vi "SIcamera_Manager.vi"() -> ()   [LabVIEW 2015]
uses:
  SI_Client_Subvis/Client Acquisition Mode Menu.ctl
  SI_Client_Subvis/Frame Mode 1.ctl
  W:/GSCS/Systems/SystemUtil/Command.ctl
  W:/GSCS/Systems/SIcamera_Control/SI_Client_Subvis/CameraStates.ctl
  W:/GSCS/Systems/Cam_Focus/CF_drivercontrol.ctl
  W:/GSCS/Log/LogItem.ctl
  SIcamera_Globals.vi
  W:/GSCS/Systems/SIcamera_Control/GPS_Drivers/GPS_Driver_Global.vi
  W:/GSCS/Systems/TCS_Link/TCSLINK_global.vi
  Instance          36 24Saved   SIcamera_Manager .vi
  W:/GSCS/GUI/GSP_GUI_global.vi
  W:/GSCS/Systems/SIcamera_Control/Apogee_Global.vi
  W:/GSCS/Systems/Cam_Focus/GSP_CF_Global.vi
panel:
  out "Focus Changed?":bool
  out "Current Lamp Percent":string
  out "Current Lamp":string
  out "Has Red switch been run":bool
  out "Readout left":dbl format="%<%M:%S>t"
  out "Exp time left":dbl format="%<%M:%S >t"
  out "Fe Ind":u16(ring)
  out "Quartz Ind":u16(ring)
  out "Ar Ind":u16(ring)
  out "Hg(Ar) Ind":u16(ring)
  out "Cu Ind":u16(ring)
  out "Ne Ind":u16(ring)
  out "Bulb Ind":u16(ring)
  in  "CCD Readout Speed":u8(ring)=3 items=["750 kHz, ATTN 0", "750 kHz, ATTN 2", "344 kHz, ATTN 0", "344 kHz, ATTN 3", "100 kHz, ATTN 2", "100 kHz, ATTN 3"]
  in  "CCD ROI Mode":u16(ring)=10 items=["Imaging, 1x1  "=0, "Imaging, 2x2"=1, "Imaging, 3x3"=2, "Spectroscopic, 1x1"=3, "Spectroscopic, 2x2"=4, "Spectroscopic, 3x3"=5, "MOS, 1x1"=11, "MOS, 2x2"=12, "MOS, 3x3"=13, "Slicer"=6, "Spectroscopic, ZZ Ceti"=14, "Slit Imaging/Alignment"=7, "MOS Imaging/Alignment"=10, "Set user-defined ROI..."=8, "Custom Mode"=9, "Custom from Script"=21]
  in  "MOS":bool
  in  "Lamp Cluster":T1
  in  "Calculate Offset":bool
  in  "sy1":dbl
  in  "sx1":dbl
  in  "oy1":dbl
  in  "ox1":dbl
  in  "N/S Offset":dbl min=0.0 max=420.0 step=0.15 format="%03.2f"
  in  "N/S Offset Choice":u16(ring) items=["North", "South"]
  in  "E/W Offset Choice":u8(ring) items=["East", "West"]
  in  "E/W Offset":dbl min=0.0 max=420.0 step=0.15 format="%03.2f"
  in  "Offset Telescope":bool
  in  "Systems Status & Control":enum32{"Camera", "General"}(tab)
  in  "Camera Color":string(combo)="Red"
  in  "Get Camera Status":bool
  out "CCD Temp.":string
  out "Vacuum Pressure":string
  in  "Reset TCP":bool
  out "Connection Status":bool
  in  "Reset Wavelength Angles System":bool
  in  "Proposal #":string
  in  "Observer Name":string
  in  "Show Images?":bool
  out "Image File Name":string="0001.image.fits"
  in  "Image #":i32=1 min=1 step=1 format="%04.0f"
  out "Current Status":string
  in  "Exp. Time (s)":dbl=1.0 min=0.25 step=1.0 format="%.2f"
  in  "RO Done":bool
  out "Exposure":u16(slide) scale=0.0..100.0
  out "Readout":u16(slide) caption="% Readout" scale=0.0..100.0
  in  "File Name Base":string="image"
  in  "Start Exposure":bool
  in  "Exposure Tab":T2(tab)=enum."Zero"
  in  "# Exposures":i32=1 min=1 step=1
  in  "Object Comments:":string
  in  "Object Name:":string
  in  "Dome Set Percent":i32 caption="%"
  out "Dome Ind":u16(ring)
  out "Dome Percent":i8=70 caption="%" min=0 max=100 step=1
  in  "Dome":bool
  out "Quartz Actual":i8 caption="%"
  in  "Quartz Intensity":i8=70 caption="%" min=0 max=100 step=1
  in  "# Flat Exposures":i32=1 min=1 step=1
  in  "Flat Name:":string
  in  "# Comp Exposures":i32=1 min=1 step=1
  in  "Comp Comments:":string
  in  "Comp Name:":string
  out "Dark Name:":string="DARK"
  in  "Dark Comments:":string
  in  "# Dark Exposures":i32=1 min=1 step=1
  out "Zero Name:":string="ZERO"
  in  "Zero Comments:":string
  in  "# Zero Exposures":i32=1 min=1 step=1
  in  "Step Size":dbl
  in  "Focus Start":dbl
  in  "# Focus Steps":dbl
  in  "Focus Name":string
  in  "Control references":T3
  in  "?":bool
  in  "ROIMODE":string
  in  "Exp. Time (s) 2":dbl=1.0 min=0.5 step=1.0 format="%.1f"
  in  "Save As":u16(ring)=1 items=["U16 FITS", "I16 FITS", "I32 FITS", "SGL FITS", "U16 TIFF", "I16 TIFF", "I32 TIFF", "SGL TIFF"]
  in  "Port Readout":u16(ring)=2 items=["4-port", "Port A", "Port B", "Port C", "Port D"]
  out "Current File Name":string
  out "TCP/IP ID":refnum<k5>
  out "CCD ROI":cluster{i32, i32, i32, i32, i32, i32}={0, 4096, 1, 0, 4096, 1}
  out "Open Shutter During Image?":bool=TRUE
  out "Readout Time":dbl
  in  "Thumbnail Setting":enum16{"Check Entire CCD", "Check Star Focus"}(ring)
  in  "Take Thumbnail":bool
  in  "Save":bool
  in  "Frames":i32=1 min=1 step=1
  in  "Frame Mode":T4 items=["Single Frame Buffer", "Multiple Frame Buffer"]
  out "Packet\nError code":i32
  out "Function #":u16
  in  "# to Average":u32=2 caption="of"
  out "Error out":errorcluster
  out "Acquiring":u32
  out "P Len":i32
  out "S Len":i32
  in  "Mode":u16(ring)=4 items=["Retrieve Image Buffer", "Acquire and transfer to client", "Acquire and hold in Server Image Buffer", "Acquire, transfer to client, and save to Server's disk", "Acquire, save to Server's disk, and hold in Server Image Buffer"]
  in  "Acq Mode":T5 caption="Acquisition Mode"
  in  "SHUTDOWN":bool
  in  "Script":T6={"Exposure Time"=0.0, "#Exposures"=1, "Current Exposure"=2, "Last Exposure Start Time"=92278252, "Exposure type"=1, "Obs parameters"={"Object Name"="", "Telescope"="SOAR 4.1m", "Instrument"="Goodman Spectrograph", "Comment"="", "INSTCONF"="", "CAMSWV"="", "CONSWV"="", "INSTSWV"="", "CAMERA"=""}, "System Pos Info"={"Grating#"=0, "Slit#"=0, "Primary Filter#"=0, "Secondary Filter#"=0, "Coll Position"=1000, "Camera Focus"=-396, "Camera Angle"=12.21, "Grating Angle"=20.740599999999997, "Coll Temp"=0.0, "Cam Temp"=0.0, "Camera Target"=12.21, "Grating Target"=20.740599999999997, "WAVMODE"="", "Slit hidden?"=FALSE}, "TCSInfo"={"Mount Az"=0.0, "Mount El"=0.0, "RA"="", "DEC"="", "Hour Angle"="", "Airmass"=0.0, "Focus"=0.0, "Rotator Angle"=0.0, "Rotator Location"="", "Dome Shutter"="", "Dome Az"=0.0, "Date"="", "UT Time"="", "Sidereal Time"="", "Position Angle"=0.0, "Seeing"=0.0, "OBSRA"="", "OBSDEC"="", "Position ADC"="", "Position ADC 2"="", "Bulb"=FALSE, "Ar"=FALSE, "Cu"=FALSE, "Dome"=FALSE, "Fe"=FALSE, "Hg(Ar)"=FALSE, "Ne"=FALSE, "Quartz"=FALSE, "Dome Percent"=0.0, "Quartz Percent"=0.0}, "Exposure Active?"=FALSE, "Component Names"={"Slit Name"="<NO MASK>", "F1_Name"="<NO FILTER>", "F2_Name"="<NO FILTER>", "Grating Name"="<NO GRATING>"}, "Other Info."={"CCD Read Noise"=3.99, "CCD Gain"=2.06, "OBSTYPE"="OBJECT", "OBSERVER"="", "Proposal #"="", "Equinox"=2000.0}, "Reduction Info."={"DISPAXIS"=1, "DETSIZE"="[1:4096,1:4096]", "CCDSUM"="1 1", "DETSEC"="[1:4096,1:4096]", "DATASEC"="[1:4096,1:4096]"}, "EnvironmentalInfo"={"Outside Temp"=0.0, "Wind Direction"=0.0, "Wind Speed"=0.0, "Pressure"=0.0, "Humidity"=0.0}} {"Other Info."."Equinox" format="%#.2f"; "Other Info."."CCD Gain" format="%#.2g"; "Other Info."."CCD Read Noise" format="%#.2g"; "Exposure type" items=["Dark", "Light"]}
  out "Camera Errors":errorcluster
  in  "CommandQ":string
  # "x"
  # "y"
  # "Save As"
  # "I16 FITS"
  # "Current Pixel Values:"
  # "\" to the"
  # "Port Readout"
  # "\" to the"
  # "Desired Pixel Values:"
  # "Port B"
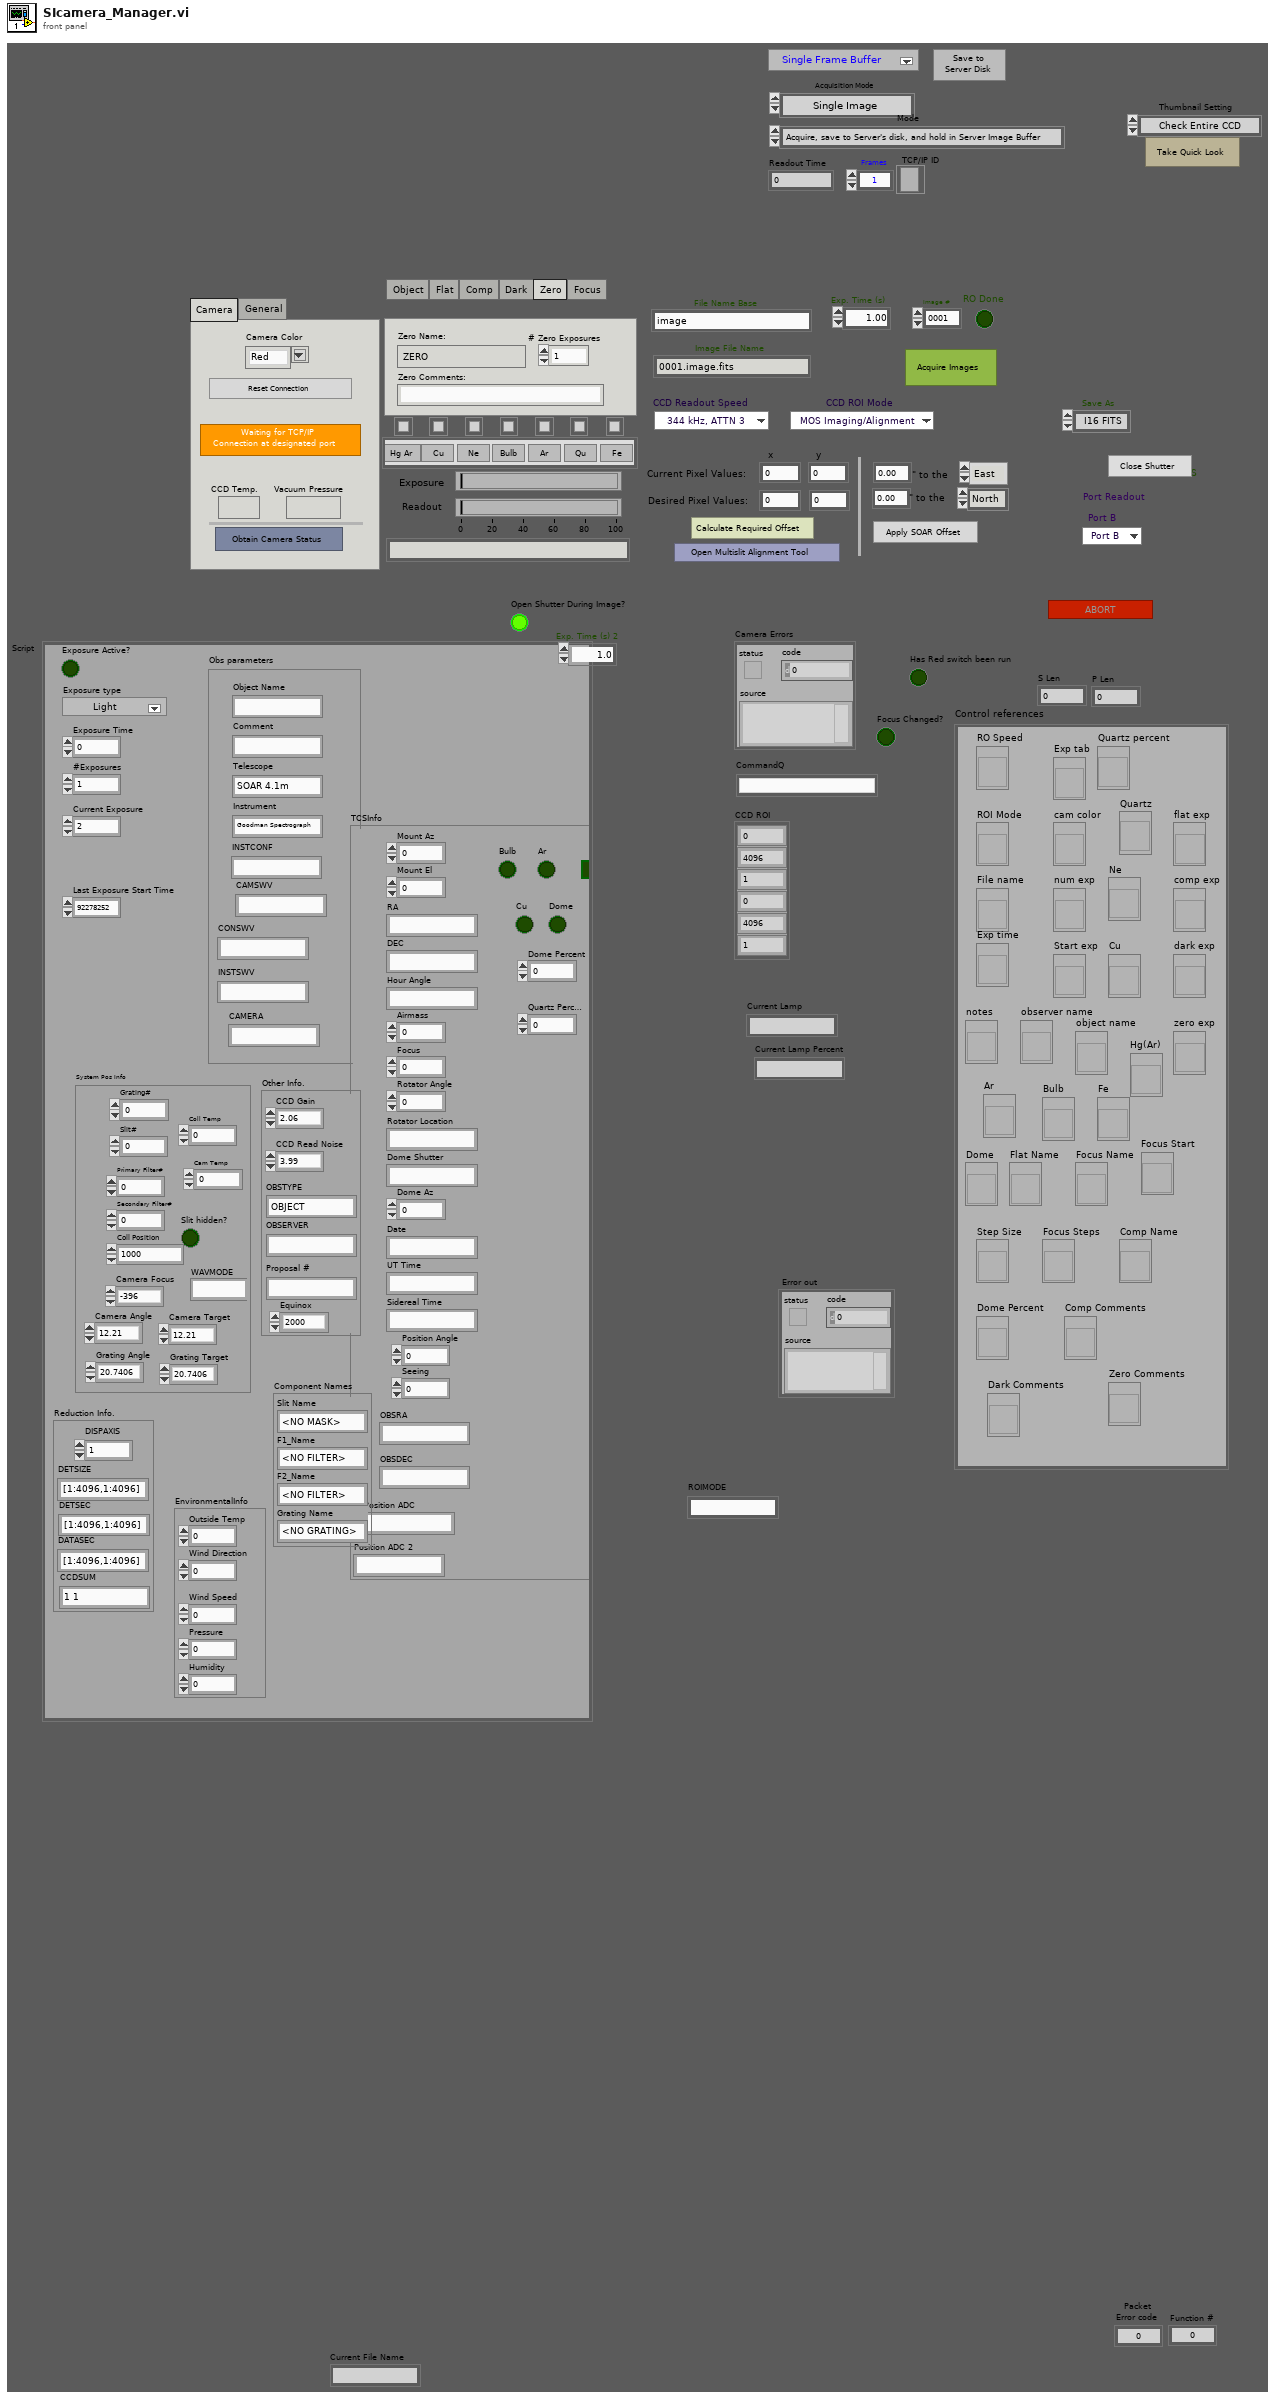
[diagram p1: front panel]
types:
  T1 = cluster{"Hg(Ar)":bool, "Cu":bool, "Ne":bool, "Ar":bool, "Quartz":bool, "Fe":bool, "Bulb":bool}
  T2 = enum32{"Object", "Flat", "Comp", "Dark", "Zero", "Focus"}
  T3 = cluster{"ROI Mode":refnum<vi>, "RO Speed":refnum<vi>, "File name":refnum<vi>, "Exp time":refnum<vi>, "Start exp":refnum<vi>, "num exp":refnum<vi>, "cam color":refnum<vi>, "Exp tab":refnum<vi>, "notes":refnum<vi>, "observer name":refnum<vi>, "object name":refnum<vi>, "Ar":refnum<vi>, "Bulb":refnum<vi>, "Fe":refnum<vi>, "Hg(Ar)":refnum<vi>, "Cu":refnum<vi>, "Ne":refnum<vi>, "Quartz":refnum<vi>, "Quartz percent":refnum<vi>, "flat exp":refnum<vi>, "comp exp":refnum<vi>, "dark exp":refnum<vi>, "zero exp":refnum<vi>, "Dome":refnum<vi>, "Flat Name":refnum<vi>, "Focus Name":refnum<vi>, "Focus Start":refnum<vi>, "Step Size":refnum<vi>, "Comp Name":refnum<vi>, "Comp Comments":refnum<vi>, "Focus Steps":refnum<vi>, "Dome Percent":refnum<vi>, "Dark Comments":refnum<vi>, "Zero Comments":refnum<vi>}
  T4 = typedef "Frame Mode 1.ctl" = i32
  T5 = typedef "Client Acquisition Mode Menu.ctl" = enum16{"Single Image", "Average Images", "Multiple Frames"}
  T6 = cluster{"Exposure Time":dbl, "#Exposures":i32, "Current Exposure":i32, "Last Exposure Start Time":u32, "Exposure type":i16, "Obs parameters":cluster{"Object Name":string, "Telescope":string, "Instrument":string, "Comment":string, "INSTCONF":string, "CAMSWV":string, "CONSWV":string, "INSTSWV":string, "CAMERA":string}, "System Pos Info":cluster{"Grating#":i32, "Slit#":i32, "Primary Filter#":i32, "Secondary Filter#":i32, "Coll Position":i32, "Camera Focus":i32, "Camera Angle":dbl, "Grating Angle":dbl, "Coll Temp":dbl, "Cam Temp":dbl, "Camera Target":dbl, "Grating Target":dbl, "WAVMODE":string, "Slit hidden?":bool}, "TCSInfo":cluster{"Mount Az":dbl, "Mount El":dbl, "RA":string, "DEC":string, "Hour Angle":string, "Airmass":dbl, "Focus":dbl, "Rotator Angle":dbl, "Rotator Location":string, "Dome Shutter":string, "Dome Az":dbl, "Date":string, "UT Time":string, "Sidereal Time":string, "Position Angle":dbl, "Seeing":dbl, "OBSRA":string, "OBSDEC":string, "Position ADC":string, "Position ADC 2":string, "Bulb":bool, "Ar":bool, "Cu":bool, "Dome":bool, "Fe":bool, "Hg(Ar)":bool, "Ne":bool, "Quartz":bool, "Dome Percent":dbl, "Quartz Percent":dbl}, "Exposure Active?":bool, "Component Names":cluster{"Slit Name":string, "F1_Name":string, "F2_Name":string, "Grating Name":string}, "Other Info.":cluster{"CCD Read Noise":dbl, "CCD Gain":dbl, "OBSTYPE":string, "OBSERVER":string, "Proposal #":string, "Equinox":dbl}, "Reduction Info.":cluster{"DISPAXIS":i8, "DETSIZE":string, "CCDSUM":string, "DETSEC":string, "DATASEC":string}, "EnvironmentalInfo":cluster{"Outside Temp":dbl, "Wind Direction":dbl, "Wind Speed":dbl, "Pressure":dbl, "Humidity":dbl}}
  T7 = typedef "Command.ctl" = cluster{"Command":string, "Parameter":string}
  T8 = cluster{"Object Name":string, "Telescope":string, "Instrument":string, "Comment":string, "\nINSTCONF":string, "CAMSWV":string, "CONSWV":string, "INSTSWV":string, "CAMERA":string}
  T9 = enum16{"POL (0)", "CPL (1)", "HLT (2)", "STP (3)", "RST (4)", "RVN (5)", "RPB (6)", "CLP (8)", "SDL (9)", "RUN (10)", "WRI (11)", "RRG (12)", "SPR (13)", "LPR (14)", "VMI (15)", "SSP (17)", "SSE (18)", "RIS (20)", "RIO (21)", "IMW (25)", "END (128)", "MAV (134)", "MRV (135)", "JRE (137)", "WCL (138)", "WCW (139)", "DLY (140)", "WDL (141)", "GCL (142)", "GOP (143)", "ZTG (144)", "ZTP (145)", "TTP (146)", "CME (147)", "CTC (148)", "TQL (149)", "AHC (150)", "ERL (151)", "OLP (152)", "WRP (154)", "IDT (155)", "LRP (156)", "VMP (159)", "RAV (160)", "RRV (161)", "JMP (162)", "JOI (162)", "CIS (163)", "CKS (164)", "CLC (165)", "KMC (167)", "MCT (168)", "FLC (169)", "EEM (170)", "DDB (171)", "DEM (171)", "PAC (172)", "ADL (173)", "BRT (174)", "MAT (176)", "MRT (177)", "RAT (178)", "RRT (179)", "SSD (180)", "KMR (181)", "KED (182)", "KDD (183)", "DIR (184)", "PRO (185)", "SIF (186)", "EDL (187)", "CIO (188)", "MDS (189)", "MDC (190)", "MDT (191)", "SEE (192)", "ARI (193)", "WBS (194)", "SCF (195)", "RSM (196)", "RLM (197)", "RSN (198)", "RLN (199)", "PCL (201)", "PCI (201)", "PRT (202)", "PRI (202)", "WBE (204)", "SOB (205)", "COB (206)", "ACR (207)", "PLR (208)", "CAI (211)", "LVT (212)", "OVT (213)", "MTT (214)", "CLC (215)", "PIM (216)", "VIM (217)", "TIM (218)", "AHM (219)", "SSL (221)", "TRU (222)", "RSD (223)", "EMT (225)", "DMT (226)", "EMD (227)", "DMD (228)", "HSM (229)", "AHD (230)", "PCM (231)", "PCG (232)", "XRV (233)", "XAV (234)", "XRT (235)", "XAT (236)", "GOC (237)", "JNA (238)", "JOR (239)", "PMC (240)", "PMV (241)", "PMX (242)", "DLC (243)", "SLC (244)", "PCP (245)", "ATR (248)", "PMO (249)", "JAN (250)", "EDH (251)", "DIF (252)", "IMS (253)", "IMQ (254)"}
  T10 = typedef "CameraStates.ctl" = enum16{"Ready", "Exposing", "Error"}
  T11 = typedef "CF_drivercontrol.ctl" = enum16{"Launch", "Move", "Set Piezos", "Flexure On", "Flexure Off", "Home", "Shutdown"}
  T12 = typedef "LogItem.ctl" = cluster{"error in (no error)":errorcluster, "Source":string, "Comment ":string}
  T13 = enum16{"Launch", "Log", "Open", "Close", "Shutdown"}
  T14 = cluster{"Serial Origin":i32, "Serial Length":i32, "Serial Binning":i32, "Parallel Origin":i32, "Parallel Length":i32, "Parallel Binning":i32}
  T15 = cluster{"Mount Az":dbl, "Mount El":dbl, "RA":string, "DEC":string, "Hour Angle":string, "Airmass":dbl, "Focus":dbl, "Rotator Angle":dbl, "Rotator Location":string, "Dome Shutter":string, "Dome Az":dbl, "Date":string, "UT Time":string, "Sidereal Time":string, "Position Angle":dbl, "Seeing":dbl, "OBSRA":string, "OBSDEC":string, "Position ADC":string, "Position ADC 2":string, "Bulb":bool, "Ar":bool, "Cu":bool, "Dome":bool, "Fe":bool, "Hg(Ar)":bool, "Ne":bool, "Quartz":bool, "Dome Percent":dbl, "Quartz Percent":dbl}
  T16 = cluster{"Grating#":i32, "Slit#":i32, "Primary Filter#":i32, "Secondary Filter#":i32, "Coll Position":i32, "Camera Focus":i32, "Camera Angle":dbl, "Grating Angle":dbl, "Coll Temp":dbl, "CF Temp\n":dbl, "Camera Target":dbl, "Grating Target":dbl, "WAVMODE":string, "Slit Hidden??":bool}
  T17 = cluster{"Slit Name":string, "F1_Name":string, "F2_Name":string, "Grating Name":string}
  T18 = cluster{"element":i32, "element":i32, "element":i32, "element":i32, "element":i32, "element":i32}
  T19 = cluster{"% Exp.":u16, "%Readout":u16, "Relative Pos.":u32, "Acquiring":i32}
  T20 = typedef "TCP-IP Image Packet.ctl" = cluster{"Image ID":u16, "Image Type":u16, "Serial Length":u16, "Parallel Length":u16, "# of Packets":u16, "Packet #":u16, "Offset":u32, "Image Bytes":u32, "Image Data $":string}
  T21 = cluster{"DISPAXIS":i8, "DETSIZE":string, "CCDSUM":string, "DETSEC":string, "DATASEC":string}
  T22 = cluster{"Object Name":string, "Telescope":string, "Instrument":string, "Comment":string, "INSTCONF":string, "CAMSWV":string, "CONSWV":string, "INSTSWV":string, "CAMERA":string}
  T23 = cluster{"CCD Read Noise":dbl, "CCD Gain":dbl, "OBSTYPE":string, "OBSERVER":string, "Proposal #":string, "Equinox":dbl}
  T24 = cluster{"Exp. Time (s)":dbl, "CCD Read Noise":dbl, "CCD Gain":dbl, "OBSTYPE":string, "OBSERVER":string, "Proposal #":string, "Equinox":dbl, "ROIMODE":string}
  T25 = cluster{"Outside Temp":dbl, "Wind Direction":dbl, "Wind Speed":dbl, "Pressure":dbl, "Humidity":dbl}
  T26 = typedef "ThreadStates.ctl" = enum16{"Waiting", "Scripting", "Uninitialized", "Error"}
  T27 = cluster{"Command":string, "Current File Name":string}
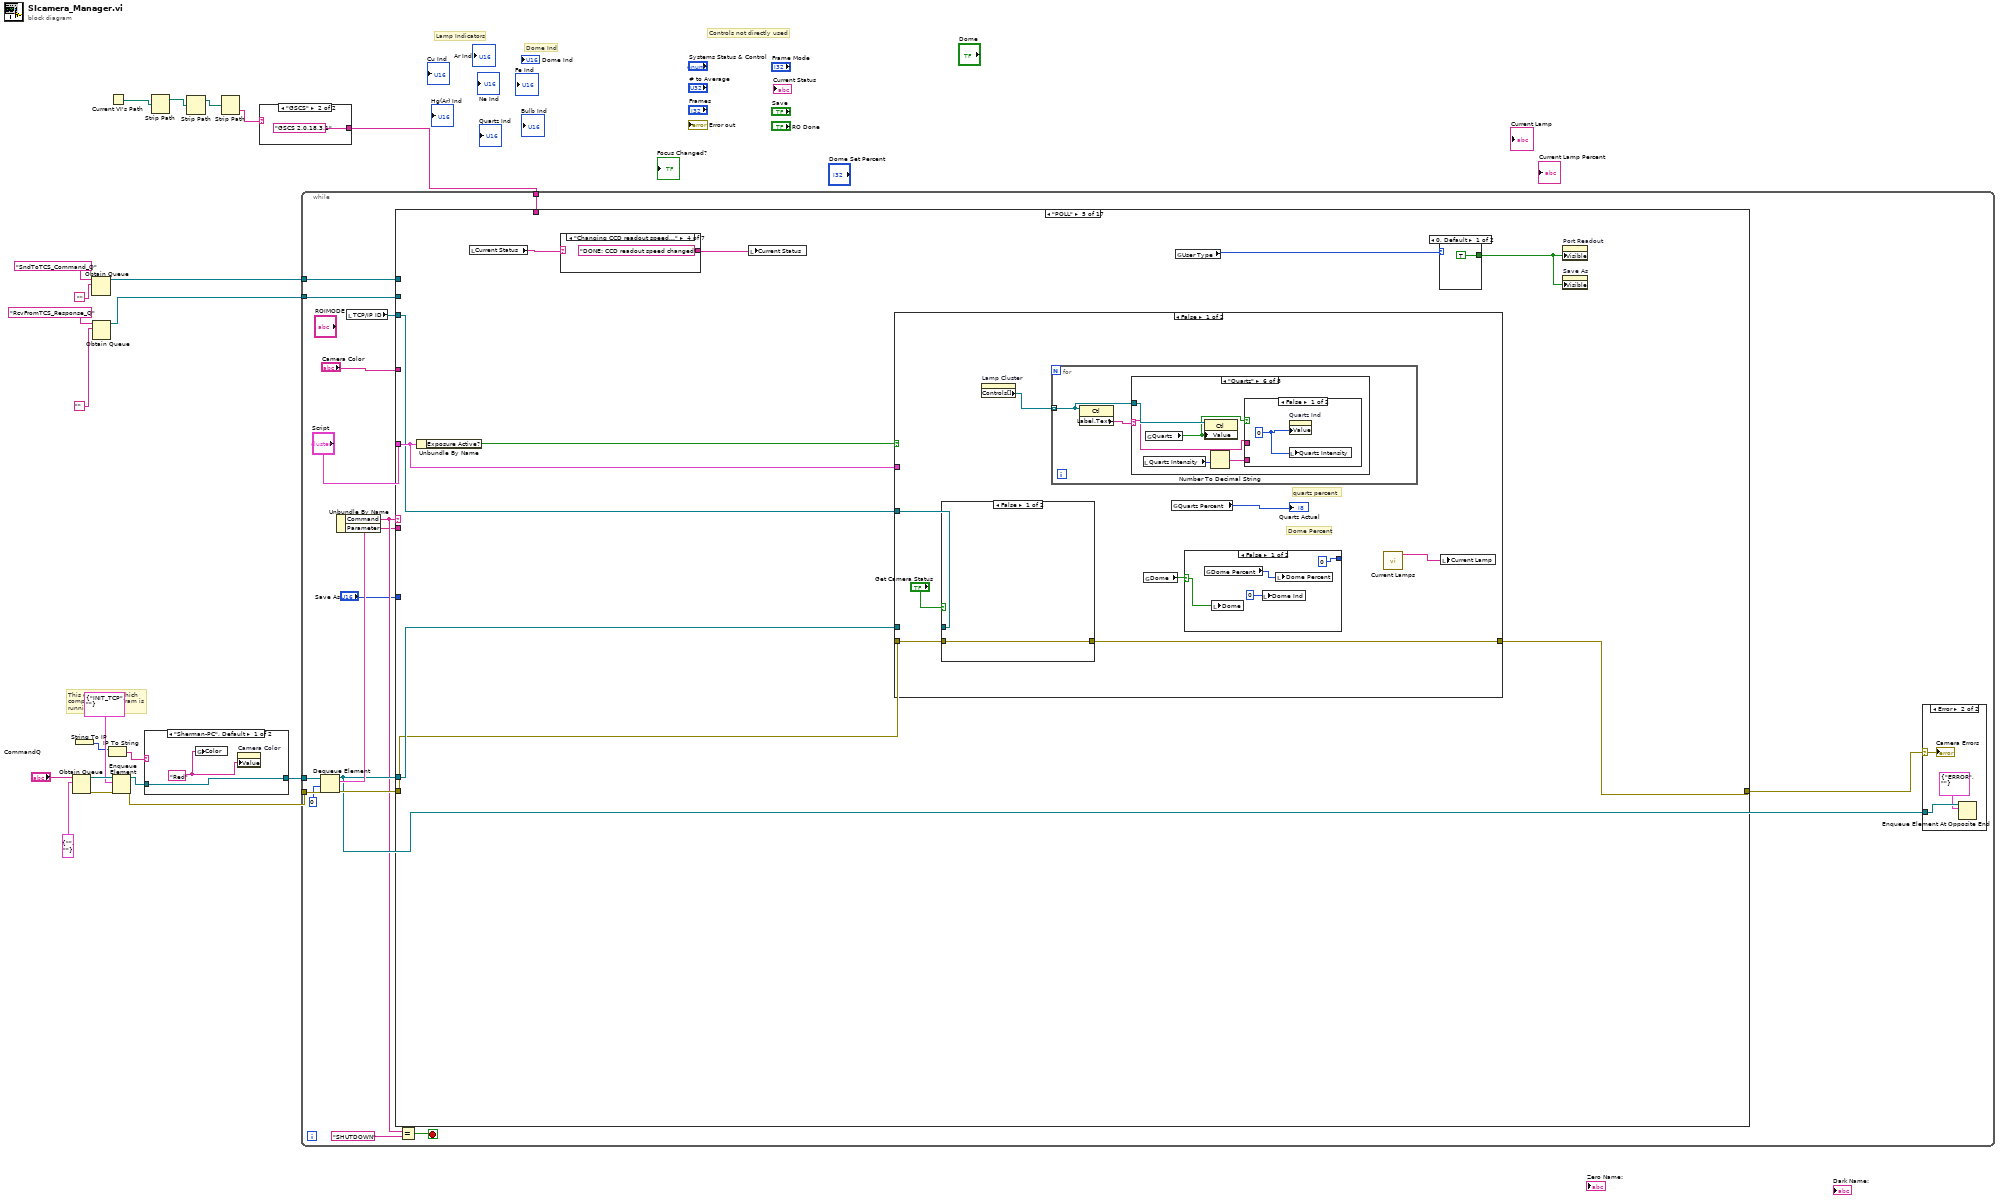
[diagram p0: block diagram]
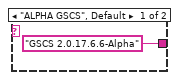
[diagram p2: hidden frame]
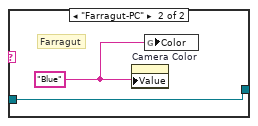
[diagram p3: hidden frame]
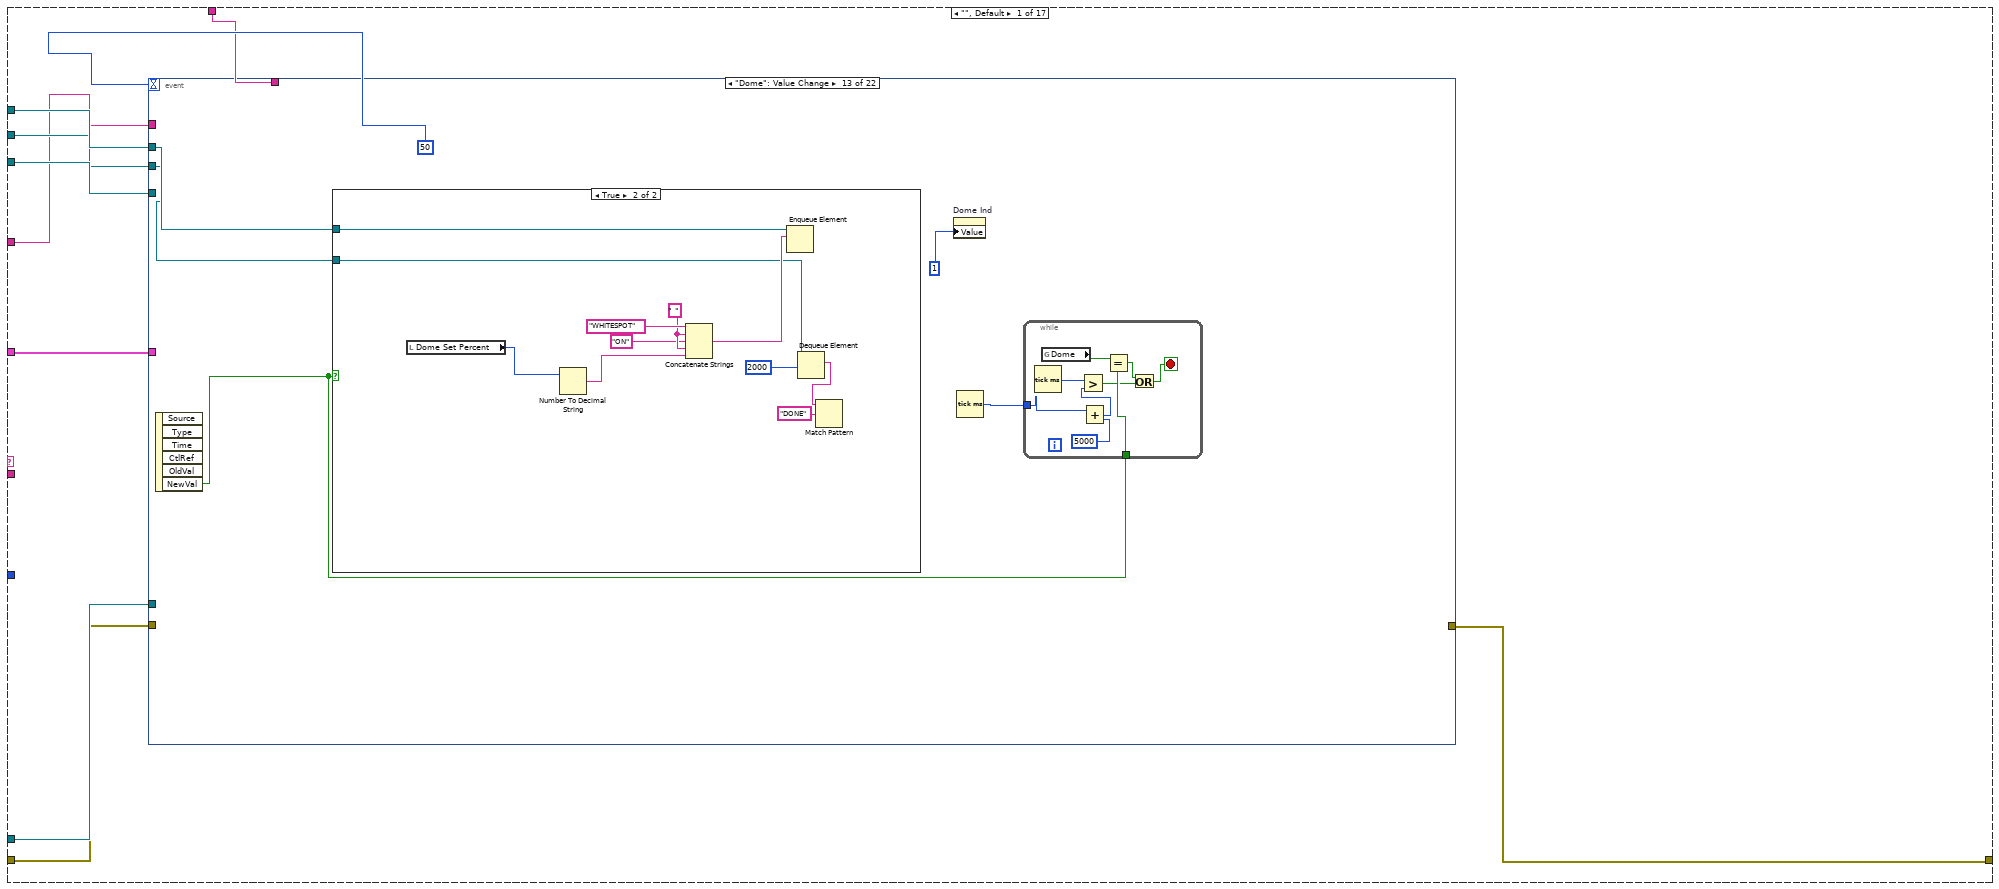
[diagram p5: hidden frame]
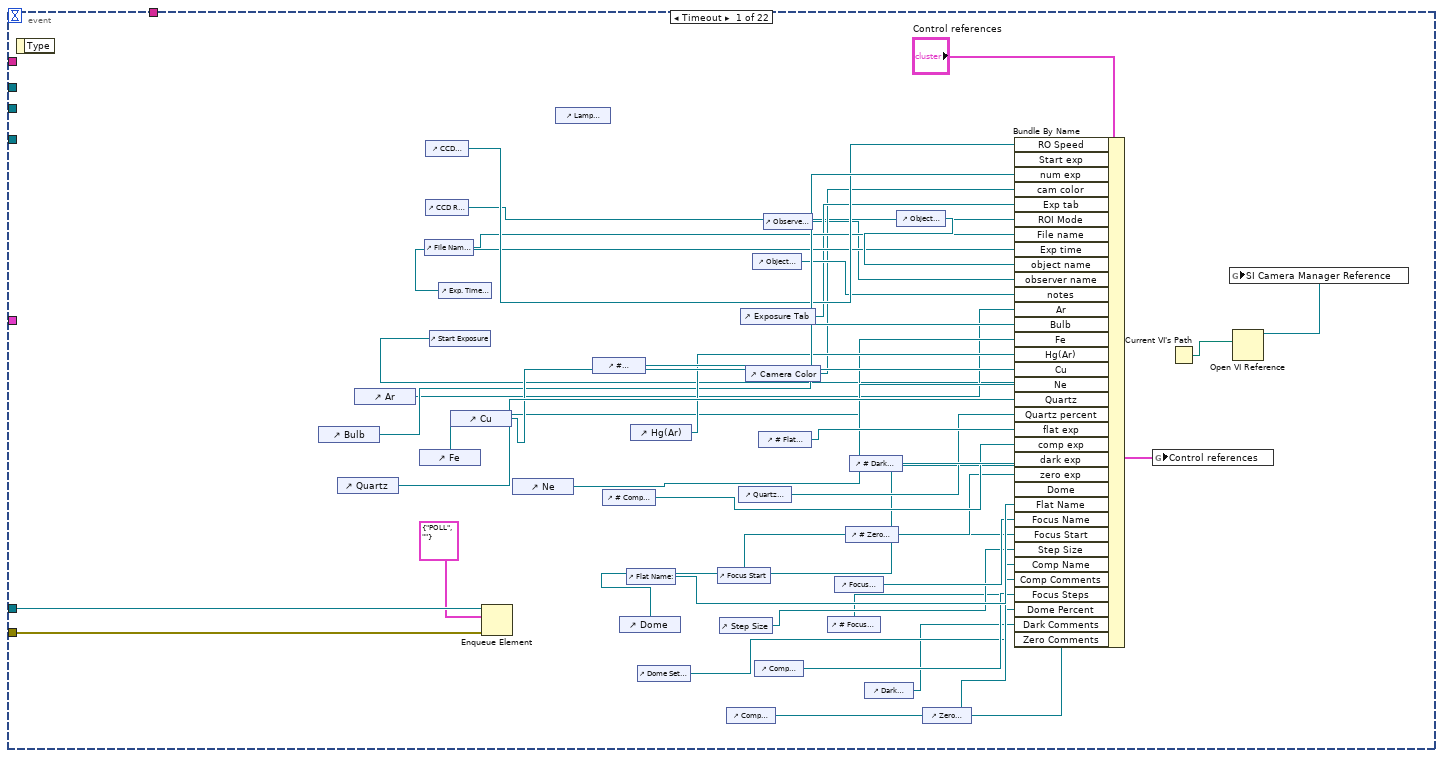
[diagram p6: hidden frame]
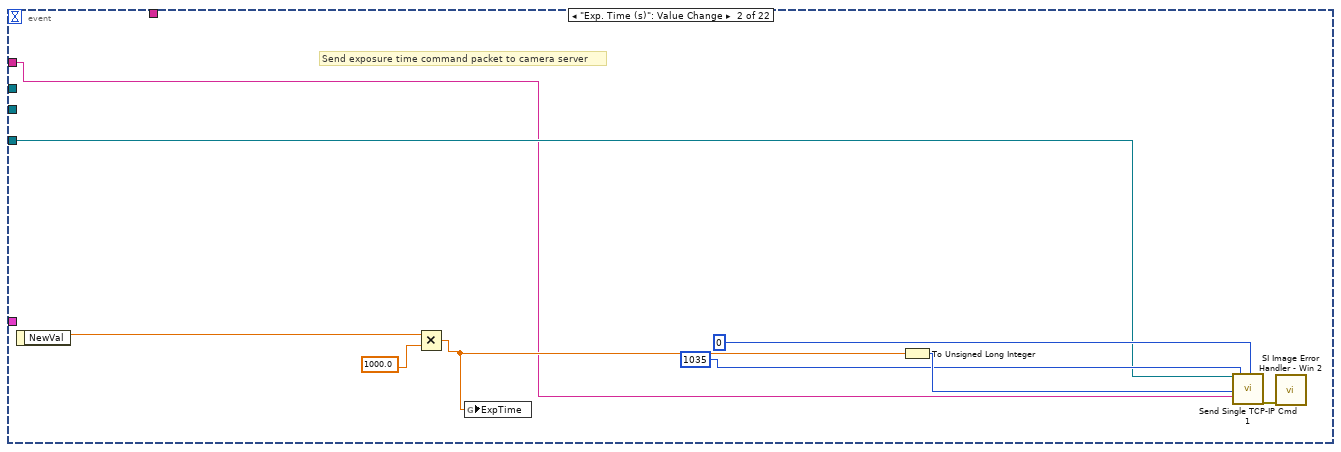
[diagram p7: hidden frame]
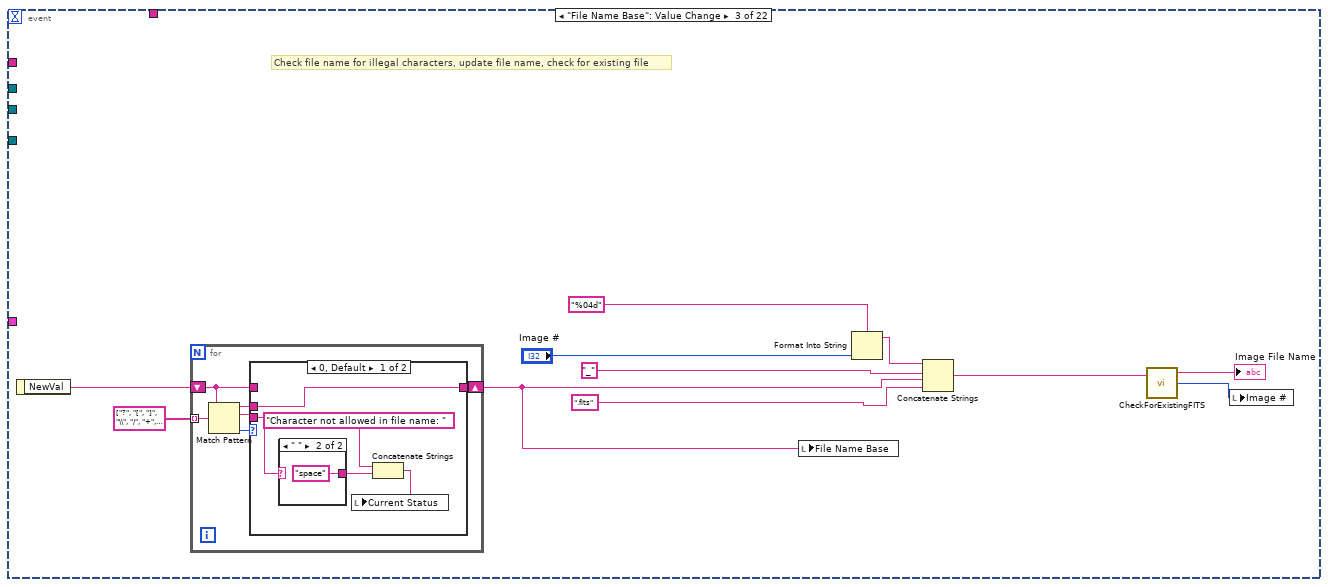
[diagram p8: hidden frame]
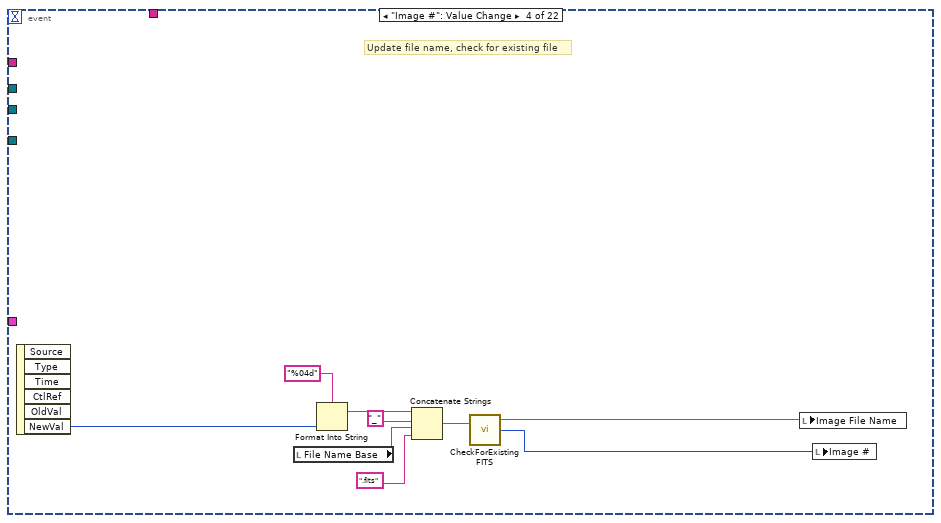
[diagram p11: hidden frame]
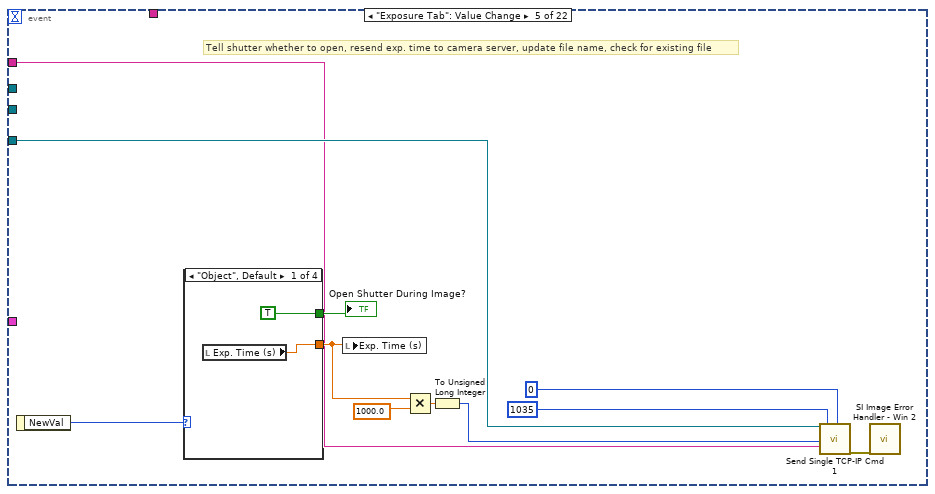
[diagram p12: hidden frame]
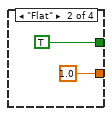
[diagram p13: hidden frame]
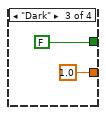
[diagram p14: hidden frame]
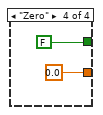
[diagram p15: hidden frame]
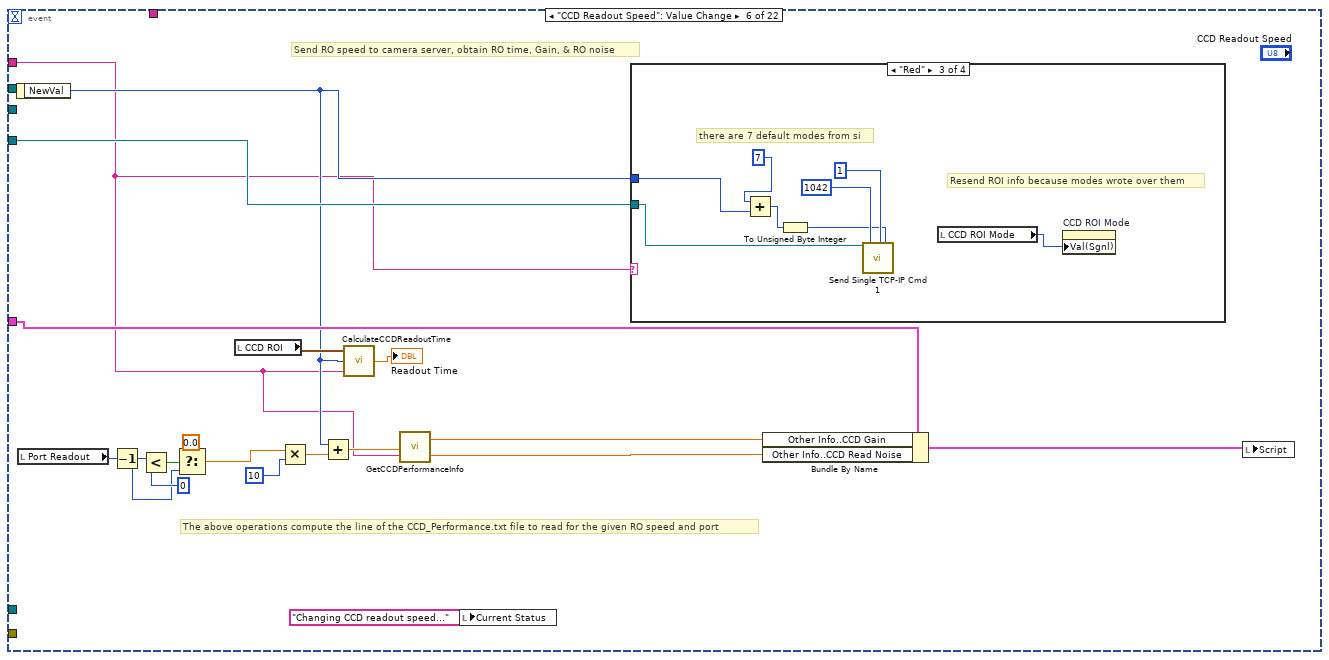
[diagram p16: hidden frame]
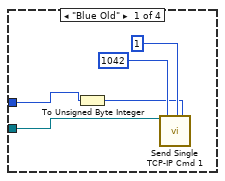
[diagram p17: hidden frame]
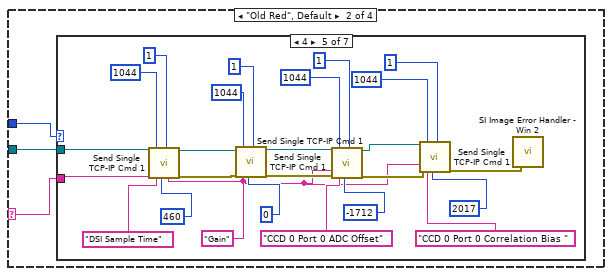
[diagram p18: hidden frame]
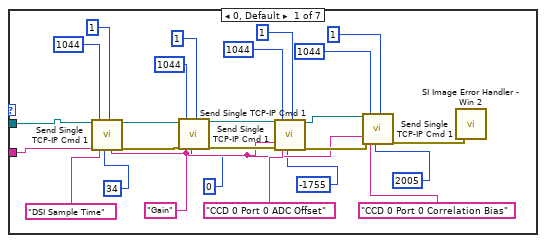
[diagram p19: hidden frame]
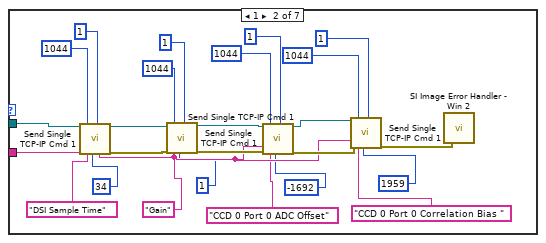
[diagram p20: hidden frame]
diagram:
  # "Lamp Indicators"
  # "Dome Ind"
  # "This determines which \ncomputer the program is \nrunning on"
  # "Controls not directly used"
  n1 = Obtain Queue(name (unnamed)="CommandQ", element data type=T7 {"Command"="", "Parameter"=""} ("Command")) -> (queue out=w18:refnum<queue>, error out=w19:errorcluster)  [unwired: 3 in, 1 out]
  n2 = String To IP() -> (0:w9:u32)  [unwired: 1 in]
  n3 = Obtain Queue(name (unnamed)="SndToTCS_Command_Q", element data type="") -> (queue out=w13:refnum<queue>)  [unwired: 3 in, 2 out]
  n4 = Obtain Queue(name (unnamed)="RcvFromTCS_Response_Q", element data type="") -> (queue out=w10:refnum<queue>)  [unwired: 3 in, 2 out]
  n5 = IP To String(2:w9) -> (0:w8:string)  [unwired: 1 in]
  n6 = Current VI's Path() -> (path=w5:path)
  n7 = Enqueue Element(queue=w18, element=T7 {"Command"="INIT_TCP", "Parameter"=""}, error in (no error)=w19) -> (queue out=w7:refnum<queue>, error out=w16:errorcluster)  [unwired: 1 in, 1 out]
  n8 = case shown="\"Sherman-PC\", Default" w8 {
    tunnel: w7 -> [w23 w25]
    tunnel: [w23 w25] -> w6
    frame "Sherman-PC", Default {
      w22 = "Red"
      n9 = global write "SIcamera_Globals.vi" "Color"(w22) -> ()
      n10 = property on="Camera Color" class="CmbBox"("Value"=w22) -> ()  [unwired: 2 in, 2 out]
    }
    frame "Farragut-PC" {
      w24 = "Blue"
      # "Farragut"
      n11 = property on="Camera Color" class="CmbBox"("Value"=w24) -> ()  [unwired: 2 in, 2 out]
      n12 = global write "SIcamera_Globals.vi" "Color"(w24) -> ()
    }
  }
  n13 = Strip Path(path=w5) -> (stripped path=w4:path)  [unwired: 1 out]
  n14 = Strip Path(path=w4) -> (stripped path=w3:path)  [unwired: 1 out]
  n15 = Strip Path(path=w3) -> (name=w2:string)  [unwired: 1 out]
  n16 = case shown="\"GSCS\"" w2 {
    tunnel: ["GSCS 2.0.17.6.6-Alpha" "GSCS 2.0.18.3.1"] -> w1
    frame "ALPHA GSCS", Default {
    }
    frame "GSCS" {
    }
  }
  n17 = while {
    tunnel: w6 -> [w45]
    tunnel: w16 -> [w44]
    tunnel: w13 -> [w34]
    tunnel: w10 -> [w33]
    tunnel: w1 -> [w29]
    stop <- w37 stop-if-true
    n18 = Dequeue Element(queue=w45, timeout in ms (-1)=0, error in (no error)=w44) -> (queue out=w39:refnum<queue>, element=w42:T7, error out=w40:errorcluster)  [unwired: 1 out]
    n19 = Unbundle By Name(w42) -> ("Command"=w36:string, "Parameter"=w32:string)
    n20 = local read "TCP/IP ID"() -> (w35:refnum<k5>)
    n21 = case shown="\"POLL\"" w36 {
      tunnel: w39 -> [w58 _ w1597 _ w1677 w1832 _ _ _ w2156 _ _ _ _ _ w2378 w2416]
      tunnel: w40 -> [w57 w1581 w1592 w1641 w1675 w1846 w2094 w2108 w2117 w2152 w2257 w2291 w2306 w2320 w2376 _ w2415]
      tunnel: [w55 w1581 errorcluster {"status"=FALSE, "code"=0, "source"=""} ("error out") w1627 w1676 w1846 w2068 w2108 w2110 w2135 w2256 w2287 w2306 w2315 w2376 errorcluster {"status"=FALSE, "code"=0, "source"=""} ("error out") w2412] -> w38
      tunnel: "Script" -> [w56 _ _ _ w1678 w1834 w2097 _ w2116 w2145 _ w2285 _ _ _ _ _]
      tunnel: w35 -> [w53 _ _ w1645 w1674 w1833 _ _ _ w2149 _ w2295 _ w2316 _ _ w2410]
      tunnel: w34 -> [w52 _ _ _ _ _ _ _ _ _ _ _ _ _ _ _ w2409]
      tunnel: w33 -> [w51 _ _ _ _ _ _ _ _ _ _ _ _ _ _ _ w2408]
      tunnel: w32 -> [_ w1584 _ _ _ _ _ _ _ _ _ _ _ _ _ _ _]
      tunnel: "Camera Color" -> [w50 _ w1589 w1625 _ w1831 _ _ _ w2136 w2255 w2294 _ w2314 _ _ _]
      tunnel: "Save As" -> [_ _ _ _ _ _ _ _ _ w2137 _ w2290 _ _ _ _ _]
      tunnel: w29 -> [w49 _ _ _ _ _ _ _ _ _ _ _ _ _ _ _ _]
      frame "", Default {
        n22 = event shown="[12] \"Dome\": Value Change" {
          selector: _ -> [_ _ _ _ _ _ _ _ _ _ _ _ _ _ _ _ _ _ _ _ _ _]
          dyn-events: _ -> [_ _ _ _ _ _ _ _ _ _ _ _ _ _ _ _ _ _ _ _ _ _]
          timeout: 50 -> [_ _ _ _ _ _ _ _ _ _ _ _ _ _ _ _ _ _ _ _ _ _]
          tunnel: w58 -> [w99 _ _ _ _ _ _ _ _ _ _ _ _ _ _ _ _ _ _ _ w1568 w1573]
          tunnel: w57 -> [w98 _ _ _ _ _ w585 _ _ _ _ _ _ w1373 w1401 _ _ _ _ _ w1567 w1572]
          tunnel: w56 -> [_ _ _ _ _ w176 w566 w1098 _ _ _ _ _ _ w1402 _ w1488 _ _ _ _ _]
          tunnel: [_ _ _ _ _ _ w585 _ _ _ _ _ _ w1372 w1401 _ _ _ _ _ w1563 w1571] -> w55
          tunnel: w53 -> [_ w103 _ _ w146 w180 w571 w1107 _ _ _ _ _ _ _ _ w1489 _ _ _ w1569 _]
          tunnel: w52 -> [_ _ _ _ _ _ _ _ _ w1142 w1281 w1311 w1336 _ _ _ _ _ _ w1543 _ _]
          tunnel: w51 -> [_ _ _ _ _ _ _ _ _ w1141 w1280 w1310 w1335 _ _ _ _ _ _ w1542 _ _]
          tunnel: w50 -> [_ w100 _ _ w143 w162 w557 w1086 _ _ _ _ _ _ w1387 _ w1481 _ _ _ _ _]
          tunnel: w49 -> [_ _ _ _ _ _ _ _ _ _ _ _ _ _ w1389 _ _ _ _ _ _ _]
          event Timeout {
            n23 = event-data() -> ()  [unwired: 1 in, 1 out]
            n24 = control-ref of="Bulb"() -> (w83:refnum<vi>)
            n25 = control-ref of="Quartz"() -> (w88:refnum<vi>)
            n26 = control-ref of="Ar"() -> (w82:refnum<vi>)
            n27 = control-ref of="Fe"() -> (w84:refnum<vi>)
            n28 = control-ref of="File Name Base"() -> (w77:refnum<vi>)
            n29 = control-ref of="CCD Readout Speed"() -> (w95:refnum<vi>)
            n30 = control-ref of="CCD ROI Mode"() -> (w70:refnum<vi>)
            n31 = control-ref of="Start Exposure"() -> (w79:refnum<vi>)
            n32 = control-ref of="Exp. Time (s)"() -> (w78:refnum<vi>)
            n33 = control-ref of="Cu"() -> (w86:refnum<vi>)
            n34 = Enqueue Element(queue=w99, element=T7 {"Command"="POLL", "Parameter"=""}, error in (no error)=w98) -> ()  [unwired: 1 in, 3 out]
            n35 = control-ref of="Ne"() -> (w87:refnum<vi>)
            n36 = control-ref of="Lamp Cluster"() -> ()  [unwired: 1 out]
            n37 = control-ref of="# Exposures"() -> (w96:refnum<vi>)
            n38 = control-ref of="# Comp Exposures"() -> (w91:refnum<vi>)
            n39 = control-ref of="Dome"() -> (w69:refnum<vi>)
            n40 = control-ref of="Flat Name:"() -> (w68:refnum<vi>)
            n41 = control-ref of="Hg(Ar)"() -> (w85:refnum<vi>)
            n42 = control-ref of="Dome Set Percent"() -> (w61:refnum<vi>)
            n43 = control-ref of="Focus Start"() -> (w66:refnum<vi>)
            n44 = control-ref of="Step Size"() -> (w65:refnum<vi>)
            n45 = control-ref of="Comp Comments:"() -> (w63:refnum<vi>)
            n46 = control-ref of="Quartz Intensity"() -> (w89:refnum<vi>)
            n47 = control-ref of="Exposure Tab"() -> (w76:refnum<vi>)
            n48 = control-ref of="Camera Color"() -> (w75:refnum<vi>)
            n49 = control-ref of="Object Comments:"() -> (w81:refnum<vi>)
            n50 = control-ref of="Comp Name:"() -> (w64:refnum<vi>)
            n51 = control-ref of="# Flat Exposures"() -> (w90:refnum<vi>)
            n52 = control-ref of="Observer Name"() -> (w71:refnum<vi>)
            n53 = control-ref of="# Focus Steps"() -> (w62:refnum<vi>)
            n54 = control-ref of="Focus Name"() -> (w67:refnum<vi>)
            n55 = control-ref of="# Zero Exposures"() -> (w73:refnum<vi>)
            n56 = control-ref of="# Dark Exposures"() -> (w92:refnum<vi>)
            n57 = control-ref of="Dark Comments:"() -> (w60:refnum<vi>)
            n58 = control-ref of="Object Name:"() -> (w94:refnum<vi>)
            n59 = control-ref of="Zero Comments:"() -> (w59:refnum<vi>)
            n60 = Bundle By Name(cluster="Control references", "RO Speed"=w95, "Start exp"=w79, "num exp"=w96, "cam color"=w75, "Exp tab"=w76, "ROI Mode"=w70, "File name"=w77, "Exp time"=w78, "object name"=w94, "observer name"=w71, "notes"=w81, "Ar"=w82, "Bulb"=w83, "Fe"=w84, "Hg(Ar)"=w85, "Cu"=w86, "Ne"=w87, "Quartz"=w88, "Quartz percent"=w89, "flat exp"=w90, "comp exp"=w91, "dark exp"=w92, "zero exp"=w73, "Dome"=w69, "Flat Name"=w68, "Focus Name"=w67, "Focus Start"=w66, "Step Size"=w65, "Comp Name"=w64, "Comp Comments"=w63, "Focus Steps"=w62, "Dome Percent"=w61, "Dark Comments"=w60, "Zero Comments"=w59) -> (w80:T3)
            n61 = global write "SIcamera_Globals.vi" "Control references"(w80) -> ()
            n62 = Current VI's Path() -> (path=w93:path)
            n63 = Open VI Reference(vi path=w93) -> (vi reference=w72:refnum<vi>)  [unwired: 5 in, 1 out]
            n64 = global write "SIcamera_Globals.vi" "SI Camera Manager Reference"(w72) -> ()
          }
          event "Exp. Time (s)": Value Change {
            # "Send exposure time command packet to camera server"
            n65 = event-data() -> ("NewVal"=w101:dbl)  [unwired: 1 in]
            n66 = Multiply(x=w101, y=1000.0) -> (x*y=w102:dbl)
            n67 = global write "GPS_Driver_Global.vi" "ExpTime"(w102) -> ()
            n68 = To Unsigned Long Integer(number=w102) -> (unsigned 32bit integer=w108:u32)
            n69 = call "Send Single TCP-IP Cmd 1.vi"("TCP/IP ID"=w103, "Exposure Time (ms)"=w108, "Camera Color"=w100, "Function #"=u16 1035, "Camera ID"=u8 0) -> ("Error Out"=w106:errorcluster)  [unwired: 11 in, 3 out]
            n70 = call "SI Image Error Handler - Win 2.vi"("error in (no error)"=w106) -> ()  [unwired: 4 in, 1 out]
          }
          event "File Name Base": Value Change {
            # "Check file name for illegal characters, update file name, check for existing file"
            n71 = event-data() -> ("NewVal"=w110:string)  [unwired: 1 in]
            n72 = for {
              tunnel: string[] ["?", "[", "]", "\\", "/", "=", "+", "<", ">", ":", ";", "\"", ",", " ", "*"] -> [w125] mode=indexing
              shift-right: [w121] -> w109
              shift-left: w110 -> [w122]
              n73 = Match Pattern(string=w122, regular expression=w125) -> (before substring=w123:string, match substring=w120:string, offset past match=w124:i32)  [unwired: 1 in, 1 out]
              n74 = case shown="0, Default" w124 {
                tunnel: w123 -> [w130 _]
                tunnel: w122 -> [_ w133]
                tunnel: [w130 w133] -> w121
                tunnel: w120 -> [w128 _]
                frame 0, Default {
                  n75 = case shown="\" \"" w128 {
                    selector: w128 -> [w131 _]
                    tunnel: [w131 "space"] -> w127
                    frame Default {
                    }
                    frame " " {
                    }
                  }
                  n76 = Concatenate Strings("Character not allowed in file name: " ("string"), w127) -> (w126:string)
                  n77 = local write "Current Status"(w126) -> ()
                }
                frame -1 {
                }
              }
            }
            n78 = local write "File Name Base"(w109) -> ()
            n79 = Format Into String(format string="%04d", "Image #") -> (resulting string=w117:string)  [unwired: 2 in, 1 out]
            n80 = Concatenate Strings(w117, "_" ("string"), w109, ".fits" ("string")) -> (w113:string)
            n81 = call "CheckForExistingFITS.vi"("Filename"=w113) -> ("New Filename"=→"Image File Name":string, "New Exposure #"=w114:i32)  [unwired: 1 in, 1 out]
            n82 = local write "Image #"(w114) -> ()
          }
          event "Image #": Value Change {
            # "Update file name, check for existing file"
            n83 = event-data() -> ("NewVal"=w141:i32)  [unwired: 1 in, 5 out]
            n84 = local read "File Name Base"() -> (w138:string)
            n85 = Format Into String(format string="%04d", w141) -> (resulting string=w140:string)  [unwired: 2 in, 1 out]
            n86 = Concatenate Strings(w140, "_" ("string"), w138, ".fits" ("string")) -> (w136:string)
            n87 = call "CheckForExistingFITS.vi"("Filename"=w136) -> ("New Filename"=w135:string, "New Exposure #"=w134:i32)  [unwired: 1 in, 1 out]
            n88 = local write "Image File Name"(w135) -> ()
            n89 = local write "Image #"(w134) -> ()
          }
          event "Exposure Tab": Value Change {
            # "Tell shutter whether to open, resend exp. time to camera server, update file name, check for existing file"
            n90 = event-data() -> ("NewVal"=w153:T2)  [unwired: 1 in]
            n91 = case shown="\"Object\", Default" w153 {
              tunnel: [w154 1.0 ("Exposure Time") 1.0 ("Exposure Time") 0.0 ("Exposure Time")] -> w145
              tunnel: [TRUE ("Open Shutter During Image?") TRUE ("Open Shutter During Image?") FALSE ("Open Shutter During Image?") FALSE ("Open Shutter During Image?")] -> w144
              frame "Object", Default {
                n92 = local read "Exp. Time (s)"() -> (w154:dbl)
              }
              frame "Flat" {
              }
              frame "Dark" {
              }
              frame "Zero" {
              }
            }
            "Open Shutter During Image?" <- w144
            n93 = local write "Exp. Time (s)"(w145) -> ()
            n94 = Multiply(x=w145, y=1000.0) -> (x*y=w151:dbl)
            n95 = To Unsigned Long Integer(number=w151) -> (unsigned 32bit integer=w152:u32)
            n96 = call "Send Single TCP-IP Cmd 1.vi"("TCP/IP ID"=w146, "Exposure Time (ms)"=w152, "Camera Color"=w143, "Function #"=u16 1035, "Camera ID"=u8 0) -> ("Error Out"=w149:errorcluster)  [unwired: 11 in, 3 out]
            n97 = call "SI Image Error Handler - Win 2.vi"("error in (no error)"=w149) -> ()  [unwired: 4 in, 1 out]
          }
          event "CCD Readout Speed": Value Change {
            # "The above operations compute the line of the CCD_Performance.txt file to read for the given RO speed and port"
            # "Send RO speed to camera server, obtain RO time, Gain, & RO noise"
            n98 = event-data() -> ("NewVal"=w163:u8)  [unwired: 1 in]
            n99 = local read "Port Readout"() -> (w166:u16)
            n100 = Decrement(x=w166) -> (x-1=w164:u16)
            n101 = Less?(x=w164, y=u16 0) -> (x < y?=w168:bool)
            n102 = Select(t=0.0, s=w168, f=w164) -> (s? t:f=w165:dbl)
            n103 = local read "CCD ROI"() -> (w179:cluster{i32, i32, i32, i32, i32, i32})
            n104 = Multiply(x=w165, y=u16 10) -> (x*y=w170:dbl)
            n105 = Add(x=w163, y=w170) -> (x+y=w171:dbl)
            n106 = call "CalculateCCDReadoutTime.vi"("Color"=w162, "Readout Speed"=w163, "CCD ROI"=w179) -> ("Readout Time"=→"Readout Time":dbl)
            n107 = call "GetCCDPerformanceInfo.vi"("Color"=w162, "RO Speed Mode"=w171) -> ("Read Noise"=w174:dbl, "Gain"=w175:dbl)
            n108 = local write "Current Status"("Changing CCD readout speed..." ("Current Status")) -> ()
            n109 = case shown="\"Red\"" w162 {
              selector: w162 -> [_ w186 _ w377]
              tunnel: w180 -> [w183 w188 w371 w376]
              tunnel: w163 -> [w182 w187 w370 w375]
              frame "Blue Old" {
                n110 = To Unsigned Byte Integer(number=w182) -> (unsigned 8bit integer=w181:u8)
                n111 = call "Send Single TCP-IP Cmd 1.vi"("TCP/IP ID"=w183, "Function #"=u16 1042, "Camera ID"=u8 1, "Acq. Mode/Type/Frame Mode/RO Mode #"=w181) -> ()  [unwired: 12 in, 4 out]
              }
              frame "Old Red", Default {
                n112 = case shown="4" w187 {
                  tunnel: w188 -> [w196 w236 w243 w268 w292 w318 w348]
                  tunnel: w186 -> [w197 w225 w239 w267 w293 w314 w349]
                  frame 0, Default {
                    n113 = call "Send Single TCP-IP Cmd 1.vi"("TCP/IP ID"=w196, "Camera Color"=w197, "Function #"=u16 1044, "File Name"="DSI Sample Time", "Parameter Value"=34, "Camera ID"=u8 1) -> ("TCP/IP ID Out"=w191:refnum<k5>, "Error Out"=w211:errorcluster)  [unwired: 10 in, 2 out]
                    n114 = call "Send Single TCP-IP Cmd 1.vi"("TCP/IP ID"=w191, "Camera Color"=w197, "Error In"=w211, "Function #"=u16 1044, "File Name"="Gain", "Parameter Value"=0, "Camera ID"=u8 1) -> ("TCP/IP ID Out"=w190:refnum<k5>, "Error Out"=w210:errorcluster)  [unwired: 9 in, 2 out]
                    n115 = call "Send Single TCP-IP Cmd 1.vi"("TCP/IP ID"=w190, "Camera Color"=w197, "Error In"=w210, "Function #"=u16 1044, "File Name"="CCD 0 Port 0 ADC Offset", "Parameter Value"=-1755, "Camera ID"=u8 1) -> ("TCP/IP ID Out"=w189:refnum<k5>, "Error Out"=w209:errorcluster)  [unwired: 9 in, 2 out]
                    n116 = call "Send Single TCP-IP Cmd 1.vi"("TCP/IP ID"=w189, "Camera Color"=w197, "Error In"=w209, "Function #"=u16 1044, "File Name"="CCD 0 Port 0 Correlation Bias", "Parameter Value"=2005, "Camera ID"=u8 1) -> ("Error Out"=w208:errorcluster)  [unwired: 9 in, 3 out]
                    n117 = call "SI Image Error Handler - Win 2.vi"("error in (no error)"=w208) -> ()  [unwired: 4 in, 1 out]
                  }
                  frame 1 {
                    n118 = call "Send Single TCP-IP Cmd 1.vi"("TCP/IP ID"=w236, "Camera Color"=w225, "Function #"=u16 1044, "File Name"="DSI Sample Time", "Parameter Value"=34, "Camera ID"=u8 1) -> ("TCP/IP ID Out"=w220:refnum<k5>, "Error Out"=w235:errorcluster)  [unwired: 10 in, 2 out]
                    n119 = call "Send Single TCP-IP Cmd 1.vi"("TCP/IP ID"=w220, "Camera Color"=w225, "Error In"=w235, "Function #"=u16 1044, "File Name"="Gain", "Parameter Value"=1, "Camera ID"=u8 1) -> ("TCP/IP ID Out"=w219:refnum<k5>, "Error Out"=w234:errorcluster)  [unwired: 9 in, 2 out]
                    n120 = call "Send Single TCP-IP Cmd 1.vi"("TCP/IP ID"=w219, "Camera Color"=w225, "Error In"=w234, "Function #"=u16 1044, "File Name"="CCD 0 Port 0 ADC Offset", "Parameter Value"=-1692, "Camera ID"=u8 1) -> ("TCP/IP ID Out"=w218:refnum<k5>, "Error Out"=w233:errorcluster)  [unwired: 9 in, 2 out]
                    n121 = call "Send Single TCP-IP Cmd 1.vi"("TCP/IP ID"=w218, "Camera Color"=w225, "Error In"=w233, "Function #"=u16 1044, "File Name"="CCD 0 Port 0 Correlation Bias ", "Parameter Value"=1959, "Camera ID"=u8 1) -> ("Error Out"=w232:errorcluster)  [unwired: 9 in, 3 out]
                    n122 = call "SI Image Error Handler - Win 2.vi"("error in (no error)"=w232) -> ()  [unwired: 4 in, 1 out]
                  }
                  frame 2 {
                    n123 = call "Send Single TCP-IP Cmd 1.vi"("TCP/IP ID"=w243, "Camera Color"=w239, "Function #"=u16 1044, "File Name"="DSI Sample Time", "Parameter Value"=113, "Camera ID"=u8 1) -> ("TCP/IP ID Out"=w242:refnum<k5>, "Error Out"=w261:errorcluster)  [unwired: 10 in, 2 out]
                    n124 = call "Send Single TCP-IP Cmd 1.vi"("TCP/IP ID"=w242, "Camera Color"=w239, "Error In"=w261, "Function #"=u16 1044, "File Name"="Gain", "Parameter Value"=0, "Camera ID"=u8 1) -> ("TCP/IP ID Out"=w241:refnum<k5>, "Error Out"=w260:errorcluster)  [unwired: 9 in, 2 out]
                    n125 = call "Send Single TCP-IP Cmd 1.vi"("TCP/IP ID"=w241, "Camera Color"=w239, "Error In"=w260, "Function #"=u16 1044, "File Name"="CCD 0 Port 0 ADC Offset", "Parameter Value"=-1752, "Camera ID"=u8 1) -> ("TCP/IP ID Out"=w240:refnum<k5>, "Error Out"=w259:errorcluster)  [unwired: 9 in, 2 out]
                    n126 = call "Send Single TCP-IP Cmd 1.vi"("TCP/IP ID"=w240, "Camera Color"=w239, "Error In"=w259, "Function #"=u16 1044, "File Name"="CCD 0 Port 0 Correlation Bias ", "Parameter Value"=2010, "Camera ID"=u8 1) -> ("Error Out"=w258:errorcluster)  [unwired: 9 in, 3 out]
                    n127 = call "SI Image Error Handler - Win 2.vi"("error in (no error)"=w258) -> ()  [unwired: 4 in, 1 out]
                  }
                  frame 3 {
                    n128 = call "Send Single TCP-IP Cmd 1.vi"("TCP/IP ID"=w268, "Camera Color"=w267, "Function #"=u16 1044, "File Name"="DSI Sample Time", "Parameter Value"=34, "Camera ID"=u8 1) -> ("TCP/IP ID Out"=w266:refnum<k5>, "Error Out"=w286:errorcluster)  [unwired: 10 in, 2 out]
                    n129 = call "Send Single TCP-IP Cmd 1.vi"("TCP/IP ID"=w266, "Camera Color"=w267, "Error In"=w286, "Function #"=u16 1044, "File Name"="Gain", "Parameter Value"=1, "Camera ID"=u8 1) -> ("TCP/IP ID Out"=w265:refnum<k5>, "Error Out"=w285:errorcluster)  [unwired: 9 in, 2 out]
                    n130 = call "Send Single TCP-IP Cmd 1.vi"("TCP/IP ID"=w265, "Camera Color"=w267, "Error In"=w285, "Function #"=u16 1044, "File Name"="CCD 0 Port 0 ADC Offset", "Parameter Value"=-1691, "Camera ID"=u8 1) -> ("TCP/IP ID Out"=w264:refnum<k5>, "Error Out"=w284:errorcluster)  [unwired: 9 in, 2 out]
                    n131 = call "Send Single TCP-IP Cmd 1.vi"("TCP/IP ID"=w264, "Camera Color"=w267, "Error In"=w284, "Function #"=u16 1044, "File Name"="CCD 0 Port 0 Correlation Bias ", "Parameter Value"=1993, "Camera ID"=u8 1) -> ("Error Out"=w283:errorcluster)  [unwired: 9 in, 3 out]
                    n132 = call "SI Image Error Handler - Win 2.vi"("error in (no error)"=w283) -> ()  [unwired: 4 in, 1 out]
                  }
                  frame 4 {
                    n133 = call "Send Single TCP-IP Cmd 1.vi"("TCP/IP ID"=w292, "Camera Color"=w293, "Function #"=u16 1044, "File Name"="DSI Sample Time", "Parameter Value"=460, "Camera ID"=u8 1) -> ("TCP/IP ID Out"=w291:refnum<k5>, "Error Out"=w311:errorcluster)  [unwired: 10 in, 2 out]
                    n134 = call "Send Single TCP-IP Cmd 1.vi"("TCP/IP ID"=w291, "Camera Color"=w293, "Error In"=w311, "Function #"=u16 1044, "File Name"="Gain", "Parameter Value"=0, "Camera ID"=u8 1) -> ("TCP/IP ID Out"=w290:refnum<k5>, "Error Out"=w310:errorcluster)  [unwired: 9 in, 2 out]
                    n135 = call "Send Single TCP-IP Cmd 1.vi"("TCP/IP ID"=w290, "Camera Color"=w293, "Error In"=w310, "Function #"=u16 1044, "File Name"="CCD 0 Port 0 ADC Offset", "Parameter Value"=-1712, "Camera ID"=u8 1) -> ("TCP/IP ID Out"=w289:refnum<k5>, "Error Out"=w309:errorcluster)  [unwired: 9 in, 2 out]
                    n136 = call "Send Single TCP-IP Cmd 1.vi"("TCP/IP ID"=w289, "Camera Color"=w293, "Error In"=w309, "Function #"=u16 1044, "File Name"="CCD 0 Port 0 Correlation Bias ", "Parameter Value"=2017, "Camera ID"=u8 1) -> ("Error Out"=w308:errorcluster)  [unwired: 9 in, 3 out]
                    n137 = call "SI Image Error Handler - Win 2.vi"("error in (no error)"=w308) -> ()  [unwired: 4 in, 1 out]
                  }
                  frame 5 {
                    n138 = call "Send Single TCP-IP Cmd 1.vi"("TCP/IP ID"=w318, "Camera Color"=w314, "Function #"=u16 1044, "File Name"="DSI Sample Time", "Parameter Value"=460, "Camera ID"=u8 1) -> ("TCP/IP ID Out"=w317:refnum<k5>, "Error Out"=w336:errorcluster)  [unwired: 10 in, 2 out]
                    n139 = call "Send Single TCP-IP Cmd 1.vi"("TCP/IP ID"=w317, "Camera Color"=w314, "Error In"=w336, "Function #"=u16 1044, "File Name"="Gain", "Parameter Value"=1, "Camera ID"=u8 1) -> ("TCP/IP ID Out"=w316:refnum<k5>, "Error Out"=w335:errorcluster)  [unwired: 9 in, 2 out]
                    n140 = call "Send Single TCP-IP Cmd 1.vi"("TCP/IP ID"=w316, "Camera Color"=w314, "Error In"=w335, "Function #"=u16 1044, "File Name"="CCD 0 Port 0 ADC Offset", "Parameter Value"=-1747, "Camera ID"=u8 1) -> ("TCP/IP ID Out"=w315:refnum<k5>, "Error Out"=w334:errorcluster)  [unwired: 9 in, 2 out]
                    n141 = call "Send Single TCP-IP Cmd 1.vi"("TCP/IP ID"=w315, "Camera Color"=w314, "Error In"=w334, "Function #"=u16 1044, "File Name"="CCD 0 Port 0 Correlation Bias ", "Parameter Value"=2011, "Camera ID"=u8 1) -> ("Error Out"=w333:errorcluster)  [unwired: 9 in, 3 out]
                    n142 = call "SI Image Error Handler - Win 2.vi"("error in (no error)"=w333) -> ()  [unwired: 4 in, 1 out]
                  }
                  frame 6 {
                    n143 = call "Send Single TCP-IP Cmd 1.vi"("TCP/IP ID"=w348, "Camera Color"=w349, "Function #"=u16 1044, "File Name"="DSI Sample Time", "Parameter Value"=460, "Camera ID"=u8 1) -> ("TCP/IP ID Out"=w347:refnum<k5>, "Error Out"=w344:errorcluster)  [unwired: 10 in, 2 out]
                    n144 = call "SI Image Error Handler - Win 2.vi"("error in (no error)"=w344) -> ("error out"=w343:errorcluster)  [unwired: 4 in]
                    n145 = call "Send Single TCP-IP Cmd 1.vi"("TCP/IP ID"=w347, "Camera Color"=w349, "Error In"=w343, "Function #"=u16 1044, "File Name"="Gain", "Parameter Value"=1, "Camera ID"=u8 1) -> ("TCP/IP ID Out"=w346:refnum<k5>, "Error Out"=w342:errorcluster)  [unwired: 9 in, 2 out]
                    n146 = call "SI Image Error Handler - Win 2.vi"("error in (no error)"=w342) -> ("error out"=w341:errorcluster)  [unwired: 4 in]
                    n147 = call "Send Single TCP-IP Cmd 1.vi"("TCP/IP ID"=w346, "Camera Color"=w349, "Error In"=w341, "Function #"=u16 1044, "File Name"="CCD 0 Port 0 ADC Offset", "Parameter Value"=-1659, "Camera ID"=u8 1) -> ("TCP/IP ID Out"=w345:refnum<k5>, "Error Out"=w340:errorcluster)  [unwired: 9 in, 2 out]
                    n148 = call "SI Image Error Handler - Win 2.vi"("error in (no error)"=w340) -> ("error out"=w339:errorcluster)  [unwired: 4 in]
                    n149 = call "Send Single TCP-IP Cmd 1.vi"("TCP/IP ID"=w345, "Camera Color"=w349, "Error In"=w339, "Function #"=u16 1044, "File Name"="CCD 0 Port 0 Correlation Bias ", "Parameter Value"=2019, "Camera ID"=u8 1) -> ("Error Out"=w364:errorcluster)  [unwired: 9 in, 3 out]
                    n150 = call "SI Image Error Handler - Win 2.vi"("error in (no error)"=w364) -> ()  [unwired: 4 in, 1 out]
                  }
                }
              }
              frame "Red" {
                # "Resend ROI info because modes wrote over them"
                # "there are 7 default modes from si"
                n151 = Add(x=7, y=w370) -> (x+y=w368:i32)
                n152 = To Unsigned Byte Integer(number=w368) -> (unsigned 8bit integer=w372:u8)
                n153 = call "Send Single TCP-IP Cmd 1.vi"("TCP/IP ID"=w371, "Function #"=u16 1042, "Camera ID"=u8 1, "Acq. Mode/Type/Frame Mode/RO Mode #"=w372) -> ()  [unwired: 12 in, 4 out]
                n154 = local read "CCD ROI Mode"() -> (w367:u16)
                n155 = property on="CCD ROI Mode" class="Ring (strict)"("Val(Sgnl)"=w367) -> ()  [unwired: 2 in, 2 out]
              }
              frame "Blue" {
                n156 = case shown="2" w375 {
                  tunnel: w376 -> [w385 w413 w420 w439 w458 w477 w500 w518 w538]
                  tunnel: w377 -> [w378 w397 w416 w435 w455 w473 w493 w514 w539]
                  frame 8 {
                    n157 = call "Send Single TCP-IP Cmd 1.vi"("TCP/IP ID"=w385, "Camera Color"=w378, "Function #"=u16 1044, "File Name"="DSI Sample Time", "Parameter Value"=30, "Camera ID"=u8 1) -> ("TCP/IP ID Out"=w381:refnum<k5>, "Error Out"=w394:errorcluster)  [unwired: 10 in, 2 out]
                    n158 = call "Send Single TCP-IP Cmd 1.vi"("TCP/IP ID"=w381, "Camera Color"=w378, "Error In"=w394, "Function #"=u16 1044, "File Name"="Analog Attenuation", "Parameter Value"=0, "Camera ID"=u8 1) -> ("TCP/IP ID Out"=w380:refnum<k5>, "Error Out"=w379:errorcluster)  [unwired: 9 in, 2 out]
                    n159 = call "Send Single TCP-IP Cmd 1.vi"("TCP/IP ID"=w380, "Camera Color"=w378, "Error In"=w379, "Function #"=u16 1044, "File Name"="CCD 0 Port 1 Correlation Bias", "Parameter Value"=1836, "Camera ID"=u8 1) -> ("Error Out"=w393:errorcluster)  [unwired: 9 in, 3 out]
                    n160 = call "SI Image Error Handler - Win 2.vi"("error in (no error)"=w393) -> ()  [unwired: 4 in, 1 out]
                  }
                  frame 7 {
                    n161 = call "Send Single TCP-IP Cmd 1.vi"("TCP/IP ID"=w413, "Camera Color"=w397, "Function #"=u16 1044, "File Name"="DSI Sample Time", "Parameter Value"=130, "Camera ID"=u8 1) -> ("TCP/IP ID Out"=w403:refnum<k5>, "Error Out"=w412:errorcluster)  [unwired: 10 in, 2 out]
                    n162 = call "Send Single TCP-IP Cmd 1.vi"("TCP/IP ID"=w403, "Camera Color"=w397, "Error In"=w412, "Function #"=u16 1044, "File Name"="Analog Attenuation", "Parameter Value"=2, "Camera ID"=u8 1) -> ("TCP/IP ID Out"=w399:refnum<k5>, "Error Out"=w398:errorcluster)  [unwired: 9 in, 2 out]
                    n163 = call "Send Single TCP-IP Cmd 1.vi"("TCP/IP ID"=w399, "Camera Color"=w397, "Error In"=w398, "Function #"=u16 1044, "File Name"="CCD 0 Port 1 Correlation Bias ", "Parameter Value"=1880, "Camera ID"=u8 1) -> ("Error Out"=w411:errorcluster)  [unwired: 9 in, 3 out]
                    n164 = call "SI Image Error Handler - Win 2.vi"("error in (no error)"=w411) -> ()  [unwired: 4 in, 1 out]
                  }
                  frame 6 {
                    n165 = call "Send Single TCP-IP Cmd 1.vi"("TCP/IP ID"=w420, "Camera Color"=w416, "Function #"=u16 1044, "File Name"="DSI Sample Time", "Parameter Value"=130, "Camera ID"=u8 1) -> ("TCP/IP ID Out"=w419:refnum<k5>, "Error Out"=w432:errorcluster)  [unwired: 10 in, 2 out]
                    n166 = call "Send Single TCP-IP Cmd 1.vi"("TCP/IP ID"=w419, "Camera Color"=w416, "Error In"=w432, "Function #"=u16 1044, "File Name"="Analog Attenuation", "Parameter Value"=0, "Camera ID"=u8 1) -> ("TCP/IP ID Out"=w418:refnum<k5>, "Error Out"=w417:errorcluster)  [unwired: 9 in, 2 out]
                    n167 = call "Send Single TCP-IP Cmd 1.vi"("TCP/IP ID"=w418, "Camera Color"=w416, "Error In"=w417, "Function #"=u16 1044, "File Name"="CCD 0 Port 1 Correlation Bias ", "Parameter Value"=1877, "Camera ID"=u8 1) -> ("Error Out"=w431:errorcluster)  [unwired: 9 in, 3 out]
                    n168 = call "SI Image Error Handler - Win 2.vi"("error in (no error)"=w431) -> ()  [unwired: 4 in, 1 out]
                  }
                  frame 5 {
                    n169 = call "Send Single TCP-IP Cmd 1.vi"("TCP/IP ID"=w439, "Camera Color"=w435, "Function #"=u16 1044, "File Name"="DSI Sample Time", "Parameter Value"=330, "Camera ID"=u8 1) -> ("TCP/IP ID Out"=w438:refnum<k5>, "Error Out"=w451:errorcluster)  [unwired: 10 in, 2 out]
                    n170 = call "Send Single TCP-IP Cmd 1.vi"("TCP/IP ID"=w438, "Camera Color"=w435, "Error In"=w451, "Function #"=u16 1044, "File Name"="Analog Attenuation", "Parameter Value"=3, "Camera ID"=u8 1) -> ("TCP/IP ID Out"=w436:refnum<k5>, "Error Out"=w437:errorcluster)  [unwired: 9 in, 2 out]
                    n171 = call "Send Single TCP-IP Cmd 1.vi"("TCP/IP ID"=w436, "Camera Color"=w435, "Error In"=w437, "Function #"=u16 1044, "File Name"="CCD 0 Port 1 Correlation Bias ", "Parameter Value"=1911, "Camera ID"=u8 1) -> ("Error Out"=w450:errorcluster)  [unwired: 9 in, 3 out]
                    n172 = call "SI Image Error Handler - Win 2.vi"("error in (no error)"=w450) -> ()  [unwired: 4 in, 1 out]
                  }
                  frame 4 {
                    n173 = call "Send Single TCP-IP Cmd 1.vi"("TCP/IP ID"=w458, "Camera Color"=w455, "Function #"=u16 1044, "File Name"="DSI Sample Time", "Parameter Value"=330, "Camera ID"=u8 1) -> ("TCP/IP ID Out"=w457:refnum<k5>, "Error Out"=w470:errorcluster)  [unwired: 10 in, 2 out]
                    n174 = call "Send Single TCP-IP Cmd 1.vi"("TCP/IP ID"=w457, "Camera Color"=w455, "Error In"=w470, "Function #"=u16 1044, "File Name"="Analog Attenuation", "Parameter Value"=2, "Camera ID"=u8 1) -> ("TCP/IP ID Out"=w454:refnum<k5>, "Error Out"=w456:errorcluster)  [unwired: 9 in, 2 out]
                    n175 = call "Send Single TCP-IP Cmd 1.vi"("TCP/IP ID"=w454, "Camera Color"=w455, "Error In"=w456, "Function #"=u16 1044, "File Name"="CCD 0 Port 1 Correlation Bias ", "Parameter Value"=1984, "Camera ID"=u8 1) -> ("Error Out"=w469:errorcluster)  [unwired: 9 in, 3 out]
                    n176 = call "SI Image Error Handler - Win 2.vi"("error in (no error)"=w469) -> ()  [unwired: 4 in, 1 out]
                  }
                  frame 3 {
                    n177 = call "Send Single TCP-IP Cmd 1.vi"("TCP/IP ID"=w477, "Camera Color"=w473, "Function #"=u16 1044, "File Name"="DSI Sample Time", "Parameter Value"=330, "Camera ID"=u8 1) -> ("TCP/IP ID Out"=w476:refnum<k5>, "Error Out"=w489:errorcluster)  [unwired: 10 in, 2 out]
                    n178 = call "Send Single TCP-IP Cmd 1.vi"("TCP/IP ID"=w476, "Camera Color"=w473, "Error In"=w489, "Function #"=u16 1044, "File Name"="Analog Attenuation", "Parameter Value"=0, "Camera ID"=u8 1) -> ("TCP/IP ID Out"=w475:refnum<k5>, "Error Out"=w474:errorcluster)  [unwired: 9 in, 2 out]
                    n179 = call "Send Single TCP-IP Cmd 1.vi"("TCP/IP ID"=w475, "Camera Color"=w473, "Error In"=w474, "Function #"=u16 1044, "File Name"="CCD 0 Port 1 Correlation Bias ", "Parameter Value"=1984, "Camera ID"=u8 1) -> ("Error Out"=w488:errorcluster)  [unwired: 9 in, 3 out]
                    n180 = call "SI Image Error Handler - Win 2.vi"("error in (no error)"=w488) -> ()  [unwired: 4 in, 1 out]
                  }
                  frame 2 {
                    n181 = call "Send Single TCP-IP Cmd 1.vi"("TCP/IP ID"=w500, "Camera Color"=w493, "Function #"=u16 1044, "File Name"="DSI Sample Time", "Parameter Value"=746, "Camera ID"=u8 1) -> ("TCP/IP ID Out"=w499:refnum<k5>, "Error Out"=w498:errorcluster)  [unwired: 10 in, 2 out]
                    n182 = call "SI Image Error Handler - Win 2.vi"("error in (no error)"=w498) -> ("error out"=w497:errorcluster)  [unwired: 4 in]
                    n183 = call "Send Single TCP-IP Cmd 1.vi"("TCP/IP ID"=w499, "Camera Color"=w493, "Error In"=w497, "Function #"=u16 1044, "File Name"="Analog Attenuation", "Parameter Value"=3, "Camera ID"=u8 1) -> ("TCP/IP ID Out"=w492:refnum<k5>, "Error Out"=w496:errorcluster)  [unwired: 9 in, 2 out]
                    n184 = call "SI Image Error Handler - Win 2.vi"("error in (no error)"=w496) -> ("error out"=w494:errorcluster)  [unwired: 4 in]
                    n185 = call "SI Image Error Handler - Win 2.vi"("error in (no error)"=w494) -> ("error out"=w495:errorcluster)  [unwired: 4 in]
                    n186 = call "Send Single TCP-IP Cmd 1.vi"("TCP/IP ID"=w492, "Camera Color"=w493, "Error In"=w495, "Function #"=u16 1044, "File Name"="CCD 0 Port 1 Correlation Bias ", "Parameter Value"=1968, "Camera ID"=u8 1) -> ("Error Out"=w511:errorcluster)  [unwired: 9 in, 3 out]
                    n187 = call "SI Image Error Handler - Win 2.vi"("error in (no error)"=w511) -> ()  [unwired: 4 in, 1 out]
                  }
                  frame 1 {
                    n188 = call "Send Single TCP-IP Cmd 1.vi"("TCP/IP ID"=w518, "Camera Color"=w514, "Function #"=u16 1044, "File Name"="DSI Sample Time", "Parameter Value"=746, "Camera ID"=u8 1) -> ("TCP/IP ID Out"=w522:refnum<k5>, "Error Out"=w521:errorcluster)  [unwired: 10 in, 2 out]
                    n189 = call "SI Image Error Handler - Win 2.vi"("error in (no error)"=w521) -> ("error out"=w520:errorcluster)  [unwired: 4 in]
                    n190 = call "Send Single TCP-IP Cmd 1.vi"("TCP/IP ID"=w522, "Camera Color"=w514, "Error In"=w520, "Function #"=u16 1044, "File Name"="Analog Attenuation", "Parameter Value"=2, "Camera ID"=u8 1) -> ("TCP/IP ID Out"=w516:refnum<k5>, "Error Out"=w519:errorcluster)  [unwired: 9 in, 2 out]
                    n191 = call "SI Image Error Handler - Win 2.vi"("error in (no error)"=w519) -> ("error out"=w515:errorcluster)  [unwired: 4 in]
                    n192 = call "Send Single TCP-IP Cmd 1.vi"("TCP/IP ID"=w516, "Camera Color"=w514, "Error In"=w515, "Function #"=u16 1044, "File Name"="CCD 0 Port 1 Correlation Bias ", "Parameter Value"=1984, "Camera ID"=u8 1) -> ("Error Out"=w532:errorcluster)  [unwired: 9 in, 3 out]
                    n193 = call "SI Image Error Handler - Win 2.vi"("error in (no error)"=w532) -> ()  [unwired: 4 in, 1 out]
                  }
                  frame 0, Default {
                    n194 = call "Send Single TCP-IP Cmd 1.vi"("TCP/IP ID"=w538, "Camera Color"=w539, "Function #"=u16 1044, "File Name"="DSI Sample Time", "Parameter Value"=746, "Camera ID"=u8 1) -> ("TCP/IP ID Out"=w544:refnum<k5>, "Error Out"=w543:errorcluster)  [unwired: 10 in, 2 out]
                    n195 = call "SI Image Error Handler - Win 2.vi"("error in (no error)"=w543) -> ("error out"=w542:errorcluster)  [unwired: 4 in]
                    n196 = call "Send Single TCP-IP Cmd 1.vi"("TCP/IP ID"=w544, "Camera Color"=w539, "Error In"=w542, "Function #"=u16 1044, "File Name"="Analog Attenuation", "Parameter Value"=0, "Camera ID"=u8 1) -> ("TCP/IP ID Out"=w535:refnum<k5>, "Error Out"=w541:errorcluster)  [unwired: 9 in, 2 out]
                    n197 = call "SI Image Error Handler - Win 2.vi"("error in (no error)"=w541) -> ("error out"=w536:errorcluster)  [unwired: 4 in]
                    n198 = call "SI Image Error Handler - Win 2.vi"("error in (no error)"=w536) -> ("error out"=w540:errorcluster)  [unwired: 4 in]
                    n199 = call "Send Single TCP-IP Cmd 1.vi"("TCP/IP ID"=w535, "Camera Color"=w539, "Error In"=w540, "Function #"=u16 1044, "File Name"="CCD 0 Port 1 Correlation Bias ", "Parameter Value"=1984, "Camera ID"=u8 1) -> ("Error Out"=w554:errorcluster)  [unwired: 9 in, 3 out]
                    n200 = call "SI Image Error Handler - Win 2.vi"("error in (no error)"=w554) -> ()  [unwired: 4 in, 1 out]
                  }
                }
              }
            }
            n201 = Bundle By Name(cluster=w176, "Other Info..CCD Gain"=w175, "Other Info..CCD Read Noise"=w174) -> (w173:T6)
            n202 = local write "Script"(w173) -> ()
          }
          event "CCD ROI Mode": Value Change {
            # "Send ROI parameters to camera server, recalculate RO time, trimsec, ccdsum"
            n203 = event-data() -> ("OldVal"=w561:u16, "NewVal"=w562:u16)  [unwired: 1 in, 4 out]
            n204 = local read "CCD ROI"() -> (w578:cluster{i32, i32, i32, i32, i32, i32})
            n205 = local read "Port Readout"() -> (w583:u16)
            n206 = Unbundle(w578) -> (w577:i32, w576:i32, w575:i32, w574:i32, w573:i32, w572:i32)
            n207 = Not Equal To 0?(x=w583) -> (x != 0?=w582:bool)
            n208 = case shown="True" w582 {
              tunnel: w562 -> [w612 w769]
              tunnel: [w626 w768] -> w590
              tunnel: [w625 w767] -> w589
              tunnel: [w624 w766] -> w569
              tunnel: [w623 w765] -> w588
              tunnel: [w622 w764] -> w587
              tunnel: [w621 w763] -> w586
              tunnel: [w620 w762] -> w558
              tunnel: w577 -> [w619 w761]
              tunnel: w576 -> [w618 w760]
              tunnel: w575 -> [w617 w759]
              tunnel: w574 -> [w616 w758]
              tunnel: w573 -> [w615 w757]
              tunnel: w572 -> [w614 w756]
              tunnel: w561 -> [w613 w755]
              tunnel: [w611 w754] -> w567
              tunnel: w557 -> [_ w753]
              frame False {
                # "4-port RO"
                n209 = case shown="1" w612 {
                  selector: w612 -> [w627 w635 w643 w651 w659 w667 w675 w683 w691 w699 w714 w715 w730 _]
                  tunnel: [516 516 516 16 16 16 0 0 0 0 0 1850 1366 w745] -> w626
                  tunnel: [1548 774 516 2048 1024 683 4142 2071 1381 2071 2071 200 1370 w744] -> w625
                  tunnel: [1 2 3 1 2 3 1 2 3 2 2 1 1 w743] -> w624
                  tunnel: [500 500 500 1100 1100 1100 740 740 740 1800 980 1100 790 w742] -> w623
                  tunnel: [1548 774 516 948 474 316 2514 1257 838 200 1008 948 2370 w741] -> w622
                  tunnel: [1 2 3 1 2 3 1 2 3 2 2 1 1 w740] -> w621
                  tunnel: ["Imaging 1x1" ("Current Status") "Imaging 2x2" ("Current Status") "Imaging 3x3" ("Current Status") "Spectroscopic 1x1" ("Current Status") "Spectroscopic 2x2" ("Current Status") "Spectroscopic 3x3" ("Current Status") "MOS 1x1" ("Current Status") "MOS 2x2" ("Current Status") "MOS 3x3" ("Current Status") "Spectroscopic ZZ Ceti" ("Current Status") "Slicer" ("Current Status") "Slit Imaging/Alignment" ("Current Status") "MOS Imaging/Alignment" ("Current Status") "user-defined" ("Current Status")] -> w620
                  tunnel: w619 -> [_ _ _ _ _ _ _ _ _ _ _ _ _ w738]
                  tunnel: w618 -> [_ _ _ _ _ _ _ _ _ _ _ _ _ w737]
                  tunnel: w617 -> [_ _ _ _ _ _ _ _ _ _ _ _ _ w736]
                  tunnel: w616 -> [_ _ _ _ _ _ _ _ _ _ _ _ _ w735]
                  tunnel: w615 -> [_ _ _ _ _ _ _ _ _ _ _ _ _ w734]
                  tunnel: w614 -> [_ _ _ _ _ _ _ _ _ _ _ _ _ w733]
                  tunnel: w613 -> [_ _ _ _ _ _ _ _ _ _ _ _ _ w732]
                  tunnel: [w627 w635 w643 w651 w659 w667 w675 w683 w691 w699 w714 w715 w730 w731] -> w611
                  frame 0, Default {
                  }
                  frame 1 {
                  }
                  frame 2 {
                  }
                  frame 3 {
                  }
                  frame 4 {
                  }
                  frame 5 {
                  }
                  frame 11 {
                  }
                  frame 12 {
                  }
                  frame 13 {
                  }
                  frame 14 {
                  }
                  frame 6 {
                  }
                  frame 7 {
                  }
                  frame 10 {
                  }
                  frame 8, 9 {
                    n210 = call "GetCCDParameters.vi"("Serial Origin"=w738, "Parallel Origin"=w735, "Serial Length"=w737, "Parallel Length"=w734, "Serial Binning"=w736, "Parallel Binning"=w733) -> ("Cancelled?"=w747:bool, "CCD Format Parameters"=w748:T14)  [unwired: 10 in, 2 out]
                    n211 = case shown="False" w747 {
                      tunnel: w748 -> [w750 _]
                      tunnel: [w750 w752] -> w746
                      tunnel: w732 -> [_ w751]
                      tunnel: [u8 8 ("Camera ID") w751] -> w731
                      frame False {
                      }
                      frame True {
                        n212 = local read "CCD ROI"() -> (w752:cluster{i32, i32, i32, i32, i32, i32})
                      }
                    }
                    n213 = Unbundle(w746) -> ("Serial Origin"=w745:i32, "Serial Length"=w744:i32, "Serial Binning"=w743:i32, "Parallel Origin"=w742:i32, "Parallel Length"=w741:i32, "Parallel Binning"=w740:i32)
                  }
                }
              }
              frame True {
                # "1-port RO"
                n214 = case shown="\"Red\", Default" w753 {
                  tunnel: w769 -> [w770 w938]
                  tunnel: [w782 w937] -> w768
                  tunnel: [w780 w936] -> w767
                  tunnel: [w779 w935] -> w766
                  tunnel: [w778 w934] -> w765
                  tunnel: [w783 w933] -> w764
                  tunnel: [w784 w932] -> w763
                  tunnel: [w785 w931] -> w762
                  tunnel: w761 -> [w777 w930]
                  tunnel: w760 -> [w776 w929]
                  tunnel: w759 -> [w775 w928]
                  tunnel: w758 -> [w774 w927]
                  tunnel: w757 -> [w773 w926]
                  tunnel: w756 -> [w772 w925]
                  tunnel: w755 -> [w771 w924]
                  tunnel: [w781 w923] -> w754
                  frame "Blue" {
                    n215 = case shown="8, 9" w770 {
                      selector: w770 -> [w786 w794 w802 w810 w818 w826 w834 w842 w850 w858 w873 w874 w882 _]
                      tunnel: [516 516 516 0 0 0 0 0 0 0 0 1850 1366 w904] -> w782
                      tunnel: [3096 1548 1032 4142 2071 1381 4142 2071 1381 2071 2071 400 1370 w903] -> w780
                      tunnel: [1 2 3 1 2 3 1 2 3 2 2 1 1 w902] -> w779
                      tunnel: [500 500 500 1100 1100 1100 740 740 740 1800 980 1100 790 w901] -> w778
                      tunnel: [3096 1548 1032 1896 948 632 2514 1257 838 200 1048 1896 2370 w900] -> w783
                      tunnel: [1 2 3 1 2 3 1 2 3 2 2 1 1 w899] -> w784
                      tunnel: ["Imaging 1x1" ("Current Status") "Imaging 2x2" ("Current Status") "Imaging 3x3" ("Current Status") "Spectroscopic 1x1" ("Current Status") "Spectroscopic 2x2" ("Current Status") "Spectroscopic 3x3" ("Current Status") "MOS 1x1" ("Current Status") "MOS 2x2" ("Current Status") "MOS 3x3" ("Current Status") "Spectroscopic ZZ Ceti" ("Current Status") "Slicer" ("Current Status") "Slit Imaging/Alignment" ("Current Status") "MOS Imaging/Alignment" ("Current Status") "user-defined" ("Current Status")] -> w785
                      tunnel: w777 -> [_ _ _ _ _ _ _ _ _ _ _ _ _ w897]
                      tunnel: w776 -> [_ _ _ _ _ _ _ _ _ _ _ _ _ w896]
                      tunnel: w775 -> [_ _ _ _ _ _ _ _ _ _ _ _ _ w895]
                      tunnel: w774 -> [_ _ _ _ _ _ _ _ _ _ _ _ _ w894]
                      tunnel: w773 -> [_ _ _ _ _ _ _ _ _ _ _ _ _ w893]
                      tunnel: w772 -> [_ _ _ _ _ _ _ _ _ _ _ _ _ w892]
                      tunnel: w771 -> [_ _ _ _ _ _ _ _ _ _ _ _ _ w891]
                      tunnel: [w786 w794 w802 w810 w818 w826 w834 w842 w850 w858 w873 w874 w882 w890] -> w781
                      frame 0, Default {
                      }
                      frame 1 {
                      }
                      frame 2 {
                      }
                      frame 3 {
                      }
                      frame 4 {
                      }
                      frame 5 {
                      }
                      frame 11 {
                      }
                      frame 12 {
                      }
                      frame 13 {
                      }
                      frame 14 {
                      }
                      frame 6 {
                      }
                      frame 7 {
                      }
                      frame 10 {
                      }
                      frame 8, 9 {
                        n216 = call "GetCCDParameters.vi"("Serial Origin"=w897, "Parallel Origin"=w894, "Serial Length"=w896, "Parallel Length"=w893, "Serial Binning"=w895, "Parallel Binning"=w892) -> ("Cancelled?"=w906:bool, "CCD Format Parameters"=w905:T14)  [unwired: 10 in, 2 out]
                        n217 = case shown="False" w906 {
                          tunnel: w905 -> [w914 _]
                          tunnel: [w913 w921] -> w904
                          tunnel: [w912 w920] -> w903
                          tunnel: [w911 w919] -> w902
                          tunnel: [w910 w918] -> w901
                          tunnel: [w909 w917] -> w900
                          tunnel: [w908 w916] -> w899
                          tunnel: w891 -> [_ w915]
                          tunnel: [u8 8 ("Camera ID") w915] -> w890
                          frame False {
                            n218 = Unbundle(w914) -> ("Serial Origin"=w913:i32, "Serial Length"=w912:i32, "Serial Binning"=w911:i32, "Parallel Origin"=w910:i32, "Parallel Length"=w909:i32, "Parallel Binning"=w908:i32)
                          }
                          frame True {
                            n219 = local read "CCD ROI"() -> (w922:cluster{i32, i32, i32, i32, i32, i32})
                            n220 = Unbundle(w922) -> (w921:i32, w920:i32, w919:i32, w918:i32, w917:i32, w916:i32)
                          }
                        }
                      }
                    }
                  }
                  frame "Red", Default {
                    n221 = case shown="8, 9" w938 {
                      selector: w938 -> [w939 w947 w955 w963 w971 w979 w987 w995 w1003 w1011 w1020 w1036 w1037 w1045 _]
                      tunnel: [530 530 530 0 0 0 0 0 0 0 w1026 0 1300 1300 w1067] -> w937
                      tunnel: [3096 1548 1032 4142 2071 1381 4142 2071 1381 2071 w1025 2071 1500 1500 w1066] -> w936
                      tunnel: [1 2 3 1 2 3 1 2 3 2 w1024 2 1 1 w1065] -> w935
                      tunnel: [388 388 388 980 980 980 650 650 650 1800 w1023 900 1100 790 w1064] -> w934
                      tunnel: [3096 1548 1032 1896 948 632 2514 1257 838 200 w1022 1048 1896 2370 w1063] -> w933
                      tunnel: [1 2 3 1 2 3 1 2 3 2 w1021 2 1 1 w1062] -> w932
                      tunnel: ["Imaging 1x1" ("Current Status") "Imaging 2x2" ("Current Status") "Imaging 3x3" ("Current Status") "Spectroscopic 1x1" ("Current Status") "Spectroscopic 2x2" ("Current Status") "Spectroscopic 3x3" ("Current Status") "MOS 1x1" ("Current Status") "MOS 2x2" ("Current Status") "MOS 3x3" ("Current Status") "Spectroscopic ZZ Ceti" ("Current Status") "Custom from Script" "Slicer" ("Current Status") "Slit Imaging/Alignment" ("Current Status") "MOS Imaging/Alignment" ("Current Status") "user-defined" ("Current Status")] -> w931
                      tunnel: w930 -> [_ _ _ _ _ _ _ _ _ _ _ _ _ _ w1060]
                      tunnel: w929 -> [_ _ _ _ _ _ _ _ _ _ _ _ _ _ w1059]
                      tunnel: w928 -> [_ _ _ _ _ _ _ _ _ _ _ _ _ _ w1058]
                      tunnel: w927 -> [_ _ _ _ _ _ _ _ _ _ _ _ _ _ w1057]
                      tunnel: w926 -> [_ _ _ _ _ _ _ _ _ _ _ _ _ _ w1056]
                      tunnel: w925 -> [_ _ _ _ _ _ _ _ _ _ _ _ _ _ w1055]
                      tunnel: w924 -> [_ _ _ _ _ _ _ _ _ _ _ _ _ _ w1054]
                      tunnel: [w939 w947 w955 w963 w971 w979 w987 w995 w1003 w1011 w1020 w1036 w1037 w1045 w1053] -> w923
                      frame 0, Default {
                      }
                      frame 1 {
                      }
                      frame 2 {
                      }
                      frame 3 {
                      }
                      frame 4 {
                      }
                      frame 5 {
                      }
                      frame 11 {
                      }
                      frame 12 {
                      }
                      frame 13 {
                      }
                      frame 14 {
                      }
                      frame 21 {
                        # "wait just to make sure Roi updates"
                        n222 = global read "SIcamera_Globals.vi" "CCD ROI"() -> (w1027:cluster{i32, i32, i32, i32, i32, i32})
                        n223 = Wait (ms)(milliseconds to wait=50) -> ()  [unwired: 1 out]
                        n224 = Unbundle(w1027) -> (w1026:i32, w1025:i32, w1024:i32, w1023:i32, w1022:i32, w1021:i32)
                      }
                      frame 6 {
                      }
                      frame 7 {
                      }
                      frame 10 {
                      }
                      frame 8, 9 {
                        n225 = call "GetCCDParameters.vi"("Serial Origin"=w1060, "Parallel Origin"=w1057, "Serial Length"=w1059, "Parallel Length"=w1056, "Serial Binning"=w1058, "Parallel Binning"=w1055) -> ("Cancelled?"=w1069:bool, "CCD Format Parameters"=w1068:T14)  [unwired: 10 in, 2 out]
                        n226 = case shown="True" w1069 {
                          tunnel: w1068 -> [w1077 _]
                          tunnel: [w1076 w1084] -> w1067
                          tunnel: [w1075 w1083] -> w1066
                          tunnel: [w1074 w1082] -> w1065
                          tunnel: [w1073 w1081] -> w1064
                          tunnel: [w1072 w1080] -> w1063
                          tunnel: [w1071 w1079] -> w1062
                          tunnel: w1054 -> [_ w1078]
                          tunnel: [u8 8 ("Camera ID") w1078] -> w1053
                          frame False {
                            n227 = Unbundle(w1077) -> ("Serial Origin"=w1076:i32, "Serial Length"=w1075:i32, "Serial Binning"=w1074:i32, "Parallel Origin"=w1073:i32, "Parallel Length"=w1072:i32, "Parallel Binning"=w1071:i32)
                          }
                          frame True {
                            n228 = local read "CCD ROI"() -> (w1085:cluster{i32, i32, i32, i32, i32, i32})
                            n229 = Unbundle(w1085) -> (w1084:i32, w1083:i32, w1082:i32, w1081:i32, w1080:i32, w1079:i32)
                          }
                        }
                      }
                    }
                  }
                }
              }
            }
            n230 = Bundle("Serial Origin"=w590, "Serial Length"=w589, "Serial Binning"=w569, "Parallel Origin"=w588, "Parallel Length"=w587, "Parallel Binning"=w586) -> (w568:T14)  [unwired: 1 in]
            "CCD ROI" <- w568
            n231 = local write "ROIMODE"(w558) -> ()
            n232 = Concatenate Strings("Setting " ("string"), w558, " mode..." ("Current Status")) -> ()  [unwired: 1 out]
            n233 = flat-sequence {
              tunnel: w571 -> [w594]
              tunnel: w568 -> [w593]
              tunnel: w557 -> [w592]
              tunnel: [w591] -> w560
              tunnel: w560 -> [w602]
              tunnel: [w601] -> w559
              tunnel: w557 -> [w598]
              tunnel: w559 -> [w606]
              tunnel: w557 -> [w605]
              frame #0 {
                n234 = call "Send Single TCP-IP Cmd 1.vi"("TCP/IP ID"=w594, "Camera Color"=w592, "Function #"=u16 1043, "Camera ID"=u8 1, "CCD Format Parameters"=w593) -> ("TCP/IP ID Out"=w591:refnum<k5>, "Error Out"=w595:errorcluster)  [unwired: 11 in, 2 out]
                n235 = call "SI Image Error Handler - Win 2.vi"("error in (no error)"=w595) -> ()  [unwired: 4 in, 1 out]
              }
              frame #1 {
                n236 = call "Send Single TCP-IP Cmd 1.vi"("TCP/IP ID"=w602, "Camera Color"=w598, "Function #"=u16 1044, "File Name"="Parallel Post Scan", "Parameter Value"=0, "Camera ID"=u8 1) -> ("TCP/IP ID Out"=w601:refnum<k5>)  [unwired: 10 in, 3 out]
              }
              frame #2 {
                n237 = call "Send Single TCP-IP Cmd 1.vi"("TCP/IP ID"=w606, "Camera Color"=w605, "Function #"=u16 1044, "File Name"="Serial Post Scan", "Parameter Value"=0, "Camera ID"=u8 1) -> ()  [unwired: 10 in, 4 out]
              }
            }
            n238 = local write "CCD ROI Mode"(w567) -> ()
            n239 = local read "CCD Readout Speed"() -> (w580:u8)
            n240 = call "DataSectionCalculator.vi"("Standard Mode #"=w567, "CCD ROI"=w568) -> ("CCDSUM"=w564:string, "TRIMSEC"=w565:string)
            n241 = call "CalculateCCDReadoutTime.vi"("Color"=w557, "Readout Speed"=w580, "CCD ROI"=w568) -> ("Readout Time"=w581:dbl)
            n242 = Bundle By Name(cluster=w566, "Reduction Info..DATASEC"=w565, "Reduction Info..CCDSUM"=w564) -> (w563:T6)
            n243 = local write "Readout Time"(w581) -> ()
            n244 = local write "Current Status"("Setting new ROI mode..." ("Current Status")) -> ()
            n245 = local write "Script"(w563) -> ()
          }
          event "Port Readout": Value Change {
            w1104 = u8 5 items=["50 kHz, ATTN 0", "50 kHz, ATTN 2", "50 kHz, ATTN 3", "100 kHz, ATTN 0", "100 kHz, ATTN 2", "100 kHz, ATTN 3", "200 kHz, ATTN 0", "200 kHz, ATTN 2", "400 kHz, ATTN 0"] ("CCD Readout Speed")
            # "Send camera server mode number to read from .set file to set correct port readout choice, get GAIN & RO noise"
            # "Can remove this once I take care of all of the RO speed possibilties for port modes in *.set file"
            # "Add 9 because there are nine previous modes before getting to Port-changing modes in .set file"
            n246 = event-data() -> ("NewVal"=w1088:u16)  [unwired: 1 in, 1 out]
            n247 = Decrement(x=w1088) -> (x-1=w1087:u16)
            n248 = Less?(x=w1087, y=u16 0) -> (x < y?=w1093:bool)
            n249 = Select(t=0.0, s=w1093, f=w1087) -> (s? t:f=w1091:dbl)
            n250 = Multiply(x=w1091, y=u16 10) -> (x*y=w1095:dbl)
            n251 = Add(x=5.0, y=w1095) -> (x+y=w1090:dbl)
            n252 = call "GetCCDPerformanceInfo.vi"("Color"=w1086, "RO Speed Mode"=w1090) -> ("Read Noise"=w1099:dbl, "Gain"=w1100:dbl)
            n253 = Add(x=w1088, y=9) -> (x+y=w1106:i32)
            n254 = call <vilib>:"Set Busy.vi"() -> ("error out"=w1102:errorcluster)  [unwired: 10 in, 1 out]
            n255 = Bundle By Name(cluster=w1098, "Other Info..CCD Gain"=w1100, "Other Info..CCD Read Noise"=w1099) -> (w1097:T6)
            n256 = call "Send Single TCP-IP Cmd 1.vi"("TCP/IP ID"=w1107, "Camera Color"=w1086, "Error In"=w1102, "Function #"=u16 1042, "Camera ID"=u8 1, "Acq. Mode/Type/Frame Mode/RO Mode #"=w1106) -> ("Error Out"=w1110:errorcluster)  [unwired: 10 in, 3 out]
            n257 = local write "CCD Readout Speed"(w1104) -> ()
            n258 = call "SI Image Error Handler - Win 2.vi"("error in (no error)"=w1110) -> ("error out"=w1101:errorcluster)  [unwired: 4 in]
            n259 = call <vilib>:"Unset Busy.vi"("error in (no error)"=w1101) -> ()  [unwired: 10 in, 1 out]
            n260 = local write "Current Status"("Changing CCD port readout mode..." ("Current Status")) -> ()
            n261 = local write "Script"(w1097) -> ()
          }
          event "Calculate Offset": Value Change {
            w1137 = 0.0 ("f")
            w1138 = 1.0 ("t")
            n262 = event-data() -> ()  [unwired: 1 in, 1 out]
            n263 = call "GetTCSInfo.vi"() -> ("TCSInfo"=w1122:T15)
            n264 = Unbundle By Name(w1122) -> ("Mount Az"=w1115:dbl, "Rotator Angle"=w1121:dbl, "Mount El"=w1120:dbl)
            n265 = global read "TCSLINK_global.vi" "Position Angle"() -> (w1111:dbl)
            n266 = local read "CCD ROI"() -> (w1127:cluster{i32, i32, i32, i32, i32, i32})
            n267 = Subtract(x=w1121, y=w1120) -> (x-y=w1114:dbl)
            n268 = Divide(x=3.141592653589793, y=180.0) -> (x/y=w1118:dbl)
            n269 = Compound Arithmetic op=ADD(w1115, w1114, 180.0 ("value")) -> ()  [unwired: 1 out]
            n270 = Unbundle(w1127) -> (w1126:i32, w1125:i32)  [unwired: 4 out]
            n271 = Multiply(x=w1111, y=w1118) -> (x*y=w1112:dbl)
            n272 = formula code="ew_o = x_o*cos(p)*b_x+y_o*sin(p)*b_y;\nns_o = -x_o*sin(p)*b_x+y_o*cos(p)*b_y;\new_s = x_s*cos(p)*b_x+y_s*sin(p)*b_y;\nns_s = -x_s*sin(p)*b_x+y_s*cos(p)*b_y;\new_move=((ew_o-ew_s)*0.146);\nns_move=((ns_o-ns_s)*0.146);"("x_o"="ox1", "y_o"="oy1", "x_s"="sx1", "y_s"="sy1", "b_x"=w1126, "b_y"=w1125, "p"=w1112) -> ("ew_move"=w1134:dbl, "ns_move"=w1135:dbl)  [unwired: 4 out]
            n273 = Less Than 0?(x=w1135) -> (x < 0?=w1139:bool)
            n274 = Select(t=w1138, s=w1139, f=w1137) -> (s? t:f=w1129:dbl)
            n275 = local write "N/S Offset Choice"(w1129) -> ()
            n276 = Less Than 0?(x=w1134) -> (x < 0?=w1136:bool)
            n277 = Select(t=w1138, s=w1136, f=w1137) -> (s? t:f=w1128:dbl)
            n278 = local write "E/W Offset Choice"(w1128) -> ()
            n279 = Absolute Value(x=w1134) -> (abs(x)=w1124:dbl)
            n280 = Absolute Value(x=w1135) -> (abs(x)=w1123:dbl)
            n281 = local write "E/W Offset"(w1124) -> ()
            n282 = local write "N/S Offset"(w1123) -> ()
            n283 = local write "Calculate Offset"(FALSE ("Calculate Offset")) -> ()
          }
          event "Lamp Cluster": Value Change {
            n284 = event-data() -> ("OldVal"=w1144:T1, "NewVal"=w1140:T1)  [unwired: 1 in]
            n285 = Cluster To Array(cluster=w1144) -> (array=w1143:bool[])
            n286 = Cluster To Array(cluster=w1140) -> (array=w1145:bool[])
            n287 = for {
              tunnel: w1145 -> [w1147] mode=indexing
              tunnel: w1143 -> [w1151] mode=indexing
              tunnel: w1142 -> [w1149]
              tunnel: w1141 -> [w1148]
              i -> [w1150]
              n288 = Equal?(x=w1151, y=w1147) -> (x = y?=w1146:bool)
              n289 = case shown="False" w1146 {
                tunnel: w1150 -> [_ w1161]
                tunnel: w1149 -> [_ w1165]
                tunnel: w1148 -> [_ w1164]
                tunnel: w1147 -> [_ w1152]
                frame True {
                }
                frame False {
                  w1159 = " " ("string")
                  # "What lamp is Fe?"
                  n290 = property on="Lamp Cluster" class="Clust (strict)"() -> ("Controls[]"=w1168:refnum<vi>[])  [unwired: 2 in, 2 out]
                  n291 = Index Array(array=w1168, index=w1161) -> (element=w1160:refnum<vi>)
                  n292 = property class="Ctl"(reference=w1160) -> ("Label.Text"=w1153:string)  [unwired: 1 in, 2 out]
                  n293 = case shown="True" w1152 {
                    tunnel: ["OFF" ("string") "ON" ("string")] -> w1157
                    frame False {
                    }
                    frame True {
                    }
                  }
                  n294 = case shown="\"Quartz\"" w1153 {
                    tunnel: ["" "" "" "" "" w1272 "" w1276] -> w1158
                    tunnel: ["L1" ("string") "L4" ("string") "L2" ("string") "L5" "L3" ("string") "L9" ("string") "L11" ("string") w1276] -> w1166
                    frame "Hg(Ar)" {
                    }
                    frame "Cu" {
                    }
                    frame "Ne" {
                    }
                    frame "Fe" {
                    }
                    frame "Ar" {
                    }
                    frame "Quartz" {
                      n295 = Number To Decimal String(number="Quartz Intensity") -> (decimal integer string=w1272:string)  [unwired: 1 in]
                    }
                    frame "Bulb" {
                    }
                    frame "", Default {
                      w1276 = ""
                    }
                  }
                  n296 = Concatenate Strings("LAMP", w1159, w1166, w1159, w1157, w1159, w1158) -> (w1156:string)
                  n297 = Enqueue Element(queue=w1165, element=w1156) -> ()  [unwired: 2 in, 3 out]
                  n298 = Dequeue Element(queue=w1164, timeout in ms (-1)=2000) -> (element=w1154:string)  [unwired: 1 in, 3 out]
                  n299 = Match Pattern(string=w1154, regular expression="DONE") -> (offset past match=w1162:i32)  [unwired: 1 in, 3 out]
                  n300 = case shown="-1" w1162 {
                    tunnel: w1160 -> [w1260 _]
                    frame -1 {
                      n301 = property class="Ctl"(reference=w1260) -> (reference out=w1255:refnum<vi>, "Value"=w1259:variant)  [unwired: 1 in, 1 out]
                      n302 = Variant To Data(type=TRUE, Variant=w1259) -> (data=w1258:bool)  [unwired: 1 in, 1 out]
                      n303 = Not(x=w1258) -> (.not. x?=w1257:bool)
                      n304 = property class="Ctl"(reference=w1255, "Value"=w1257) -> ()  [unwired: 1 in, 2 out]
                    }
                    frame 0, Default {
                    }
                  }
                  n305 = case shown="\"Quartz\"" w1153 {
                    tunnel: w1152 -> [w1170 w1181 _ w1193 w1205 w1217 w1229 w1241]
                    frame "Quartz" {
                      n306 = property on="Quartz Ind" class="Ring (strict)"("Value"=1) -> ()  [unwired: 2 in, 2 out]
                      n307 = Tick Count (ms)() -> (millisecond timer value=w1169:u32)
                      n308 = while {
                        tunnel: w1170 -> [w1179]
                        tunnel: w1169 -> [w1173]
                        stop <- w1175 stop-if-true
                        n309 = Tick Count (ms)() -> (millisecond timer value=w1174:u32)
                        n310 = global read "TCSLINK_global.vi" "Quartz"() -> (w1180:bool)
                        n311 = Add(x=w1173, y=10000) -> (x+y=w1172:u32)
                        n312 = Greater?(x=w1174, y=w1172) -> (0:w1176:bool)
                        n313 = Equal?(x=w1180, y=w1179) -> (x = y?=w1177:bool)
                        n314 = Or(x=w1177, y=w1176) -> (x .or. y?=w1175:bool)
                      }
                    }
                    frame "Bulb" {
                      n315 = property on="Bulb Ind" class="Ring (strict)"("Value"=1) -> ()  [unwired: 2 in, 2 out]
                      n316 = Tick Count (ms)() -> (millisecond timer value=w1182:u32)
                      n317 = while {
                        tunnel: w1181 -> [w1191]
                        tunnel: w1182 -> [w1185]
                        stop <- w1187 stop-if-true
                        n318 = Tick Count (ms)() -> (millisecond timer value=w1186:u32)
                        n319 = global read "TCSLINK_global.vi" "Bulb"() -> (w1192:bool)
                        n320 = Add(x=w1185, y=10000) -> (x+y=w1184:u32)
                        n321 = Greater?(x=w1186, y=w1184) -> (0:w1188:bool)
                        n322 = Equal?(x=w1192, y=w1191) -> (x = y?=w1189:bool)
                        n323 = Or(x=w1189, y=w1188) -> (x .or. y?=w1187:bool)
                      }
                    }
                    frame "", Default {
                    }
                    frame "Hg(Ar)" {
                      n324 = property on="Hg(Ar) Ind" class="Ring (strict)"("Value"=1) -> ()  [unwired: 2 in, 2 out]
                      n325 = Tick Count (ms)() -> (millisecond timer value=w1194:u32)
                      n326 = while {
                        tunnel: w1193 -> [w1203]
                        tunnel: w1194 -> [w1197]
                        stop <- w1199 stop-if-true
                        n327 = Tick Count (ms)() -> (millisecond timer value=w1198:u32)
                        n328 = global read "TCSLINK_global.vi" "Hg(Ar)"() -> (w1204:bool)
                        n329 = Add(x=w1197, y=10000) -> (x+y=w1196:u32)
                        n330 = Greater?(x=w1198, y=w1196) -> (0:w1200:bool)
                        n331 = Equal?(x=w1204, y=w1203) -> (x = y?=w1201:bool)
                        n332 = Or(x=w1201, y=w1200) -> (x .or. y?=w1199:bool)
                      }
                    }
                    frame "Cu" {
                      n333 = property on="Cu Ind" class="Ring (strict)"("Value"=1) -> ()  [unwired: 2 in, 2 out]
                      n334 = Tick Count (ms)() -> (millisecond timer value=w1206:u32)
                      n335 = while {
                        tunnel: w1205 -> [w1215]
                        tunnel: w1206 -> [w1209]
                        stop <- w1211 stop-if-true
                        n336 = Tick Count (ms)() -> (millisecond timer value=w1210:u32)
                        n337 = global read "TCSLINK_global.vi" "Cu"() -> (w1216:bool)
                        n338 = Add(x=w1209, y=10000) -> (x+y=w1208:u32)
                        n339 = Greater?(x=w1210, y=w1208) -> (0:w1212:bool)
                        n340 = Equal?(x=w1216, y=w1215) -> (x = y?=w1213:bool)
                        n341 = Or(x=w1213, y=w1212) -> (x .or. y?=w1211:bool)
                      }
                    }
                    frame "Ne" {
                      n342 = property on="Ne Ind" class="Ring (strict)"("Value"=1) -> ()  [unwired: 2 in, 2 out]
                      n343 = Tick Count (ms)() -> (millisecond timer value=w1218:u32)
                      n344 = while {
                        tunnel: w1217 -> [w1227]
                        tunnel: w1218 -> [w1221]
                        stop <- w1223 stop-if-true
                        n345 = Tick Count (ms)() -> (millisecond timer value=w1222:u32)
                        n346 = global read "TCSLINK_global.vi" "Ne"() -> (w1228:bool)
                        n347 = Add(x=w1221, y=10000) -> (x+y=w1220:u32)
                        n348 = Greater?(x=w1222, y=w1220) -> (0:w1224:bool)
                        n349 = Equal?(x=w1228, y=w1227) -> (x = y?=w1225:bool)
                        n350 = Or(x=w1225, y=w1224) -> (x .or. y?=w1223:bool)
                      }
                    }
                    frame "Fe" {
                      n351 = property on="Fe Ind" class="Ring (strict)"("Value"=1) -> ()  [unwired: 2 in, 2 out]
                      n352 = Tick Count (ms)() -> (millisecond timer value=w1230:u32)
                      n353 = while {
                        tunnel: w1229 -> [w1239]
                        tunnel: w1230 -> [w1233]
                        stop <- w1235 stop-if-true
                        n354 = Tick Count (ms)() -> (millisecond timer value=w1234:u32)
                        n355 = global read "TCSLINK_global.vi" "Fe"() -> (w1240:bool)
                        n356 = Add(x=w1233, y=10000) -> (x+y=w1232:u32)
                        n357 = Greater?(x=w1234, y=w1232) -> (0:w1236:bool)
                        n358 = Equal?(x=w1240, y=w1239) -> (x = y?=w1237:bool)
                        n359 = Or(x=w1237, y=w1236) -> (x .or. y?=w1235:bool)
                      }
                    }
                    frame "Ar" {
                      n360 = property on="Ar Ind" class="Ring (strict)"("Value"=1) -> ()  [unwired: 2 in, 2 out]
                      n361 = Tick Count (ms)() -> (millisecond timer value=w1242:u32)
                      n362 = while {
                        tunnel: w1241 -> [w1251]
                        tunnel: w1242 -> [w1245]
                        stop <- w1247 stop-if-true
                        n363 = Tick Count (ms)() -> (millisecond timer value=w1246:u32)
                        n364 = global read "TCSLINK_global.vi" "Ar"() -> (w1252:bool)
                        n365 = Add(x=w1245, y=10000) -> (x+y=w1244:u32)
                        n366 = Greater?(x=w1246, y=w1244) -> (0:w1248:bool)
                        n367 = Equal?(x=w1252, y=w1251) -> (x = y?=w1249:bool)
                        n368 = Or(x=w1249, y=w1248) -> (x .or. y?=w1247:bool)
                      }
                    }
                  }
                }
              }
            }
          }
          event "Quartz Intensity": Value Change {
            n369 = event-data() -> ("OldVal"=w1283:i8, "NewVal"=w1278:i8)  [unwired: 1 in, 4 out]
            n370 = Equal?(x=w1283, y=w1278) -> (x = y?=w1282:bool)
            n371 = case shown="False" w1282 {
              tunnel: w1281 -> [w1304 _]
              tunnel: w1280 -> [w1303 _]
              tunnel: w1278 -> [w1293 _]
              frame False {
                w1301 = " " ("string")
                n372 = Number To Decimal String(number=w1293) -> (decimal integer string=w1297:string)  [unwired: 1 in]
                n373 = Concatenate Strings("LAMP", w1301, "L9", w1301, "ON", w1301, w1297) -> (w1300:string)
                n374 = Enqueue Element(queue=w1304, element=w1300) -> ()  [unwired: 2 in, 3 out]
                n375 = Dequeue Element(queue=w1303, timeout in ms (-1)=2000) -> (element=w1295:string)  [unwired: 1 in, 3 out]
                n376 = Match Pattern(string=w1295, regular expression="DONE") -> ()  [unwired: 1 in, 4 out]
              }
              frame True {
              }
            }
            n377 = Tick Count (ms)() -> (millisecond timer value=w1279:u32)
            n378 = property on="Quartz Ind" class="Ring (strict)"("Value"=1) -> ()  [unwired: 2 in, 2 out]
            n379 = while {
              tunnel: w1278 -> [w1291]
              tunnel: w1279 -> [w1284]
              stop <- w1287 stop-if-true
              n380 = global read "TCSLINK_global.vi" "Quartz Percent"() -> (w1292:i8)
              n381 = Tick Count (ms)() -> (millisecond timer value=w1286:u32)
              n382 = Add(x=w1284, y=10000) -> (x+y=w1285:u32)
              n383 = Greater?(x=w1286, y=w1285) -> (0:w1288:bool)
              n384 = Equal?(x=w1292, y=w1291) -> (x = y?=w1289:bool)
              n385 = Or(x=w1289, y=w1288) -> (x .or. y?=w1287:bool)
            }
          }
          event "Dome Set Percent": Value Change {
            n386 = event-data() -> ("OldVal"=w1309:i32, "NewVal"=w1305:i32)  [unwired: 1 in, 4 out]
            n387 = Equal?(x=w1309, y=w1305) -> (x = y?=w1308:bool)
            n388 = case shown="False" w1308 {
              tunnel: w1311 -> [w1331 _]
              tunnel: w1310 -> [w1330 _]
              tunnel: w1305 -> [w1321 _]
              frame False {
                w1329 = " " ("string")
                n389 = Number To Decimal String(number=w1321) -> (decimal integer string=w1325:string)  [unwired: 1 in]
                n390 = Concatenate Strings("WHITESPOT", w1329, "ON", w1329, w1325) -> (w1328:string)
                n391 = Enqueue Element(queue=w1331, element=w1328) -> ()  [unwired: 2 in, 3 out]
                n392 = Dequeue Element(queue=w1330, timeout in ms (-1)=2000) -> (element=w1323:string)  [unwired: 1 in, 3 out]
                n393 = Match Pattern(string=w1323, regular expression="DONE") -> ()  [unwired: 1 in, 4 out]
              }
              frame True {
              }
            }
            n394 = property on="Dome Ind" class="Ring (strict)"("Value"=1) -> ()  [unwired: 2 in, 2 out]
            n395 = Tick Count (ms)() -> (millisecond timer value=w1307:u32)
            n396 = while {
              tunnel: w1305 -> [w1319]
              tunnel: w1307 -> [w1312]
              stop <- w1315 stop-if-true
              n397 = Tick Count (ms)() -> (millisecond timer value=w1314:u32)
              n398 = global read "TCSLINK_global.vi" "Dome Percent"() -> (w1320:i8)
              n399 = Add(x=w1312, y=5000) -> (x+y=w1313:u32)
              n400 = Greater?(x=w1314, y=w1313) -> (0:w1316:bool)
              n401 = Equal?(x=w1320, y=w1319) -> (x = y?=w1317:bool)
              n402 = Or(x=w1317, y=w1316) -> (x .or. y?=w1315:bool)
            }
          }
          event "Dome": Value Change {
            n403 = event-data() -> ("NewVal"=w1332:bool)  [unwired: 1 in, 5 out]
            n404 = case shown="True" w1332 {
              tunnel: w1336 -> [w1347 w1358]
              tunnel: w1335 -> [w1346 w1357]
              frame False {
                w1353 = " " ("string")
                n405 = Concatenate Strings("WHITESPOT", w1353, "OFF", w1353) -> (w1352:string)
                n406 = Enqueue Element(queue=w1347, element=w1352) -> ()  [unwired: 2 in, 3 out]
                n407 = Dequeue Element(queue=w1346, timeout in ms (-1)=2000) -> (element=w1349:string)  [unwired: 1 in, 3 out]
                n408 = Match Pattern(string=w1349, regular expression="DONE") -> ()  [unwired: 1 in, 4 out]
              }
              frame True {
                w1364 = " " ("string")
                n409 = local read "Dome Set Percent"() -> (w1355:i32)
                n410 = Number To Decimal String(number=w1355) -> (decimal integer string=w1356:string)  [unwired: 1 in]
                n411 = Concatenate Strings("WHITESPOT", w1364, "ON", w1364, w1356) -> (w1363:string)
                n412 = Enqueue Element(queue=w1358, element=w1363) -> ()  [unwired: 2 in, 3 out]
                n413 = Dequeue Element(queue=w1357, timeout in ms (-1)=2000) -> (element=w1360:string)  [unwired: 1 in, 3 out]
                n414 = Match Pattern(string=w1360, regular expression="DONE") -> ()  [unwired: 1 in, 4 out]
              }
            }
            n415 = property on="Dome Ind" class="Ring (strict)"("Value"=1) -> ()  [unwired: 2 in, 2 out]
            n416 = Tick Count (ms)() -> (millisecond timer value=w1333:u32)
            n417 = while {
              tunnel: w1332 -> [w1344]
              tunnel: w1333 -> [w1337]
              stop <- w1340 stop-if-true
              n418 = Tick Count (ms)() -> (millisecond timer value=w1339:u32)
              n419 = global read "TCSLINK_global.vi" "Dome"() -> (w1345:bool)
              n420 = Add(x=w1337, y=5000) -> (x+y=w1338:u32)
              n421 = Greater?(x=w1339, y=w1338) -> (0:w1341:bool)
              n422 = Equal?(x=w1345, y=w1344) -> (x = y?=w1342:bool)
              n423 = Or(x=w1342, y=w1341) -> (x .or. y?=w1340:bool)
            }
          }
          event "Reset Wavelength Angles System": Value Change {
            n424 = event-data() -> ()  [unwired: 1 in, 6 out]
            n425 = Two Button Dialog(message="ARE YOU SURE you want to stop camera motion? ", 2:"YES" ("T button name (\"OK\")")) -> (T button?=w1369:bool)  [unwired: 1 in]
            n426 = case shown="True" w1369 {
              tunnel: w1373 -> [w1374 w1379]
              tunnel: [w1374 w1378] -> w1372
              tunnel: FALSE ("Reset Wavelength Angles System") -> [w1375 w1383]
              tunnel: [w1375 w1383] -> w1367
              frame False {
              }
              frame True {
                n427 = Obtain Queue(name (unnamed)="WL_Command_Q", element data type=T7 {"Command"="", "Parameter"=""} ("Command"), error in (no error)=w1379) -> (queue out=w1377:refnum<queue>, error out=w1382:errorcluster)  [unwired: 2 in, 1 out]
                n428 = Enqueue Element(queue=w1377, element=T7 {"Command"="STOP_CAMERA_MOTION", "Parameter"=""}, error in (no error)=w1382) -> (error out=w1378:errorcluster)  [unwired: 1 in, 2 out]
              }
            }
            n429 = local write "Reset Wavelength Angles System"(w1367) -> ()
            n430 = local write "Current Status"("Camera Rotation Stopped" ("Current Status")) -> ()
          }
          event "Start Exposure": Value Change {
            w1385 = TRUE ("Exposure Active?")
            # "Software versions"
            # "Gather information for FITS header file, change 'Exposure Acxtive?' to start image-taking sequence in 'POLL'"
            n431 = event-data() -> ()  [unwired: 1 in, 1 out]
            n432 = case shown="\"Blue\"" w1387 {
              tunnel: ["Si 600-658 " "Si 1110-111"] -> w1386
              frame "Blue" {
              }
              frame "Red", Default {
              }
            }
            n433 = case shown="\"Focus\"" "Exposure Tab" {
              tunnel: "Exp. Time (s)" -> [w1429 w1436 w1443 w1449 w1452 w1461]
              tunnel: [w1429 w1436 w1443 w1449 w1452 w1461] -> w1404
              tunnel: ["# Dark Exposures" "# Zero Exposures" "# Exposures" "# Focus Steps" "# Comp Exposures" "# Flat Exposures"] -> w1403
              tunnel: ["Dark Comments:" "Zero Comments:" "Object Comments:" "Focus Name" "Comp Comments:" ""] -> w1409
              tunnel: ["DARK" ("Object Name:") "ZERO" ("Object Name:") "Object Name:" "Focus Name" "Comp Name:" "Flat Name:"] -> w1410
              tunnel: [w1425 w1432 w1439 w1448 w1454 w1463] -> w1405
              tunnel: ["DARK" ("Other Info..OBSTYPE") "BIAS" ("Other Info..OBSTYPE") "OBJECT" ("Other Info..OBSTYPE") "FOCUS" ("Other Info..OBSTYPE") "COMP" ("Other Info..OBSTYPE") "FLAT" ("Other Info..OBSTYPE")] -> w1397
              tunnel: [TRUE TRUE TRUE FALSE TRUE TRUE] -> w1384
              frame "Dark" {
                w1425 = i16 0 items=["Dark", "Light"] ("Exposure type")
              }
              frame "Zero" {
                w1432 = i16 0 items=["Dark", "Light"] ("Exposure type")
              }
              frame "Object" {
                w1439 = i16 1 items=["Dark", "Light"] ("Exposure type")
              }
              frame "Focus" {
                w1448 = i16 1 items=["Dark", "Light"] ("Exposure type")
              }
              frame "Comp" {
                w1454 = i16 1 items=["Dark", "Light"] ("Exposure type")
              }
              frame "Flat" {
                w1463 = i16 1 items=["Dark", "Light"] ("Exposure type")
              }
            }
            n434 = local write "Focus Changed?"(w1384) -> ()
            n435 = call "GetTCSInfo.vi"() -> ("TCSInfo"=w1398:T15)
            n436 = call "GetSystemsInfo.vi"() -> ("Pos Info"=w1396:T16)
            n437 = Bundle By Name(cluster=T8 {"Object Name"="", "Telescope"="", "Instrument"="", "Comment"="", "\nINSTCONF"="", "CAMSWV"="", "CONSWV"="", "INSTSWV"="", "CAMERA"=""} ("input cluster"), "Object Name"=w1410, "Telescope"="SOAR 4.1m", "Comment"=w1409, "Instrument"="Goodman Spectro", "INSTCONF"=w1387, "CAMSWV"="Beta 29", "CONSWV"="8359,10", "INSTSWV"=w1389, "CAMERA"=w1386) -> (w1392:T8)
            n438 = call "GetComponentNames.vi"() -> ("Component Names"=w1395:T17)
            n439 = local read "Has Red switch been run"() -> (w1388:bool)
            n440 = Tick Count (ms)() -> (millisecond timer value=w1400:u32)
            n441 = case shown="False" w1388 {
              tunnel: w1387 -> [_ w1416]
              frame True {
              }
              frame False {
                n442 = case shown="\"Red\"" w1416 {
                  frame "Blue", Default {
                  }
                  frame "Red" {
                    n443 = local write "Has Red switch been run"(TRUE) -> ()
                    n444 = Number To Decimal String(number=600) -> (decimal integer string=w1421:string)  [unwired: 1 in]
                    n445 = Build Array(w1421) -> (w1419:string[])
                    n446 = call "gsp_silvermax_commandreponse.vi"("Parameters (none)"=w1419, "Motor #"=u8 40, "Command"=T9."LRP (156)") -> ()  [unwired: 1 in, 4 out]
                  }
                }
              }
            }
            n447 = Bundle By Name(cluster=w1402, "Obs parameters"=w1392, "Current Exposure"=1, "Exposure type"=w1405, "Exposure Active?"=w1385, "#Exposures"=w1403, "Exposure Time"=w1404, "TCSInfo"=w1398, "System Pos Info"=w1396, "Component Names"=w1395, "Last Exposure Start Time"=w1400, "Other Info..OBSTYPE"=w1397, "Other Info..OBSERVER"="Observer Name", "Other Info..Proposal #"="Proposal #") -> (w1412:T6)
            n448 = local write "Script"(w1412) -> ()
            n449 = global write "SIcamera_Globals.vi" "Exposure Active?"(w1385) -> ()
          }
          event "Show Images?": Value Change {
            n450 = event-data() -> ("NewVal"=w1468:bool)  [unwired: 1 in]
            n451 = Current VI's Path() -> (path=w1465:path)
            n452 = Strip Path(path=w1465) -> (stripped path=w1466:path)  [unwired: 1 out]
            n453 = Build Path(base path=w1466, name or relative path="Quick_Look\\Quick_Look.vi") -> (appended path=w1464:path)
            n454 = case shown="False" w1468 {
              tunnel: w1464 -> [_ w1479]
              frame False {
                n455 = Obtain Queue(name (unnamed)="QUICKLOOK_Q", element data type=T7 {"Command"="", "Parameter"=""} ("element")) -> (queue out=w1475:refnum<queue>, error out=w1474:errorcluster)  [unwired: 3 in, 1 out]
                n456 = Enqueue Element(queue=w1475, element=T7 {"Command"="SHUTDOWN", "Parameter"=""}, error in (no error)=w1474) -> (queue out=w1472:refnum<queue>, error out=w1471:errorcluster)  [unwired: 1 in, 1 out]
                n457 = Release Queue(queue=w1472, error in (no error)=w1471) -> ()  [unwired: 1 in, 3 out]
              }
              frame True {
                n458 = Open VI Reference(vi path=w1479) -> (vi reference=w1480:refnum<vi>)  [unwired: 5 in, 1 out]
                n459 = invoke class="VI" method="FP.Open"(reference=w1480) -> (reference out=w1478:refnum<vi>)  [unwired: 4 in, 4 out]
                n460 = invoke class="VI" method="Run VI"(reference=w1478, "Wait until done"=FALSE) -> (reference out=w1476:refnum<vi>)  [unwired: 3 in, 4 out]
                n461 = Close Reference(reference=w1476) -> ()  [unwired: 1 in, 1 out]
              }
            }
          }
          event "Take Thumbnail": Value Change {
            w1496 = u16 1 items=["Retrieve Image Buffer", "Acquire and transfer to client", "Acquire and hold in Server Image Buffer", "Acquire, transfer to client, and save to Server's disk", "Acquire, save to Server's disk, and hold in Server Image Buffer"] ("Mode")
            w1485 = 1 ("Current Exposure")
            # "Transfer instead of save"
            n462 = event-data() -> ()  [unwired: 1 in, 1 out]
            n463 = case shown="\"Check Entire CCD\", Default" "Thumbnail Setting" {
              tunnel: [w1508 w1514] -> w1490
              frame "Check Entire CCD", Default {
                w1507 = 32 ("element")
                # "Take current ROI, bin by 4"
                n464 = local read "Port Readout"() -> (w1501:u16)
                n465 = Greater Than 0?(x=w1501) -> (x > 0?=w1502:bool)
                n466 = Select(t=128 ("element"), s=w1502, f=64 ("element")) -> (s? t:f=w1500:i32)
                n467 = Bundle("element"=16, "element"=w1500, "element"=w1507, "element"=0, "element"=w1500, "element"=w1507) -> (w1508:T18)  [unwired: 1 in]
              }
              frame "Check Star Focus" {
                w1509 = 1 ("element")
                n468 = Bundle("element"=1964, "element"=200, "element"=w1509, "element"=1948, "element"=200, "element"=w1509) -> (w1514:T18)  [unwired: 1 in]
              }
            }
            n469 = local read "Exposure Tab"() -> (w1484:T2)
            n470 = case shown="\"Object\", Default" w1484 {
              tunnel: [w1497 w1498 w1499] -> w1483
              frame "Object", Default {
                w1497 = i16 1 items=["Dark", "Light"] ("Exposure type")
              }
              frame "Zero" {
                w1498 = i16 0 items=["Dark", "Light"] ("Exposure type")
              }
              frame "Dark" {
                w1499 = i16 0 items=["Dark", "Light"] ("Exposure type")
              }
            }
            n471 = property on="Mode" class="Ring (strict)"("Value"=w1496) -> ()  [unwired: 2 in, 2 out]
            n472 = local read "Exp. Time (s)"() -> (w1482:dbl)
            n473 = local write "Current Status"("Acquiring thumbnail of CCD image..." ("Current Status")) -> ()
            n474 = Bundle By Name(cluster=w1488, "Exposure Active?"=TRUE, "Current Exposure"=w1485, "#Exposures"=w1485, "Exposure type"=w1483, "Exposure Time"=w1482) -> (w1486:T6)
            n475 = local write "Script"(w1486) -> ()
            n476 = call "Send Single TCP-IP Cmd 1.vi"("TCP/IP ID"=w1489, "Camera Color"=w1481, "Function #"=u16 1043, "Camera ID"=u8 1, "CCD Format Parameters"=w1490) -> ("Error Out"=w1494:errorcluster)  [unwired: 11 in, 3 out]
            n477 = call "SI Image Error Handler - Win 2.vi"("error in (no error)"=w1494) -> ()  [unwired: 4 in, 1 out]
          }
          event "MOS": Value Change {
            n478 = event-data() -> ("NewVal"=w1515:bool)  [unwired: 1 in]
            n479 = Current VI's Path() -> (path=w1517:path)
            n480 = Strip Path(path=w1517) -> (stripped path=w1518:path)  [unwired: 1 out]
            n481 = Build Path(base path=w1518, name or relative path="Quick_Look\\MultiSlit_Graphical.vi") -> (appended path=w1516:path)
            n482 = case shown="True" w1515 {
              tunnel: w1516 -> [_ w1530]
              frame False {
                n483 = Obtain Queue(name (unnamed)="MULTISLIT_Q", element data type=T7 {"Command"="", "Parameter"=""} ("element")) -> (queue out=w1526:refnum<queue>, error out=w1525:errorcluster)  [unwired: 3 in, 1 out]
                n484 = Enqueue Element(queue=w1526, element=T7 {"Command"="SHUTDOWN", "Parameter"=""}, error in (no error)=w1525) -> (queue out=w1523:refnum<queue>, error out=w1522:errorcluster)  [unwired: 1 in, 1 out]
                n485 = Release Queue(queue=w1523, error in (no error)=w1522) -> ()  [unwired: 1 in, 3 out]
              }
              frame True {
                n486 = Open VI Reference(vi path=w1530) -> (vi reference=w1531:refnum<vi>)  [unwired: 5 in, 1 out]
                n487 = invoke class="VI" method="FP.Open"(reference=w1531) -> (reference out=w1529:refnum<vi>)  [unwired: 4 in, 4 out]
                n488 = invoke class="VI" method="Run VI"(reference=w1529, "Wait until done"=FALSE) -> (reference out=w1527:refnum<vi>)  [unwired: 3 in, 4 out]
                n489 = Close Reference(reference=w1527) -> ()  [unwired: 1 in, 1 out]
              }
            }
          }
          event "Observer Name": Value Change {
            n490 = event-data() -> ()  [unwired: 1 in, 6 out]
            n491 = local read "Observer Name"() -> (w1536:string)
            n492 = Search and Replace String(input string=w1536, search string="'") -> (offset past replacement=w1534:i32)  [unwired: 6 in, 3 out]
            n493 = Equal?(x=w1534, y=-1) -> (x = y?=w1532:bool)
            n494 = case shown="False" w1532 {
              frame False {
                n495 = call "Display Message to User"() -> ()  [unwired: 10 in, 2 out]
              }
              frame True {
              }
            }
          }
          event "Offset Telescope": Value Change {
            w1547 = " " ("string")
            w1552 = "%1.2f" ("format string")
            w1557 = 1 ("length (rest)")
            # "Send offset command to TCS, obtain response from TCS"
            n496 = event-data() -> ()  [unwired: 1 in, 1 out]
            n497 = property on="E/W Offset Choice" class="Ring (strict)"() -> ("Ring Text.Text"=w1555:string)  [unwired: 2 in, 2 out]
            n498 = property on="N/S Offset Choice" class="Ring (strict)"() -> ("Ring Text.Text"=w1556:string)  [unwired: 2 in, 2 out]
            n499 = Format Value(format string=w1552, value (0)="E/W Offset") -> (output string=w1549:string)  [unwired: 1 in]
            n500 = Format Value(format string=w1552, value (0)="N/S Offset") -> (output string=w1546:string)  [unwired: 1 in]
            n501 = String Subset(string=w1555, length (rest)=w1557) -> (substring=w1553:string)  [unwired: 1 in]
            n502 = String Subset(string=w1556, length (rest)=w1557) -> (substring=w1548:string)  [unwired: 1 in]
            n503 = Concatenate Strings("OFFSET MOVE ", w1553, w1547, w1549, w1547, w1548, w1547, w1546) -> (w1541:string)
            n504 = Enqueue Element(queue=w1543, element=w1541) -> (error out=w1545:errorcluster)  [unwired: 2 in, 2 out]
            n505 = Dequeue Element(queue=w1542, timeout in ms (-1)=2000, error in (no error)=w1545) -> (element=w1539:string)  [unwired: 3 out]
            n506 = Concatenate Strings("TCS: " ("string"), w1539) -> (w1538:string)
            n507 = flat-sequence {
              tunnel: w1538 -> [_]
              tunnel: ["Applying SOAR offset..."] -> w1537
              frame #0 {
                w1559 = 0.0 ("E/W Offset")
                n508 = local write "Offset Telescope"(FALSE ("Offset Telescope")) -> ()
                n509 = local write "E/W Offset"(w1559) -> ()
                n510 = local write "N/S Offset"(w1559) -> ()
              }
            }
            n511 = local write "Current Status"(w1537) -> ()
          }
          event "Reset TCP": Value Change {
            n512 = event-data() -> ()  [unwired: 1 in, 1 out]
            n513 = Enqueue Element(queue=w1568, element=T7 {"Command"="INIT_TCP", "Parameter"=""}, error in (no error)=w1567) -> (error out=w1564:errorcluster)  [unwired: 1 in, 2 out]
            n514 = TCP Close Connection(connection ID=w1569, error in (no error)=w1564) -> (error out=w1563:errorcluster)  [unwired: 1 in, 1 out]
            n515 = local write "Connection Status"(FALSE ("Connection Status")) -> ()
            n516 = local write "Reset TCP"(FALSE ("Reset TCP")) -> ()
            n517 = local write "Current Status"("Resetting TCP/IP connection..." ("Current Status")) -> ()
          }
          event "SHUTDOWN": Value Change {
            n518 = event-data() -> ()  [unwired: 1 in, 1 out]
            n519 = Enqueue Element(queue=w1573, element=T7 {"Command"="SHUTDOWN", "Parameter"=""}, error in (no error)=w1572) -> (error out=w1571:errorcluster)  [unwired: 1 in, 2 out]
          }
        }
      }
      frame "ACCEPT_OFFSET_COORD" {
        w1576 = 0.0 ("sx1")
        w1574 = "%.1f" ("format string")
        w1580 = " " ("regular expression")
        n520 = Match Pattern(string=w1584, regular expression=w1580) -> (before substring=w1582:string, after substring=w1583:string)  [unwired: 1 in, 2 out]
        n521 = Match Pattern(string=w1583, regular expression=w1580) -> (before substring=w1579:string, after substring=w1577:string)  [unwired: 1 in, 2 out]
        n522 = Scan Value(string=w1579, format string=w1574, default (0 dbl)=w1576) -> (value=w1578:dbl)  [unwired: 1 out]
        n523 = Scan Value(string=w1577, format string=w1574, default (0 dbl)=w1576) -> (value=w1575:dbl)  [unwired: 1 out]
        n524 = case shown="\"O\"" w1582 {
          tunnel: w1578 -> [w1585 _ w1588]
          tunnel: w1575 -> [w1586 _ w1587]
          frame "O" {
            n525 = local write "ox1"(w1585) -> ()
            n526 = local write "oy1"(w1586) -> ()
          }
          frame Default {
          }
          frame "T" {
            n527 = local write "sx1"(w1588) -> ()
            n528 = local write "sy1"(w1587) -> ()
          }
        }
      }
      frame "INIT_TCP" {
        # "Establish TCP/ID connection with camera server; try again until connection sucessful."
        n529 = global write "SIcamera_Globals.vi" "Color"(w1589) -> ()
        n530 = case shown="\"Red\", Default" w1589 {
          tunnel: [w1604 w1608] -> w1593
          tunnel: w1592 -> [w1603 w1607]
          tunnel: [w1602 w1606] -> w1591
          frame "Red", Default {
            n531 = TCP Open Connection(address="Localhost", remote port or service name=u16 2055, error in (no error)=w1603) -> (connection ID=w1604:refnum<k5>, error out=w1602:errorcluster)  [unwired: 2 in]
          }
          frame "Blue" {
            # "Ip address of blue computer"
            n532 = TCP Open Connection(address="Localhost", remote port or service name=2055, error in (no error)=w1607) -> (connection ID=w1608:refnum<k5>, error out=w1606:errorcluster)  [unwired: 2 in]
          }
        }
        "TCP/IP ID" <- w1593
        n533 = Unbundle By Name(w1591) -> ("status"=w1595:bool)
        n534 = case shown="True" w1595 {
          tunnel: w1597 -> [w1614 w1618]
          tunnel: ["TCP/IP connection established..." ("Current Status") "Trying to establish TCP/IP connection..." ("Current Status")] -> w1594
          frame False {
            n535 = Enqueue Element(queue=w1614, element=T7 {"Command"="INIT_CAMERA", "Parameter"=""}) -> (queue out=w1612:refnum<queue>)  [unwired: 2 in, 2 out]
            n536 = Enqueue Element(queue=w1612, element=T7 {"Command"="ENABLE_CONTROLS", "Parameter"=""}) -> ()  [unwired: 2 in, 3 out]
          }
          frame True {
            n537 = Enqueue Element(queue=w1618, element=T7 {"Command"="INIT_TCP", "Parameter"=""}) -> ()  [unwired: 2 in, 3 out]
          }
        }
        n538 = Not(x=w1595) -> (.not. x?=→"Connection Status":bool)
        n539 = case shown="\"Red\", Default" w1589 {
          frame "Blue" {
            n540 = property on="CCD Readout Speed" class="Ring (strict)"("Strings []"=string[] ["50 kHz, ATTN 0", "50 kHz, ATTN 2", "50 kHz, ATTN 3", "100 kHz, ATTN 0", "100 kHz, ATTN 2", "100 kHz, ATTN 3", "200 kHz, ATTN 0", "200 kHz, ATTN 2", "400 kHz, ATTN 0"]) -> ()  [unwired: 2 in, 2 out]
          }
          frame "Red", Default {
            n541 = property on="CCD Readout Speed" class="Ring (strict)"("Strings []"=string[] ["750 kHz, ATTN 0", "750 kHz, ATTN 2", "344 kHz, ATTN 0", "344 kHz, ATTN 3", "100 kHz, ATTN 2", "100 kHz, ATTN 3"]) -> ()  [unwired: 2 in, 2 out]
          }
        }
        n542 = local write "Current Status"(w1594) -> ()
        n543 = Wait (ms)(milliseconds to wait=u32 100) -> ()  [unwired: 1 out]
      }
      frame "INIT_CAMERA" {
        w1624 = FALSE
        w1629 = u16 2 items=["4-port", "Port A", "Port B", "Port C", "Port D"] ("Port Readout")
        w1620 = 1.0 ("Exp. Time (s)")
        w1642 = u8 5 items=["50 kHz, ATTN 0", "50 kHz, ATTN 2", "50 kHz, ATTN 3", "100 kHz, ATTN 0", "100 kHz, ATTN 2", "100 kHz, ATTN 3", "200 kHz, ATTN 0", "200 kHz, ATTN 2", "400 kHz, ATTN 0"] ("CCD Readout Speed")
        w1643 = u16 0 items=["Imaging, 1x1  ", "Imaging, 2x2", "Spectroscopic, 1x1", "Spectroscopic, 2x2", "Focus (Imag.)", "Focus (Spect.)", "Slicer", "Slit Imaging/Alignment", "Set user-defined ROI...", "Custom Mode"] ("CCD ROI Mode")
        # "4/12/17 - we are not manually setting the port, \nwe are changing the readout speeds and this \nwill map the gain and read noise."
        # "Upon startup, set acquisition mode to \"Triggered Acquisition\""
        # "Upon startup, set tab to \"object\" , set exp time to 1sec."
        # "=100kHz ATTN3"
        # "Upon startup, set to Port B; proper gain and RDnoise for Port B, 100 kHz  ATTN 3 are default values in script"
        n544 = invoke on="Script" class="Clust (strict)" method="Reinit To Default"(error in=w1641) -> (error out=w1640:errorcluster)  [unwired: 2 in, 2 out]
        n545 = case shown="\"Red\", Default" w1625 {
          tunnel: w1645 -> [w1666 w1667]
          tunnel: w1640 -> [w1665 w1668]
          tunnel: [w1665 w1668] -> w1632
          tunnel: [w1666 w1667] -> w1631
          frame "Red", Default {
            n546 = property on="CCD Readout Speed" class="Ring (strict)"("Val(Sgnl)"=3) -> ()  [unwired: 2 in, 2 out]
          }
          frame "Blue" {
            # "=100kHz ATTN3\non Port B"
            n547 = property on="CCD Readout Speed" class="Ring (strict)"("Val(Sgnl)"=3) -> ()  [unwired: 2 in, 2 out]
          }
        }
        n548 = local write "Exp. Time (s)"(w1620) -> ()
        n549 = local write "Port Readout"(w1629) -> ()
        n550 = property on="Readout left" class="DigNum (strict)"("Visible"=w1624) -> ()  [unwired: 2 in, 2 out]
        n551 = property on="Port Readout" class="Ring (strict)"("Visible"=FALSE) -> ()  [unwired: 2 in, 2 out]
        n552 = property on="Exp time left" class="DigNum (strict)"("Visible"=w1624) -> ()  [unwired: 2 in, 2 out]
        n553 = local read "CCD ROI"() -> (w1639:cluster{i32, i32, i32, i32, i32, i32})
        n554 = local write "Exposure Tab"(enum32{"Object", "Flat", "Comp", "Dark", "Zero"}."Object" ("Exposure Tab")) -> ()
        n555 = call "CalculateCCDReadoutTime.vi"("Color"=w1625, "Readout Speed"=5.0 ("Acq. Mode/Type/Frame Mode/RO Mode #"), "CCD ROI"=w1639) -> ("Readout Time"=w1638:dbl)
        n556 = local write "CCD Readout Speed"(w1642) -> ()
        n557 = local write "CCD ROI Mode"(w1643) -> ()
        n558 = Multiply(x=w1620, y=1000.0) -> (x*y=w1622:dbl)
        n559 = global write "GPS_Driver_Global.vi" "ExpTime"(w1622) -> ()
        n560 = local write "Readout Time"(w1638) -> ()
        n561 = call "StartPCI.vi"("Device Number"=0) -> ()  [unwired: 5 in, 1 out]
        n562 = call "Send Single TCP-IP Cmd 1.vi"("TCP/IP ID"=w1631, "Exposure Time (ms)"=u32 1000, "Camera Color"=w1625, "Error In"=w1632, "Function #"=u16 1035, "Camera ID"=u8 0) -> ("TCP/IP ID Out"=w1626:refnum<k5>, "Error Out"=w1635:errorcluster)  [unwired: 10 in, 2 out]
        n563 = call "SI Image Error Handler - Win 2.vi"("error in (no error)"=w1635) -> ("error out"=w1628:errorcluster)  [unwired: 4 in]
        n564 = case shown="\"Red\", Default" w1625 {
          selector: w1625 -> [w1651 w1657]
          tunnel: w1628 -> [w1649 w1660]
          tunnel: [w1648 w1659] -> w1627
          tunnel: w1626 -> [w1650 w1658]
          frame "Blue" {
            n565 = To Unsigned Byte Integer(number=u8 2) -> (unsigned 8bit integer=w1646:u8)
            n566 = call "Send Single TCP-IP Cmd 1.vi"("TCP/IP ID"=w1650, "Camera Color"=w1651, "Error In"=w1649, "Function #"=u16 1036, "Camera ID"=u8 1, "Acq. Mode/Type/Frame Mode/RO Mode #"=w1646) -> ("Error Out"=w1654:errorcluster)  [unwired: 10 in, 3 out]
            n567 = call "SI Image Error Handler - Win 2.vi"("error in (no error)"=w1654) -> ("error out"=w1648:errorcluster)  [unwired: 4 in]
          }
          frame "Red", Default {
            n568 = To Unsigned Byte Integer(number=u8 0) -> (unsigned 8bit integer=w1655:u8)
            n569 = call "Send Single TCP-IP Cmd 1.vi"("TCP/IP ID"=w1658, "Camera Color"=w1657, "Error In"=w1660, "Function #"=u16 1036, "Camera ID"=u8 1, "Acq. Mode/Type/Frame Mode/RO Mode #"=w1655) -> ("Error Out"=w1663:errorcluster)  [unwired: 10 in, 3 out]
            n570 = call "SI Image Error Handler - Win 2.vi"("error in (no error)"=w1663) -> ("error out"=w1659:errorcluster)  [unwired: 4 in]
          }
        }
        "Has Red switch been run" <- FALSE
      }
      frame "POLL" {
        n571 = Unbundle By Name(w1678) -> ("Exposure Active?"=w1679:bool)
        n572 = local read "Current Status"() -> (w1672:string)
        n573 = case shown="\"Changing CCD readout speed...\"" w1672 {
          selector: w1672 -> [w1682 _ _ _ _ _ _]
          tunnel: [w1682 "DONE: SOAR offset applied" ("Current Status") "DONE: Camera status updated" ("Current Status") "DONE: CCD readout speed changed" ("Current Status") "DONE: Waiting for next command" ("Current Status") "DONE:  New ROI mode set" ("Current Status") "DONE: CCD port readout mode set" ("Current Status")] -> w1673
          frame "", Default {
          }
          frame "Applying SOAR offset..." {
          }
          frame "Getting camera status..." {
          }
          frame "Changing CCD readout speed..." {
          }
          frame "Finalizing acquisition..." {
          }
          frame "Setting new ROI mode..." {
          }
          frame "Changing CCD port readout mode..." {
          }
        }
        n574 = local write "Current Status"(w1673) -> ()
        n575 = case shown="False" w1679 {
          tunnel: w1678 -> [_ w1757]
          tunnel: w1677 -> [_ w1756]
          tunnel: w1675 -> [w1696 w1755]
          tunnel: [w1694 w1754] -> w1676
          tunnel: w1674 -> [w1695 w1753]
          frame False {
            # "Dome Percent"
            # "quartz percent"
            n576 = case shown="False" "Get Camera Status" {
              tunnel: w1696 -> [w1745 w1751]
              tunnel: w1695 -> [_ w1750]
              tunnel: [w1745 w1749] -> w1694
              frame False {
              }
              frame True {
                n577 = call "GetCameraStatus.vi"("TCP/IP ID"=w1750, "error in (no error)"=w1751) -> ("CCD temp"=→"CCD Temp.":string, "Vacuum Pressure"=→"Vacuum Pressure":string, "error out"=w1749:errorcluster)  [unwired: 1 in, 1 out]
                n578 = property on="Get Camera Status" class="Bool (strict)"("Value"=FALSE ("Get Camera Status")) -> ()  [unwired: 2 in, 2 out]
                n579 = local write "Current Status"("Getting camera status..." ("Current Status")) -> ()
              }
            }
            n580 = property on="Lamp Cluster" class="Clust (strict)"() -> ("Controls[]"=w1692:refnum<vi>[])  [unwired: 2 in, 2 out]
            n581 = for {
              tunnel: w1692 -> [w1705] mode=indexing
              n582 = property class="Ctl"(reference=w1705) -> ("Label.Text"=w1706:string)  [unwired: 1 in, 2 out]
              n583 = case shown="\"Quartz\"" w1706 {
                selector: w1706 -> [w1707 w1712 w1717 w1722 w1727 w1734 w1740 _]
                tunnel: w1705 -> [w1709 w1714 w1719 w1724 w1729 w1736 w1742 _]
                frame "Hg(Ar)" {
                  n584 = global read "TCSLINK_global.vi" "Hg(Ar)"() -> (w1708:bool)
                  n585 = property class="Ctl"(reference=w1709, "Value"=w1708) -> ()  [unwired: 1 in, 2 out]
                  n586 = case shown="True" w1708 {
                    tunnel: w1707 -> [_ _]
                    frame False {
                      n587 = property on="Hg(Ar) Ind" class="Ring (strict)"("Value"=0) -> ()  [unwired: 2 in, 2 out]
                    }
                    frame True {
                      n588 = property on="Hg(Ar) Ind" class="Ring (strict)"("Value"=2) -> ()  [unwired: 2 in, 2 out]
                    }
                  }
                }
                frame "Cu" {
                  n589 = global read "TCSLINK_global.vi" "Cu"() -> (w1713:bool)
                  n590 = property class="Ctl"(reference=w1714, "Value"=w1713) -> ()  [unwired: 1 in, 2 out]
                  n591 = case shown="True" w1713 {
                    tunnel: w1712 -> [_ _]
                    frame False {
                      n592 = property on="Cu Ind" class="Ring (strict)"("Value"=0) -> ()  [unwired: 2 in, 2 out]
                    }
                    frame True {
                      n593 = property on="Cu Ind" class="Ring (strict)"("Value"=2) -> ()  [unwired: 2 in, 2 out]
                    }
                  }
                }
                frame "Ne" {
                  n594 = global read "TCSLINK_global.vi" "Ne"() -> (w1718:bool)
                  n595 = property class="Ctl"(reference=w1719, "Value"=w1718) -> ()  [unwired: 1 in, 2 out]
                  n596 = case shown="True" w1718 {
                    tunnel: w1717 -> [_ _]
                    frame False {
                      n597 = property on="Ne Ind" class="Ring (strict)"("Value"=0) -> ()  [unwired: 2 in, 2 out]
                    }
                    frame True {
                      n598 = property on="Ne Ind" class="Ring (strict)"("Value"=2) -> ()  [unwired: 2 in, 2 out]
                    }
                  }
                }
                frame "Fe" {
                  n599 = global read "TCSLINK_global.vi" "Fe"() -> (w1723:bool)
                  n600 = property class="Ctl"(reference=w1724, "Value"=w1723) -> ()  [unwired: 1 in, 2 out]
                  n601 = case shown="True" w1723 {
                    tunnel: w1722 -> [_ _]
                    frame False {
                      n602 = property on="Fe Ind" class="Ring (strict)"("Value"=0) -> ()  [unwired: 2 in, 2 out]
                    }
                    frame True {
                      n603 = property on="Fe Ind" class="Ring (strict)"("Value"=2) -> ()  [unwired: 2 in, 2 out]
                    }
                  }
                }
                frame "Ar" {
                  n604 = global read "TCSLINK_global.vi" "Ar"() -> (w1728:bool)
                  n605 = property class="Ctl"(reference=w1729, "Value"=w1728) -> ()  [unwired: 1 in, 2 out]
                  n606 = case shown="True" w1728 {
                    tunnel: w1727 -> [_ _]
                    frame False {
                      n607 = property on="Ar Ind" class="Ring (strict)"("Value"=0) -> ()  [unwired: 2 in, 2 out]
                    }
                    frame True {
                      n608 = property on="Ar Ind" class="Ring (strict)"("Value"=2) -> ()  [unwired: 2 in, 2 out]
                    }
                  }
                }
                frame "Quartz" {
                  n609 = local read "Quartz Intensity"() -> (w1733:i8)
                  n610 = global read "TCSLINK_global.vi" "Quartz"() -> (w1735:bool)
                  n611 = property class="Ctl"(reference=w1736, "Value"=w1735) -> ()  [unwired: 1 in, 2 out]
                  n612 = Number To Decimal String(number=w1733) -> (decimal integer string=w1732:string)  [unwired: 1 in]
                  n613 = case shown="False" w1735 {
                    tunnel: w1734 -> [_ _]
                    tunnel: w1732 -> [_ w1738]
                    frame False {
                      w1737 = 0
                      n614 = property on="Quartz Ind" class="Ring (strict)"("Value"=w1737) -> ()  [unwired: 2 in, 2 out]
                      n615 = local write "Quartz Intensity"(w1737) -> ()
                    }
                    frame True {
                      n616 = local write "Current Lamp Percent"(w1738) -> ()
                      n617 = property on="Quartz Ind" class="Ring (strict)"("Value"=2) -> ()  [unwired: 2 in, 2 out]
                    }
                  }
                }
                frame "Bulb" {
                  n618 = global read "TCSLINK_global.vi" "Bulb"() -> (w1741:bool)
                  n619 = property class="Ctl"(reference=w1742, "Value"=w1741) -> ()  [unwired: 1 in, 2 out]
                  n620 = case shown="True" w1741 {
                    tunnel: w1740 -> [_ _]
                    frame False {
                      n621 = property on="Bulb Ind" class="Ring (strict)"("Value"=0) -> ()  [unwired: 2 in, 2 out]
                    }
                    frame True {
                      n622 = property on="Bulb Ind" class="Ring (strict)"("Value"=2) -> ()  [unwired: 2 in, 2 out]
                    }
                  }
                }
                frame "", Default {
                }
              }
            }
            n623 = global read "TCSLINK_global.vi" "Dome"() -> (w1691:bool)
            n624 = global read "TCSLINK_global.vi" "Quartz Percent"() -> (→"Quartz Actual":i8)
            n625 = case shown="False" w1691 {
              selector: w1691 -> [w1698 w1701]
              tunnel: [0 w1702] -> _
              frame False {
                n626 = global read "TCSLINK_global.vi" "Dome Percent"() -> (w1699:i8)
                n627 = local write "Dome"(w1698) -> ()
                n628 = local write "Dome Ind"(0) -> ()
                n629 = local write "Dome Percent"(w1699) -> ()
              }
              frame True {
                n630 = global read "TCSLINK_global.vi" "Dome Percent"() -> (w1702:i8)
                "Dome Percent" <- w1702
                n631 = Number To Decimal String(number=w1702) -> (decimal integer string=w1703:string)  [unwired: 1 in]
                n632 = local write "Dome"(w1701) -> ()
                n633 = local write "Current Lamp Percent"(w1703) -> ()
                n634 = local write "Dome Ind"(2) -> ()
              }
            }
            n635 = call "Current Lamps.vi"() -> ("Current Lamps"=w1689:string)  [unwired: 11 in]
            n636 = local write "Current Lamp"(w1689) -> ()
          }
          frame True {
            n637 = global read "Apogee_Global.vi" "Camera State"() -> (w1758:T10)
            n638 = case shown="\"Ready\", Default" w1758 {
              tunnel: w1757 -> [_ w1764]
              tunnel: w1756 -> [w1760 w1767]
              tunnel: w1755 -> [w1761 w1766]
              tunnel: [w1762 w1765] -> w1754
              tunnel: w1753 -> [_ _]
              frame "Exposing" {
                n639 = Enqueue Element(queue=w1760, element=T7 {"Command"="START_SCRIPT", "Parameter"=""}, error in (no error)=w1761) -> (error out=w1762:errorcluster)  [unwired: 1 in, 2 out]
              }
              frame "Ready", Default {
                n640 = Unbundle By Name(w1764) -> ("Current Exposure"=w1769:i32, "#Exposures"=w1768:i32)
                n641 = Greater?(x=w1769, y=w1768) -> (0:w1763:bool)
                n642 = case shown="False" w1763 {
                  tunnel: w1767 -> [w1779 w1824]
                  tunnel: w1766 -> [w1778 w1822]
                  tunnel: [w1777 w1825] -> w1765
                  tunnel: w1764 -> [w1770 w1827]
                  frame False {
                    n643 = local read "Take Thumbnail"() -> (w1773:bool)
                    n644 = Not(x=w1773) -> (.not. x?=w1772:bool)
                    n645 = local read "Mode"() -> (w1776:u16)
                    n646 = Greater?(x=w1776, y=u16 0) -> (0:w1774:bool)
                    n647 = And(x=w1774, y=w1772) -> (x .and. y?=w1771:bool)
                    n648 = case shown="True" w1771 {
                      tunnel: w1779 -> [w1781 w1816]
                      tunnel: w1778 -> [w1782 w1814]
                      tunnel: [w1783 w1818] -> w1777
                      tunnel: w1770 -> [_ _]
                      frame True {
                        n649 = local read "Focus Changed?"() -> (w1780:bool)
                        n650 = case shown="False" w1780 {
                          tunnel: [w1784 w1795] -> w1783
                          tunnel: w1782 -> [w1786 w1790]
                          tunnel: w1781 -> [w1785 w1789]
                          frame False {
                            n651 = Enqueue Element(queue=w1785, element=T7 {"Command"="FOCUS", "Parameter"=""}, error in (no error)=w1786) -> (error out=w1784:errorcluster)  [unwired: 1 in, 2 out]
                          }
                          frame True {
                            n652 = flat-sequence {
                              tunnel: w1790 -> [w1802]
                              tunnel: [w1797] -> _
                              tunnel: [w1797] -> w1788
                              frame #0 {
                                n653 = global write "GPS_Driver_Global.vi" "RODone"(FALSE) -> ()
                              }
                              frame #1 {
                                n654 = Current VI's Path() -> (path=w1801:path)
                                n655 = local read "Open Shutter During Image?"() -> (w1803:bool)
                                n656 = Strip Path(path=w1801) -> (stripped path=w1800:path)  [unwired: 1 out]
                                n657 = Build Path(base path=w1800, name or relative path="GPS_Drivers\\ReadExEventFINAL.vi" ("vi path")) -> (appended path=w1798:path)
                                n658 = case shown="True" w1803 {
                                tunnel: [w1804 w1809] -> w1797
                                tunnel: w1802 -> [w1804 w1806]
                                tunnel: w1798 -> [_ w1811]
                                frame False {
                                }
                                frame True {
                                n659 = Open VI Reference(vi path=w1811, error in (no error)=w1806) -> (vi reference=w1810:refnum<vi>, error out=w1805:errorcluster)  [unwired: 4 in]
                                n660 = invoke class="VI" method="Run VI"(reference=w1810, error in=w1805, "Wait until done"=FALSE, "Auto Dispose Ref"=TRUE) -> (error out=w1809:errorcluster)  [unwired: 1 in, 4 out]
                                }
                                }
                              }
                            }
                            n661 = Enqueue Element(queue=w1789, element=T7 {"Command"="DISABLE_CONTROLS", "Parameter"=""}, error in (no error)=w1788) -> (queue out=w1793:refnum<queue>, error out=w1792:errorcluster)  [unwired: 1 in, 1 out]
                            n662 = Enqueue Element(queue=w1793, element=T7 {"Command"="WRITE_FITS_HEADER", "Parameter"=""}, error in (no error)=w1792) -> (error out=w1795:errorcluster)  [unwired: 1 in, 2 out]
                          }
                        }
                      }
                      frame False {
                        n663 = Enqueue Element(queue=w1816, element=T7 {"Command"="DISABLE_CONTROLS", "Parameter"=""}, error in (no error)=w1814) -> (queue out=w1815:refnum<queue>, error out=w1813:errorcluster)  [unwired: 1 in, 1 out]
                        n664 = Enqueue Element(queue=w1815, element=T7 {"Command"="START_SCRIPT", "Parameter"=""}, error in (no error)=w1813) -> (error out=w1818:errorcluster)  [unwired: 1 in, 2 out]
                      }
                    }
                  }
                  frame True {
                    w1819 = FALSE ("Exposure Active?")
                    n665 = Bundle By Name(cluster=w1827, "Exposure Active?"=w1819) -> (w1826:T6)
                    n666 = Enqueue Element(queue=w1824, element=T7 {"Command"="ENABLE_CONTROLS", "Parameter"=""}, error in (no error)=w1822) -> (queue out=w1823:refnum<queue>, error out=w1821:errorcluster)  [unwired: 1 in, 1 out]
                    n667 = global write "SIcamera_Globals.vi" "Exposure Active?"(w1819) -> ()
                    n668 = local write "Script"(w1826) -> ()
                    n669 = Enqueue Element(queue=w1823, element=T7 {"Command"="END_SCRIPT", "Parameter"=""}, error in (no error)=w1821) -> (error out=w1825:errorcluster)  [unwired: 1 in, 2 out]
                  }
                }
              }
            }
          }
        }
        n670 = global read "GSP_GUI_global.vi" "User Type"() -> (w1671:i8)
        n671 = case shown="0, Default" w1671 {
          tunnel: [TRUE ("Visible") TRUE ("Visible")] -> w1670
          frame 0, Default {
          }
          frame 2, 3 {
          }
        }
        n672 = property on="Port Readout" class="Ring (strict)"("Visible"=w1670) -> ()  [unwired: 2 in, 2 out]
        n673 = property on="Save As" class="Ring (strict)"("Visible"=w1670) -> ()  [unwired: 2 in, 2 out]
      }
      frame "TAKE_IMAGE" {
        # "Code from SI camera client software..."
        n674 = Unbundle By Name(w1834) -> ("Current Exposure"=w1836:i32, "#Exposures"=w1830:i32)
        n675 = Tick Count (ms)() -> (millisecond timer value=w1835:u32)
        n676 = Decrement(x=w1836) -> (x-1=w1829:i32)
        n677 = Number To Decimal String(number=w1829) -> (decimal integer string=w1841:string)  [unwired: 1 in]
        n678 = Number To Decimal String(number=w1830) -> (decimal integer string=w1839:string)  [unwired: 1 in]
        n679 = while {
          shift-right: [w1882] -> _
          shift-left: TRUE -> [w1883]
          shift-right: [w1880] -> _
          shift-left: _ -> [w1881]
          shift-right: [w1878] -> _
          shift-left: 0 ("timeout ms (5000)") -> [w1879]
          tunnel: w1835 -> [w1876]
          tunnel: w1833 -> [_]
          tunnel: w1834 -> [w1868]
          tunnel: w1833 -> [w1867]
          tunnel: w1832 -> [w1865]
          tunnel: w1831 -> [w1864]
          tunnel: w1830 -> [w1857]
          tunnel: w1829 -> [w1856]
          stop <- w1847 continue-if-true
          # "This Wait was added to work with Linux"
          n680 = local read "Start Exposure"() -> (w1869:bool)
          n681 = case shown="False" w1869 {
            selector: w1869 -> [_ w1921]
            tunnel: [TRUE w1921] -> w1866
            tunnel: w1868 -> [w1912 _]
            tunnel: w1867 -> [w1905 w1919]
            tunnel: w1865 -> [w1908 _]
            tunnel: w1864 -> [w1906 _]
            tunnel: [w1902 w1918] -> w1853
            tunnel: [_ w1917] -> w1852
            tunnel: [_ w1916] -> w1851
            tunnel: [_ w1915] -> w1850
            tunnel: [w1901 w1914] -> w1849
            tunnel: [w1900 w1913] -> w1848
            frame False {
              n682 = Bundle By Name(cluster=w1912, "#Exposures"=0) -> (w1910:T6)
              n683 = Enqueue Element(queue=w1908, element=T7 {"Command"="ABORT_RECOVERY", "Parameter"=""}) -> ()  [unwired: 2 in, 3 out]
              n684 = call "Send Single TCP-IP Cmd Abort.vi"("TCP/IP ID"=w1905, "Camera Color"=w1906, "Function #"=u16 1018, "Camera ID"=u8 1) -> ("Data Type"=w1901:i32, "Packet ID"=w1900:i32, "Error Out"=w1902:errorcluster)  [unwired: 11 in, 2 out]
              n685 = local write "Script"(w1910) -> ()
            }
            frame True {
              n686 = call "Parse TCP-IP Response 4_RED.vi"("TCP/IP ID"=w1919, "timeout ms (5000)"=100) -> ("Packet ID"=w1913:u8, "Data Type"=w1914:u16, "Command Done"=w1915:cluster{"Function #":u16}, "Acq. Status"=w1916:T19, "Image Packet"=w1917:T20, "error out"=w1918:errorcluster)  [unwired: 3 in, 5 out]
            }
          }
          n687 = local read "Readout Time"() -> (w1871:dbl)
          n688 = case shown="No Error" w1853 {
            selector: w1853 -> [_ w2051]
            tunnel: w1848 -> [w1933 _]
            tunnel: w1850 -> [w1932 _]
            tunnel: w1851 -> [w1923 _]
            tunnel: [w1931 w2052] -> w1884
            tunnel: w1849 -> [w1930 _]
            tunnel: w1881 -> [w1929 w2054]
            tunnel: [w1928 w2054] -> w1880
            tunnel: [w1927 w2049] -> w1882
            tunnel: w1883 -> [w1926 w2049]
            tunnel: w1879 -> [w1925 w2050]
            tunnel: [w1924 w2050] -> w1878
            tunnel: w1852 -> [w1922 _]
            frame No Error {
              n689 = case shown="131" w1933 {
                tunnel: w1932 -> [_ _ _]
                tunnel: w1923 -> [_ w1944 _]
                tunnel: [TRUE w1942 w1979] -> w1931
                tunnel: w1930 -> [_ w1943 _]
                tunnel: w1929 -> [w1936 w1941 w1984]
                tunnel: [w1936 w1941 w1982] -> w1928
                tunnel: [w1935 w1940 FALSE] -> w1927
                tunnel: w1926 -> [w1935 w1940 w1983]
                tunnel: w1925 -> [w1934 w1939 w1981]
                tunnel: [w1934 w1939 w1980] -> w1924
                tunnel: w1922 -> [_ _ w1978]
                frame 0, Default {
                  n690 = One Button Dialog(message="An unknown Packet Identifier was received.") -> ()  [unwired: 1 in, 1 out]
                }
                frame 131 {
                  n691 = case shown="2007" w1943 {
                    tunnel: w1944 -> [_ _ w1973]
                    tunnel: [TRUE FALSE TRUE] -> w1942
                    frame 0, Default {
                    }
                    frame 2007 {
                      w1946 = TRUE
                      # "Command Done"
                      n692 = local read "Image #"() -> (w1947:i32)
                      n693 = local read "File Name Base"() -> (w1951:string)
                      n694 = local read "Start Exposure"() -> (w1948:bool)
                      n695 = case shown="False" w1948 {
                        tunnel: [w1957 w1960] -> w1949
                        tunnel: w1947 -> [w1958 w1959]
                        frame False {
                          n696 = Increment(x=w1958) -> (x+1=w1957:i32)
                          n697 = local write "Image #"(w1957) -> ()
                        }
                        frame True {
                          n698 = Increment(x=w1959) -> (x+1=w1960:i32)
                          n699 = local write "Image #"(w1960) -> ()
                        }
                      }
                      n700 = Format Into String(format string="%04d", w1949) -> (resulting string=w1953:string)  [unwired: 2 in, 1 out]
                      n701 = Concatenate Strings(w1953, "_" ("string"), w1951) -> (w1950:string)
                      n702 = local write "Image File Name"(w1950) -> ()
                      n703 = global write "Apogee_Global.vi" "Camera State"(CameraStates."Ready" ("Camera State")) -> ()
                      n704 = global write "GPS_Driver_Global.vi" "RODone"(w1946) -> ()
                      n705 = local write "RO Done"(w1946) -> ()
                    }
                    frame 2004 {
                      n706 = Unbundle By Name(w1973) -> ("% Exp."=w1963:u16, "%Readout"=w1966:u16)
                      n707 = local read "Readout"() -> (w1968:u16)
                      n708 = Equal To 0?(x=w1966) -> (x = 0?=w1965:bool)
                      n709 = Greater?(x=w1968, y=w1966) -> (0:w1967:bool)
                      n710 = Less?(x=w1966, y=u16 100) -> (x < y?=w1971:bool)
                      n711 = Select(t=w1963, s=w1965, f=u16 100) -> (s? t:f=→"Exposure":u16)
                      n712 = Not(x=w1971) -> (.not. x?=w1961:bool)
                      n713 = local write "RO Done"(w1961) -> ()
                      n714 = global write "GPS_Driver_Global.vi" "RODone"(w1961) -> ()
                      n715 = case shown="False" w1967 {
                        tunnel: [w1974 w1975] -> w1969
                        tunnel: w1966 -> [w1974 w1975]
                        frame False {
                        }
                        frame True {
                          n716 = local read "Acquiring"() -> (w1976:u32)
                          n717 = Increment(x=w1976) -> (x+1=w1977:u32)
                          n718 = local write "Acquiring"(w1977) -> ()
                        }
                      }
                      "Readout" <- w1969
                    }
                  }
                }
                frame 132 {
                  n719 = Unbundle By Name(w1978) -> ("Image Data $"=w1993:string, "Image Type"=w1992:u16, "Serial Length"=w1991:u16, "Parallel Length"=w1990:u16, "Offset"=w1986:u32, "# of Packets"=w1989:u16)  [unwired: 1 out]
                  n720 = To Long Integer(number=w1990) -> (32bit integer=w1988:i32)
                  n721 = To Long Integer(number=w1991) -> (32bit integer=w1987:i32)
                  n722 = case shown="0, Default" w1992 {
                    tunnel: [w2028 w2031 w2036 w2039 w2043 w2046] -> w1985
                    tunnel: w1993 -> [w2026 w2030 w2034 w2038 w2042 w2045]
                    frame 0, Default {
                      # "U16"
                      n723 = Type Cast(type=u16[] [] ("Array Constant"), x=w2026) -> (*(type *) &x=w2029:u16[])
                      n724 = To Single Precision Float(number=w2029) -> (single precision float=w2028:sgl[])
                    }
                    frame 1 {
                      # "I16"
                      n725 = Type Cast(type=i16[] [] ("Array Constant"), x=w2030) -> (*(type *) &x=w2033:i16[])
                      n726 = To Single Precision Float(number=w2033) -> (single precision float=w2031:sgl[])
                    }
                    frame 2 {
                      # "U32"
                      n727 = Type Cast(type=u32[] [] ("Array Constant"), x=w2034) -> (*(type *) &x=w2037:u32[])
                      n728 = To Single Precision Float(number=w2037) -> (single precision float=w2036:sgl[])
                    }
                    frame 3 {
                      # "I32"
                      n729 = Type Cast(type=i32[] [] ("Array Constant"), x=w2038) -> (*(type *) &x=w2041:i32[])
                      n730 = To Single Precision Float(number=w2041) -> (single precision float=w2039:sgl[])
                    }
                    frame 4 {
                      # "SGL"
                      n731 = Type Cast(type=sgl[] [] ("Array Constant"), x=w2042) -> (*(type *) &x=w2043:sgl[])
                    }
                    frame 5 {
                      # "DBL"
                      n732 = Type Cast(type=dbl[] [] ("Array Constant"), x=w2045) -> (*(type *) &x=w2048:dbl[])
                      n733 = To Single Precision Float(number=w2048) -> (single precision float=w2046:sgl[])
                    }
                  }
                  n734 = case shown="True" w1983 {
                    tunnel: w1984 -> [w2002 _]
                    tunnel: w1987 -> [_ w2014]
                    tunnel: w1988 -> [_ w2015]
                    tunnel: [w2003 w2024] -> w1982
                    tunnel: w1985 -> [w2010 w2023]
                    tunnel: w1981 -> [w1995 w2021]
                    tunnel: [w2000 w2013] -> w1980
                    tunnel: [w2009 w2020] -> w1979
                    tunnel: w1986 -> [w2001 w2018]
                    tunnel: w1989 -> [w1998 w2017]
                    frame False {
                      w1997 = 100.0 ("y")
                      n735 = Increment(x=w1995) -> (x+1=w2000:i32)
                      n736 = Less?(x=w2000, y=w1998) -> (x < y?=w2009:bool)
                      n737 = Divide(x=w2000, y=w1998) -> (x/y=w2005:dbl)
                      n738 = Divide(x=w1998, y=w1997) -> (x/y=w1999:dbl)
                      n739 = Multiply(x=w2005, y=w1997) -> (x*y=w2004:dbl)
                      n740 = To Unsigned Word Integer(number=w1999) -> (unsigned 16bit integer=w1996:u16)
                      n741 = Quotient & Remainder(x=w2000, y=w1996) -> (x-y*floor(x/y)=w2008:i32)  [unwired: 1 out]
                      n742 = To Unsigned Word Integer(number=w2004) -> (unsigned 16bit integer=w2006:u16)
                      n743 = Equal To 0?(x=w2008) -> (x = 0?=w2007:bool)
                      n744 = case shown="True" w2007 {
                        tunnel: w2006 -> [_ w2011]
                        frame False {
                        }
                        frame True {
                          n745 = local write "Readout"(w2011) -> ()
                        }
                      }
                      n746 = Replace Array Subset(array=w2002, new element=w2010, index=w2001) -> (w2003:sgl[])
                    }
                    frame True {
                      w2012 = TRUE
                      n747 = Increment(x=w2021) -> (x+1=w2013:i32)
                      n748 = global write "GPS_Driver_Global.vi" "RODone"(w2012) -> ()
                      n749 = local write "RO Done"(w2012) -> ()
                      n750 = Less?(x=w2013, y=w2017) -> (x < y?=w2020:bool)
                      n751 = Multiply(x=w2014, y=w2015) -> (x*y=w2019:i32)
                      n752 = Initialize Array(sgl 0.0 ("Element Data"), w2019) -> (w2022:sgl[])
                      n753 = property on="Readout" class="Slide (strict)"("Caption.Text"="%Transfered") -> ()  [unwired: 2 in, 2 out]
                      n754 = Replace Array Subset(array=w2022, new element=w2023, index=w2018) -> (w2024:sgl[])
                      "P Len" <- w2015
                      "S Len" <- w2014
                    }
                  }
                }
              }
            }
            frame Error {
              n755 = Unbundle By Name(w2051) -> ("code"=w2053:i32)
              n756 = case shown="0, Default" w2053 {
                tunnel: w2051 -> [w2058 _]
                tunnel: [w2056 TRUE] -> w2052
                frame 0, Default {
                  w2056 = FALSE
                  n757 = call <vilib>:"Simple Error Handler.vi"("error source (\" \")"="There was an error in a TCP/IP read during an Image Acquisition. ", "error in (no error)"=w2058) -> ("error out"=w2055:errorcluster)  [unwired: 3 in, 4 out]
                  n758 = local write "Error out"(w2055) -> ()
                  n759 = local write "Start Exposure"(w2056) -> ()
                }
                frame 56 {
                  # "Timeout -  Keep going"
                }
              }
            }
          }
          n760 = Multiply(x=w1871, y=1000.0) -> (x*y=w1870:dbl)
          n761 = local read "Readout"() -> (w1874:u16)
          n762 = And(x=w1884, y=w1866) -> (x .and. y?=w1847:bool)
          n763 = local read "Exp. Time (s)"() -> (w1860:dbl)
          n764 = local read "Mode"() -> (w1875:u16)
          n765 = property on="Readout" class="Slide (strict)"() -> ("Caption.Text"=w1873:string)  [unwired: 2 in, 2 out]
          n766 = call "GetExposureStatus.vi"("Readout Time"=w1870, "% Complete Caption"=w1873, "Previous % Complete Value"=w1874, "Exposure Time"=w1860, "Mode #"=w1875, "Initial Time"=w1876) -> ("Exp time left"=w1863:dbl, "Readout left"=w1855:dbl, "% Exposed"=w1861:dbl, "% Complete"=w1858:dbl)
          "Exp time left" <- w1863
          "Readout left" <- w1855
          n767 = Wait (ms)(milliseconds to wait=u32 0) -> ()  [unwired: 1 out]
          n768 = local write "Exposure"(w1861) -> ()
          n769 = local write "Readout"(w1858) -> ()
          n770 = Greater Than 0?(x=w1863) -> (x > 0?=w1862:bool)
          n771 = case shown="True" w1862 {
            selector: w1862 -> [w1887 w1899]
            tunnel: w1861 -> [_ w1897]
            tunnel: w1860 -> [_ w1896]
            tunnel: w1857 -> [_ w1891]
            tunnel: w1856 -> [_ w1892]
            frame False {
              n772 = property on="Exp time left" class="DigNum (strict)"("Visible"=w1887) -> ()  [unwired: 2 in, 2 out]
              n773 = property on="Exposure" class="Slide (strict)"("Blinking"=w1887) -> ()  [unwired: 2 in, 2 out]
            }
            frame True {
              n774 = Greater?(x=w1896, y=300.0) -> (0:w1893:bool)
              n775 = property on="Exp time left" class="DigNum (strict)"("Visible"=w1899) -> ()  [unwired: 2 in, 2 out]
              n776 = Equal?(x=w1892, y=w1891) -> (x = y?=w1889:bool)
              n777 = Greater?(x=w1897, y=98) -> (0:w1894:bool)
              n778 = And(x=w1894, y=w1893) -> (x .and. y?=w1890:bool)
              n779 = And(x=w1890, y=w1889) -> (x .and. y?=w1888:bool)
              n780 = property on="Exposure" class="Slide (strict)"("Blinking"=w1888) -> ()  [unwired: 2 in, 2 out]
            }
          }
          n781 = case shown="False" "?" {
            frame False {
              # "if shutter is closed open it"
            }
            frame True {
              # "tell motor to close"
            }
          }
          n782 = Greater Than 0?(x=w1855) -> (x > 0?=w1859:bool)
          n783 = case shown="True" w1859 {
            selector: w1859 -> [w1885 w1886]
            frame False {
              n784 = property on="Readout left" class="DigNum (strict)"("Visible"=w1885) -> ()  [unwired: 2 in, 2 out]
            }
            frame True {
              n785 = property on="Readout left" class="DigNum (strict)"("Visible"=w1886) -> ()  [unwired: 2 in, 2 out]
            }
          }
        }
        n786 = Concatenate Strings("Acquiring image " ("Current Status"), w1841, " of " ("Current Status"), w1839, " ... " ("Current Status")) -> (w1837:string)
        n787 = local write "Current Status"(w1837) -> ()
        n788 = global write "Apogee_Global.vi" "Camera State"(CameraStates."Ready" ("Camera State")) -> ()
      }
      frame "WRITE_FITS_HEADER" {
        # "Write FITS header file before taking image; change camera state to 'exposing', increase exposure # by 1"
        n789 = Unbundle By Name(w2097) -> ("Reduction Info."=w2064:T21, "Obs parameters"=w2062:T22, "Component Names"=w2080:T17, "Other Info."=w2087:T23)  [unwired: 3 out]
        n790 = Delete(path (use dialog)=path "C:/Users/Public/Documents/SI Image SGL II -/Other Parameters.txt" ("Path to FITS Header File"), error in=w2094) -> (deleted path=w2090:path, error out=w2091:errorcluster)  [unwired: 3 in, 1 out]
        n791 = call "WriteObsInfo.vi"("error in (no error)"=w2091, "Obs parameters"=w2062, "Path to FITS Header File"=w2090) -> ("error out"=w2093:errorcluster, "# of Entries (after)"=w2078:i16, "Path to FITS Header File"=w2092:path)  [unwired: 2 in]
        n792 = call "GetTCSInfo.vi"() -> ("TCSInfo"=w2060:T15)
        n793 = call "WriteTCSInfo.vi"("error in (no error)"=w2093, "# of Entries (before)"=w2078, "TCSInfo"=w2060, "Pathto FITS Header File"=w2092) -> ("error out"=w2079:errorcluster, "# of Entries (after)"=w2077:i16, "Path to FITS Header File"=w2081:path)  [unwired: 1 in]
        n794 = call "GetSystemsInfo.vi"() -> ("Pos Info"=w2061:T16)
        n795 = call "WriteGoodmanInfo.vi"("System Pos Info"=w2061, "error in (no error)"=w2079, "# of Entries (before)"=w2077, "Component Names"=w2080, "Path to FITS Header File"=w2081) -> ("error out"=w2073:errorcluster, "# of Entries (after)"=w2074:i16, "Path to FITS Header File"=w2076:path)  [unwired: 1 in]
        n796 = local read "Exp. Time (s)"() -> (w2088:dbl)
        n797 = Unbundle(w2087) -> ("CCD Read Noise"=w2086:dbl, "CCD Gain"=w2085:dbl, "OBSTYPE"=w2084:string, "OBSERVER"=w2083:string, "Proposal #"=w2082:string, "Equinox"=w2072:dbl)
        n798 = local read "ROIMODE"() -> (w2063:string)
        n799 = Bundle("Exp. Time (s)"=w2088, "CCD Read Noise"=w2086, "CCD Gain"=w2085, "OBSTYPE"=w2084, "OBSERVER"=w2083, "Proposal #"=w2082, "Equinox"=w2072, "ROIMODE"=w2063) -> (w2075:T24)  [unwired: 1 in]
        n800 = call "WriteOtherInfo.vi"("error in (no error)"=w2073, "# of Entries (before)"=w2074, "Other Info"=w2075, "Path to FITS Header File"=w2076) -> ("error out"=w2069:errorcluster, "# of Entries (after)"=w2067:i16, "Path to FITS Header File"=w2071:path)  [unwired: 1 in]
        n801 = call "GetEnvironmentalInfo.vi"() -> ("Environmental Info"=w2065:T25)
        n802 = local write "Current Status"("Writing FITS Header File...." ("Current Status")) -> ()
        n803 = global write "Apogee_Global.vi" "Camera State"(CameraStates."Exposing" ("Camera State")) -> ()
        n804 = call "WriteEnvironmentInfo.vi"("error in (no error)"=w2069, "# of Entries (before)"=w2067, "EnvironmentalInfo"=w2065, "Pathto FITS Header File"=w2071) -> ("error out"=w2068:errorcluster, "# of Entries (after)"=w2066:i16, "Path to FITS Header File"=w2070:path)  [unwired: 1 in]
        n805 = call "WriteReductionInfo.vi"("error in (no error)"=w2068, "# of Entries (before)"=w2066, "Reduction Info."=w2064, "Path to FITS Header File"=w2070) -> ()  [unwired: 1 in, 3 out]
      }
      frame "DISABLE_CONTROLS" {
        w2103 = u8 1 ("Disabled")
        n806 = Obtain Queue(name (unnamed)="Coll_Command_Q", element data type=T7 {"Command"="", "Parameter"=""} ("Command")) -> (queue out=w2099:refnum<queue>)  [unwired: 3 in, 2 out]
        n807 = property on="Port Readout" class="Ring (strict)"("Disabled"=w2103) -> ()  [unwired: 2 in, 2 out]
        n808 = property on="CCD Readout Speed" class="Ring (strict)"("Disabled"=w2103) -> ()  [unwired: 2 in, 2 out]
        n809 = property on="Systems Status & Control" class="TabCtl (strict)"("Disabled"=w2103) -> ()  [unwired: 2 in, 2 out]
        n810 = local read "Take Thumbnail"() -> (w2107:bool)
        n811 = property on="File Name Base" class="Str"("Disabled"=w2103) -> ()  [unwired: 2 in, 2 out]
        n812 = property on="Save" class="Bool (strict)"("Disabled"=w2103) -> ()  [unwired: 2 in, 2 out]
        n813 = property on="Image #" class="DigNum (strict)"("Disabled"=w2103) -> ()  [unwired: 2 in, 2 out]
        n814 = Select(t=1.0, s=w2107, f=0.0) -> (s? t:f=w2104:dbl)
        n815 = property on="Exposure Tab" class="TabCtl (strict)"("Disabled"=w2103) -> ()  [unwired: 2 in, 2 out]
        n816 = property on="Thumbnail Setting" class="Enum (strict)"("Disabled"=w2103) -> ()  [unwired: 2 in, 2 out]
        n817 = property on="CCD ROI Mode" class="Ring (strict)"("Disabled"=w2103) -> ()  [unwired: 2 in, 2 out]
        n818 = property on="Take Thumbnail" class="Bool (strict)"("Disabled"=w2103) -> ()  [unwired: 2 in, 2 out]
        n819 = property on="Start Exposure" class="Bool (strict)"("Disabled"=w2104) -> ()  [unwired: 2 in, 2 out]
        n820 = property on="Get Camera Status" class="Bool (strict)"("Disabled"=w2103) -> ()  [unwired: 2 in, 2 out]
        n821 = property on="Save As" class="Ring (strict)"("Disabled"=w2103) -> ()  [unwired: 2 in, 2 out]
        n822 = property on="Acq Mode" class="Enum (strict)"("Disabled"=w2103) -> ()  [unwired: 2 in, 2 out]
        n823 = property on="Exp. Time (s)" class="DigNum (strict)"("Disabled"=w2103) -> ()  [unwired: 2 in, 2 out]
        n824 = Enqueue Element(queue=w2099, element=T7 {"Command"="DISABLE", "Parameter"=""}) -> (queue out=w2098:refnum<queue>)  [unwired: 2 in, 2 out]
        n825 = Release Queue(queue=w2098) -> ()  [unwired: 2 in, 3 out]
      }
      frame "FOCUS" {
        # "first pause to give time for system to register move\nthen wait for thread state to be done\nthen pause again to allow time for the flexure comp"
        n826 = Unbundle By Name(w2116) -> ("Current Exposure"=w2115:i32)
        n827 = Decrement(x=w2115) -> (x-1=w2114:i32)
        n828 = Multiply(x="Step Size", y=w2114) -> (x*y=w2120:dbl)
        n829 = Add(x="Focus Start", y=w2120) -> (x+y=w2118:dbl)
        n830 = call "GSP_Manager_CF_driver.vi"("error in (no error)"=w2117, "Target (Move Only)"=w2118, "Action"=CF_drivercontrol."Move") -> ("error out"=w2112:errorcluster)  [unwired: 4 in, 1 out]
        n831 = while {
          tunnel: [w2123] -> w2111
          tunnel: w2112 -> [w2124]
          i -> [w2125]
          stop <- w2122 stop-if-true
          n832 = case shown="0" w2125 {
            tunnel: w2124 -> [w2128 w2129]
            tunnel: [w2127 w2129] -> w2123
            tunnel: [FALSE w2130] -> w2122
            frame 0 {
              n833 = call "Time Delay"("error in (no error)"=w2128) -> ("error out"=w2127:errorcluster)  [unwired: 10 in]
            }
            frame 1, Default {
              n834 = global read "GSP_CF_Global.vi" "CF Thread State"() -> (w2132:T26)
              n835 = Equal?(x=w2132, y=0) -> (x = y?=w2130:bool)
            }
          }
        }
        n836 = local write "Focus Changed?"(TRUE) -> ()
        n837 = call "Time Delay2"("error in (no error)"=w2111) -> ("error out"=w2110:errorcluster)  [unwired: 10 in]
      }
      frame "START_SCRIPT" {
        # "Send acquisition command to camera"
        n838 = Unbundle By Name(w2145) -> ("Current Exposure"=w2148:i32)
        n839 = local read "Image #"() -> (w2144:i32)
        n840 = Increment(x=w2148) -> (x+1=w2147:i32)
        n841 = Format Into String(format string="%04d", w2144) -> (resulting string=w2142:string)  [unwired: 2 in, 1 out]
        n842 = Bundle By Name(cluster=w2145, "Current Exposure"=w2147) -> (w2146:T6)
        n843 = Concatenate Strings(w2142, "_" ("string"), "File Name Base", ".fits" ("string")) -> (w2139:string)
        "Current File Name" <- w2139
        n844 = case shown="1..4, Default" "Mode" {
          selector: "Mode" -> [w2241 w2249]
          tunnel: [w2242 w2251] -> w2158
          tunnel: "Acq Mode" -> [_ w2248]
          tunnel: w2139 -> [_ w2247]
          tunnel: w2136 -> [w2239 w2246]
          tunnel: w2137 -> [_ w2245]
          frame 0 {
            n845 = call "Create Command Packet 3_red.vi"("Function #"=u16 1019, "Camera ID (1)"=u8 1 ("Camera ID"), "Buffer/Avg #/Frames"=u16 1 ("Buffer #"), "Camera Color"=w2239, "Mode"=w2241) -> ("Cmd Packet"=w2242:string)  [unwired: 10 in]
          }
          frame 1..4, Default {
            w2253 = u16 1037  # Function #
            w2250 = u32 1  # Buffer
            w2252 = u8 1  # Camera ID
            n846 = case shown="\"Single Image\", Default" w2248 {
              frame "Single Image", Default {
              }
              frame "Average Images" {
                n847 = local write "Acquiring"(u32 1 ("Acquiring")) -> ()
              }
            }
            n848 = call "Create Command Packet 3_red.vi"("Function #"=w2253, "Camera ID (1)"=w2252, "Buffer/Avg #/Frames"=w2250, "Camera Color"=w2246, "Mode"=w2249, "File Name"=w2247, "Save As"=w2245) -> ("Cmd Packet"=w2251:string)  [unwired: 8 in]
          }
        }
        n849 = local write "Script"(w2146) -> ()
        n850 = call "Flush TCP-IP Input Buffer.vi"("TCP/IP ID"=w2149) -> ("TCP/IP ID Out"=w2159:refnum<k5>)  [unwired: 4 in]
        n851 = call "Send TCP-IP Cmd and Get Ackn 3.vi"("TCP/IP ID In"=w2159, "Cmd Packet"=w2158) -> ("Accepted Flag"=w2151:bool, "error out"=w2134:errorcluster)  [unwired: 7 in, 5 out]
        n852 = Unbundle By Name(w2134) -> ("code"=w2133:i32)
        n853 = Unbundle By Name(w2134) -> ("status"=w2154:bool)
        n854 = Not(x=w2154) -> (.not. x?=w2153:bool)
        n855 = Or(x=w2151, y=w2153) -> (x .or. y?=w2157:bool)
        n856 = case shown="True" w2157 {
          tunnel: w2156 -> [w2167 w2189]
          tunnel: w2152 -> [w2166 w2190]
          tunnel: [w2165 w2181] -> w2135
          tunnel: w2136 -> [_ w2180]
          tunnel: w2133 -> [w2164 _]
          frame False {
            n857 = Equal?(x=w2164, y=62) -> (x = y?=w2162:bool)
            n858 = case shown="True" w2162 {
              tunnel: w2167 -> [w2172 w2179]
              tunnel: w2166 -> [w2171 w2177]
              tunnel: [w2170 w2176] -> w2165
              frame True {
                w2168 = FALSE ("Connection Status")
                n859 = Enqueue Element(queue=w2172, element=T7 {"Command"="INIT_TCP", "Parameter"=""}, error in (no error)=w2171) -> (error out=w2170:errorcluster)  [unwired: 1 in, 2 out]
                n860 = local write "Connection Status"(w2168) -> ()
                n861 = local write "Start Exposure"(w2168) -> ()
                n862 = local write "Current Status"("Resetting TCP/IP connection..." ("Current Status")) -> ()
                n863 = One Button Dialog(message="The Command sent was not accepted by the Camera Server. TCP/IP communication shall be restored shortly.") -> ()  [unwired: 1 in, 1 out]
              }
              frame False {
                n864 = Enqueue Element(queue=w2179, element=T7 {"Command"="START_SCRIPT", "Parameter"=""}, error in (no error)=w2177) -> (error out=w2176:errorcluster)  [unwired: 1 in, 2 out]
                n865 = One Button Dialog(message="The Command sent was not accepted by the Camera Server.") -> ()  [unwired: 1 in, 1 out]
              }
            }
          }
          frame True {
            n866 = local read "Exp. Time (s)"() -> (w2184:dbl)
            n867 = local read "Open Shutter During Image?"() -> (w2183:bool)
            n868 = Enqueue Element(queue=w2189, element=T7 {"Command"="TAKE_IMAGE", "Parameter"=""}, error in (no error)=w2190) -> (queue out=w2186:refnum<queue>, error out=w2187:errorcluster)  [unwired: 1 in, 1 out]
            n869 = Enqueue Element(queue=w2186, element=T7 {"Command"="SEND_IMAGE", "Parameter"=""}, error in (no error)=w2187) -> (error out=w2182:errorcluster)  [unwired: 1 in, 2 out]
            n870 = case shown="\"Red\", Default" w2180 {
              tunnel: w2183 -> [w2194 w2218]
              tunnel: [w2192 w2217] -> w2181
              tunnel: w2182 -> [w2193 w2216]
              tunnel: w2184 -> [w2191 w2215]
              frame "Red", Default {
                n871 = case shown="True" w2194 {
                  tunnel: w2193 -> [w2198 w2206]
                  tunnel: [w2197 w2205] -> w2192
                  tunnel: w2191 -> [_ w2202]
                  frame False {
                    n872 = Number To Decimal String(number=500) -> (decimal integer string=w2200:string)  [unwired: 1 in]
                    n873 = Build Array(w2200) -> (w2201:string[])
                    n874 = call "gsp_silvermax_commandreponse.vi"("error in (no error)"=w2198, "Parameters (none)"=w2201, "Motor #"=u8 40, "Command"=T9."LRP (156)") -> ("error out"=w2197:errorcluster)  [unwired: 3 out]
                  }
                  frame True {
                    n875 = Multiply(x=w2202, y=8333.33) -> (x*y=w2204:dbl)
                    n876 = To Long Integer(number=w2204) -> (32bit integer=w2212:i32)
                    n877 = call "gsp_silvermax_writeregister.vi"("Register Value"=w2212, "Motor #"=u8 40, "Register# (0)"=u8 5) -> ("Motor # dup"=w2210:u8)  [unwired: 3 in, 1 out]
                    n878 = Number To Decimal String(number=600) -> (decimal integer string=w2209:string)  [unwired: 1 in]
                    n879 = Build Array(w2209) -> (w2207:string[])
                    n880 = call "gsp_silvermax_commandreponse.vi"("error in (no error)"=w2206, "Parameters (none)"=w2207, "Motor #"=w2210, "Command"=T9."LRP (156)") -> ("error out"=w2205:errorcluster)  [unwired: 3 out]
                  }
                }
              }
              frame "Blue" {
                n881 = case shown="True" w2218 {
                  tunnel: w2216 -> [w2219 w2230]
                  tunnel: [w2220 w2229] -> w2217
                  tunnel: w2215 -> [_ w2226]
                  frame False {
                    n882 = Number To Decimal String(number=500) -> (decimal integer string=w2224:string)  [unwired: 1 in]
                    n883 = Build Array(w2224) -> (w2225:string[])
                    n884 = call "gsp_silvermax_commandreponse.vi"("error in (no error)"=w2219, "Parameters (none)"=w2225, "Motor #"=u8 40, "Command"=T9."LRP (156)") -> ("error out"=w2220:errorcluster)  [unwired: 3 out]
                  }
                  frame True {
                    n885 = Multiply(x=w2226, y=8333.33) -> (x*y=w2228:dbl)
                    n886 = To Long Integer(number=w2228) -> (32bit integer=w2236:i32)
                    n887 = call "gsp_silvermax_writeregister.vi"("Register Value"=w2236, "Motor #"=u8 40, "Register# (0)"=u8 5) -> ("Motor # dup"=w2234:u8)  [unwired: 3 in, 1 out]
                    n888 = Number To Decimal String(number=450) -> (decimal integer string=w2233:string)  [unwired: 1 in]
                    n889 = Build Array(w2233) -> (w2231:string[])
                    n890 = call "gsp_silvermax_commandreponse.vi"("error in (no error)"=w2230, "Parameters (none)"=w2231, "Motor #"=w2234, "Command"=T9."LRP (156)") -> ("error out"=w2229:errorcluster)  [unwired: 3 out]
                  }
                }
              }
            }
          }
        }
        n891 = local write "Current Status"("Initializing acquisition..." ("Current Status")) -> ()
        n892 = local write "RO Done"(FALSE ("RO Done")) -> ()
      }
      frame "ABORT_RECOVERY" {
        # "should add a color option here to run the red program when red"
        n893 = case shown="\"Red\", Default" w2255 {
          tunnel: w2257 -> [w2261 w2273]
          tunnel: [w2258 w2272] -> w2256
          frame "Red", Default {
            n894 = Multiply(x=0.5, y=8333.33) -> (x*y=w2263:dbl)
            n895 = To Long Integer(number=w2263) -> (32bit integer=w2268:i32)
            n896 = Number To Decimal String(number=600) -> (decimal integer string=w2266:string)  [unwired: 1 in]
            n897 = Build Array(w2266) -> (w2264:string[])
            n898 = call "gsp_silvermax_writeregister.vi"("Register Value"=w2268, "Motor #"=u8 40, "Register# (0)"=u8 5) -> ("Motor # dup"=w2259:u8)  [unwired: 3 in, 1 out]
            n899 = call "gsp_silvermax_commandreponse.vi"("error in (no error)"=w2261, "Parameters (none)"=w2264, "Motor #"=w2259, "Command"=T9."LRP (156)") -> ("error out"=w2258:errorcluster)  [unwired: 3 out]
          }
          frame "Blue" {
            n900 = Multiply(x=0.5, y=8333.33) -> (x*y=w2275:dbl)
            n901 = To Long Integer(number=w2275) -> (32bit integer=w2281:i32)
            n902 = Number To Decimal String(number=450) -> (decimal integer string=w2278:string)  [unwired: 1 in]
            n903 = Build Array(w2278) -> (w2276:string[])
            n904 = call "gsp_silvermax_writeregister.vi"("Register Value"=w2281, "Motor #"=u8 40, "Register# (0)"=u8 5) -> ("Motor # dup"=w2279:u8)  [unwired: 3 in, 1 out]
            n905 = call "gsp_silvermax_commandreponse.vi"("error in (no error)"=w2273, "Parameters (none)"=w2276, "Motor #"=w2279, "Command"=T9."LRP (156)") -> ("error out"=w2272:errorcluster)  [unwired: 3 out]
          }
        }
      }
      frame "SEND_IMAGE" {
        n906 = local read "Current File Name"() -> (w2289:string)
        n907 = Unbundle By Name(w2285) -> ("Other Info..OBSTYPE"=w2284:string)
        n908 = call "Send Single TCP-IP Cmd 1.vi"("TCP/IP ID"=w2295, "Camera Color"=w2294, "Error In"=w2291, "Function #"=u16 1031, "File Name"=w2289, "Camera ID"=u8 0, "Save As"=w2290) -> ("Error Out"=w2287:errorcluster)  [unwired: 9 in, 3 out]
        n909 = case shown="\"\", Default" w2284 {
          frame "", Default {
            n910 = local write "Focus Changed?"(TRUE) -> ()
          }
          frame "FOCUS" {
            n911 = local write "Focus Changed?"(FALSE) -> ()
          }
        }
        n912 = case shown="False" "Show Images?" {
          tunnel: w2289 -> [_ w2298]
          frame False {
          }
          frame True {
            n913 = Obtain Queue(name (unnamed)="QUICKLOOK_Q", element data type=T7 {"Command"="", "Parameter"=""} ("element")) -> (queue out=w2303:refnum<queue>)  [unwired: 3 in, 2 out]
            n914 = Bundle("Command"="OPEN_FITS_FILE", "Current File Name"=w2298) -> (w2300:T27)  [unwired: 1 in]
            n915 = Enqueue Element(queue=w2303, element=w2300) -> (queue out=w2299:refnum<queue>)  [unwired: 2 in, 2 out]
            n916 = Release Queue(queue=w2299) -> ()  [unwired: 2 in, 3 out]
          }
        }
        n917 = property on="Readout left" class="DigNum (strict)"("Visible"=FALSE) -> ()  [unwired: 2 in, 2 out]
      }
      frame "MULTISLIT" {
        n918 = case shown="True" "MOS" {
          frame False {
          }
          frame True {
            n919 = local read "Current File Name"() -> (w2307:string)
            n920 = Obtain Queue(name (unnamed)="MULTISLIT_Q", element data type=T7 {"Command"="", "Parameter"=""} ("element")) -> (queue out=w2312:refnum<queue>)  [unwired: 3 in, 2 out]
            n921 = Bundle("Command"="OPEN_FITS_FILE", "Current File Name"=w2307) -> (w2309:T27)  [unwired: 1 in]
            n922 = Enqueue Element(queue=w2312, element=w2309) -> (queue out=w2308:refnum<queue>)  [unwired: 2 in, 2 out]
            n923 = Release Queue(queue=w2308) -> ()  [unwired: 2 in, 3 out]
          }
        }
      }
      frame "END_SCRIPT" {
        # "Check for success of acquisition"
        n924 = property on="Take Thumbnail" class="Bool (strict)"() -> ("Value"=w2319:bool)  [unwired: 2 in, 2 out]
        n925 = local read "Mode"() -> (w2325:u16)
        n926 = local read "Acq Mode"() -> (w2326:T5)
        n927 = case shown="True" w2319 {
          tunnel: w2320 -> [w2328 w2334]
          tunnel: [w2328 w2334] -> w2317
          tunnel: w2316 -> [_ w2331]
          tunnel: w2314 -> [_ w2329]
          frame False {
          }
          frame True {
            n928 = local write "Mode"(4) -> ()
            n929 = local read "CCD ROI"() -> (w2330:cluster{i32, i32, i32, i32, i32, i32})
            n930 = property on="Take Thumbnail" class="Bool (strict)"("Value"=FALSE ("Take Thumbnail")) -> ()  [unwired: 2 in, 2 out]
            n931 = call "Send Single TCP-IP Cmd 1.vi"("TCP/IP ID"=w2331, "Camera Color"=w2329, "Function #"=u16 1043, "Camera ID"=u8 1, "CCD Format Parameters"=w2330) -> ("Error Out"=w2335:errorcluster)  [unwired: 11 in, 3 out]
            n932 = call "SI Image Error Handler - Win 2.vi"("error in (no error)"=w2335) -> ()  [unwired: 4 in, 1 out]
          }
        }
        n933 = property on="Start Exposure" class="Bool (strict)"(error in=w2317, "Value"=FALSE ("Start Exposure")) -> (error out=w2321:errorcluster)  [unwired: 1 in, 1 out]
        n934 = property on="Readout" class="Slide (strict)"(error in=w2321, "Caption.Text"="% Readout") -> (error out=w2318:errorcluster)  [unwired: 1 in, 1 out]
        n935 = case shown="1, Default" w2325 {
          selector: w2325 -> [w2340 w2343 w2369]
          tunnel: w2316 -> [_ w2342 _]
          tunnel: [w2340 w2343 w2369] -> w2327
          tunnel: w2326 -> [_ w2348 _]
          tunnel: [w2339 w2345 w2368] -> w2315
          tunnel: w2318 -> [w2339 w2344 w2368]
          tunnel: w2314 -> [_ w2341 _]
          frame 0 {
          }
          frame 1, Default {
            # "If Exposure was not 100%, acquisition was terminated so send TerminateAcquisition command."
            n936 = Equal?(x=w2348, y=Client_Acquisition_Mode_Menu."Average Images") -> (x = y?=w2346:bool)
            n937 = local read "# to Average"() -> (w2352:u32)
            n938 = local read "Exposure"() -> (w2355:u16)
            n939 = local read "Acquiring"() -> (w2353:u32)
            n940 = Less?(x=w2353, y=w2352) -> (x < y?=w2351:bool)
            n941 = Less?(x=w2355, y=u16 100) -> (x < y?=w2350:bool)
            n942 = Select(t=w2351, s=w2346, f=w2350) -> (s? t:f=w2349:bool)
            n943 = case shown="True" w2349 {
              tunnel: w2342 -> [_ w2366]
              tunnel: [w2356 w2358] -> w2345
              tunnel: w2344 -> [w2356 _]
              tunnel: w2341 -> [_ w2357]
              frame False {
              }
              frame True {
                n944 = call "Create Command Packet 3_red.vi"("Function #"=u16 1018, "Camera ID (1)"=u8 1 ("Camera ID"), "Camera Color"=w2357) -> ("Cmd Packet"=w2364:string)  [unwired: 12 in]
                n945 = call "Flush TCP-IP Input Buffer.vi"("TCP/IP ID"=w2366) -> ("TCP/IP ID Out"=w2360:refnum<k5>)  [unwired: 4 in]
                n946 = TCP Write(connection ID=w2360, data in=w2364) -> (error out=w2363:errorcluster)  [unwired: 2 in, 2 out]
                n947 = call "Parse TCP-IP Response 4_RED.vi"("TCP/IP ID"=w2360, "error in (no error)"=w2363) -> ("Packet Error Code"=→"Packet\nError code":i32, "Command Done"=w2362:cluster{"Function #":u16}, "error out"=w2358:errorcluster)  [unwired: 3 in, 8 out]
                n948 = Unbundle By Name(w2362) -> ("Function #"=→"Function #":u16)
              }
            }
          }
          frame 5 {
          }
        }
        n949 = stacked-sequence {
          tunnel: w2327 -> [_]
          frame #0 {
            w2338 = u16 0 ("% Exposure")
            n950 = local write "Exposure"(w2338) -> ()
            n951 = local write "Readout"(w2338) -> ()
            "Acquiring" <- w2338
          }
        }
        n952 = local write "Current Status"("Finalizing acquisition..." ("Current Status")) -> ()
      }
      frame "ENABLE_CONTROLS" {
        w2375 = u8 0 ("Disabled")
        n953 = Obtain Queue(name (unnamed)="Coll_Command_Q", element data type=T7 {"Command"="", "Parameter"=""} ("Command")) -> (queue out=w2370:refnum<queue>)  [unwired: 3 in, 2 out]
        n954 = property on="Acq Mode" class="Enum (strict)"("Disabled"=w2375) -> ()  [unwired: 2 in, 2 out]
        n955 = property on="Save As" class="Ring (strict)"("Disabled"=w2375) -> ()  [unwired: 2 in, 2 out]
        n956 = property on="Image #" class="DigNum (strict)"("Disabled"=w2375) -> ()  [unwired: 2 in, 2 out]
        n957 = property on="Thumbnail Setting" class="Enum (strict)"("Disabled"=w2375) -> ()  [unwired: 2 in, 2 out]
        n958 = property on="Get Camera Status" class="Bool (strict)"("Disabled"=w2375) -> ()  [unwired: 2 in, 2 out]
        n959 = property on="Exp. Time (s)" class="DigNum (strict)"("Disabled"=w2375) -> ()  [unwired: 2 in, 2 out]
        n960 = property on="File Name Base" class="Str"("Disabled"=w2375) -> ()  [unwired: 2 in, 2 out]
        n961 = property on="Exposure Tab" class="TabCtl (strict)"("Disabled"=w2375) -> ()  [unwired: 2 in, 2 out]
        n962 = property on="Take Thumbnail" class="Bool (strict)"("Disabled"=w2375) -> ()  [unwired: 2 in, 2 out]
        n963 = property on="Start Exposure" class="Bool (strict)"("Disabled"=w2375) -> ()  [unwired: 2 in, 2 out]
        n964 = property on="CCD ROI Mode" class="Ring (strict)"("Disabled"=w2375) -> ()  [unwired: 2 in, 2 out]
        n965 = Enqueue Element(queue=w2370, element=T7 {"Command"="ENABLE", "Parameter"=""}) -> (queue out=w2371:refnum<queue>)  [unwired: 2 in, 2 out]
        n966 = Release Queue(queue=w2371) -> ()  [unwired: 2 in, 3 out]
        n967 = property on="Port Readout" class="Ring (strict)"("Disabled"=w2375) -> ()  [unwired: 2 in, 2 out]
        n968 = property on="CCD Readout Speed" class="Ring (strict)"("Disabled"=w2375) -> ()  [unwired: 2 in, 2 out]
        n969 = property on="Systems Status & Control" class="TabCtl (strict)"("Disabled"=w2375) -> ()  [unwired: 2 in, 2 out]
      }
      frame "ERROR" {
        n970 = local read "Camera Errors"() -> (w2384:errorcluster)
        n971 = Bundle By Name(cluster=T12 {"error in (no error)"={"status"=FALSE, "code"=0, "source"=""}, "Source"="", "Comment "=""} ("Log"), "error in (no error)"=w2384, "Source"="SIcamera Control Module") -> (w2381:T12)
        n972 = call "GSP_Logger_Handler.vi"("Log"=w2381, "Actions"=T13."Log") -> ()  [unwired: 5 in, 1 out]
        n973 = Unbundle By Name(w2384) -> ("code"=w2383:i32)
        n974 = case shown="0, Default" w2383 {
          tunnel: w2384 -> [_ w2393]
          tunnel: [errorcluster {"status"=FALSE, "code"=0, "source"=""} ("last_camera_error") w2393] -> w2385
          tunnel: w2378 -> [w2389 w2392]
          tunnel: [w2389 w2392] -> w2377
          frame 0, Default {
            n975 = global write "Apogee_Global.vi" "Camera State"(CameraStates."Error" ("Camera State")) -> ()
          }
          frame 56 {
          }
        }
        n976 = case shown="No Error" w2385 {
          tunnel: w2377 -> [_ w2387]
          frame No Error {
          }
          frame Error {
            n977 = Enqueue Element At Opposite End(queue=w2387, element=T7 {"Command"="SHUTDOWN", "Parameter"=""}) -> ()  [unwired: 2 in, 3 out]
          }
        }
      }
      frame "SHUTDOWN" {
        n978 = Release Queue(queue=w2408) -> ()  [unwired: 2 in, 3 out]
        n979 = Release Queue(queue=w2409) -> ()  [unwired: 2 in, 3 out]
        n980 = Release Queue(queue=w2416, error in (no error)=w2415) -> (error out=w2413:errorcluster)  [unwired: 1 in, 2 out]
        n981 = TCP Close Connection(connection ID=w2410, error in (no error)=w2413) -> (error out=w2412:errorcluster)  [unwired: 1 in, 1 out]
        n982 = Obtain Queue(name (unnamed)="MULTISLIT_Q", element data type=T7 {"Command"="", "Parameter"=""} ("element")) -> (queue out=w2400:refnum<queue>, error out=w2399:errorcluster)  [unwired: 3 in, 1 out]
        n983 = Obtain Queue(name (unnamed)="QUICKLOOK_Q", element data type=T7 {"Command"="", "Parameter"=""} ("element")) -> (queue out=w2407:refnum<queue>, error out=w2406:errorcluster)  [unwired: 3 in, 1 out]
        n984 = Enqueue Element(queue=w2400, element=T7 {"Command"="SHUTDOWN", "Parameter"=""}, error in (no error)=w2399) -> (queue out=w2397:refnum<queue>, error out=w2396:errorcluster)  [unwired: 1 in, 1 out]
        n985 = Enqueue Element(queue=w2407, element=T7 {"Command"="SHUTDOWN", "Parameter"=""}, error in (no error)=w2406) -> (queue out=w2404:refnum<queue>, error out=w2403:errorcluster)  [unwired: 1 in, 1 out]
        n986 = Release Queue(queue=w2397, error in (no error)=w2396) -> ()  [unwired: 1 in, 3 out]
        n987 = Release Queue(queue=w2404, error in (no error)=w2403) -> ()  [unwired: 1 in, 3 out]
        n988 = local write "Connection Status"(FALSE ("Connection Status")) -> ()
        n989 = local write "Current Status"("Shutting down..." ("Current Status")) -> ()
      }
    }
    n990 = Equal?(x=w36, y="SHUTDOWN") -> (x = y?=w37:bool)
    n991 = case shown="Error" w38 {
      selector: w38 -> [_ w46]
      tunnel: w39 -> [_ w48]
      frame No Error {
      }
      frame Error {
        n992 = Enqueue Element At Opposite End(queue=w48, element=T7 {"Command"="ERROR", "Parameter"=""}) -> ()  [unwired: 2 in, 3 out]
        "Camera Errors" <- w46
      }
    }
  }
